vi "New Cobra GUI.vi"(8 "error in":errorcluster) -> (0 "Error Out":errorcluster)   [LabVIEW 2019, in "GUI.lvlib"]
doc: "New GUI 21.7.19"
uses:
  GUI.lvlib
  Controls/Main Waveform.ctl
  Controls/System Graphs.ctl
  Controls/Module Graphs.ctl
  Controls/Dial Gauges.ctl
  Controls/Gauge Graphs/Compression Ratio.ctl
  Controls/Gauge Graphs/Subcooling.ctl
  Controls/Gauge Graphs/Superheat.ctl
  Controls/Gauge Graphs/Current.ctl
  Controls/Module Key Values.ctl
  Controls/Event.ctl
  Controls/Messaging Actions.ctl
  Controls/New GUI Variables.ctl
  Controls/Network Data Down_set back.ctl
  Controls/NS New Data.ctl
  <vilib>/NI/STM/TCP/TCP Connection Info.ctl
  <vilib>/NI/STM/SubVIs/MetaDataElement.ctl
  Controls/Dataset_New.ctl
  Controls/System Status.ctl
  Controls/Module Status.ctl
  Controls/Config Data.ctl
  <vilib>/Utility/miscctls.llb/LVPositionTypeDef.ctl
  <vilib>/NI/STM/TCP/TCP Read Options.ctl
  Controls/WebDAV states.ctl
  <vilib>/Analysis/baseanly.llb/Mean (DBL).vi
  b9938fbe-5ccd-4e62-98e3-88d978d07e59.vi
  795e1a79-78c9-4e5b-9a6d-4827452a9509.vi
  894b418a-eb83-4c03-97c2-0273c02a970a.vi
  81edff22-585a-4beb-bf15-c06a681b6c24.vi
  <vilib>/NI/STM/TCP/Read Meta Data (TCP Ref).vi
  <vilib>/NI/STM/TCP/Get Connection Reference (TCP).vi
  <vilib>/NI/STM/TCP/Read Meta Data (TCP Clst).vi
  <vilib>/NI/STM/TCP/Read Message (TCP).vi
  <vilib>/NI/STM/TCP/Write Message (TCP).vi
  <vilib>/regexp/Match Regular Expression.xnode
  <vilib>/nisyscfg/nisyscfg.lvlib
  <resource>/objmgr/ni.dex.rc
  Controls/Save Log State.ctl
  <vilib>/Analysis/NI_AALBase.lvlib
  <vilib>/NI/STM/NI STM.lvlib
  <vilib>/addons/_JKI.lib/Serialization/JSON/JKI JSON Serialization.lvlib
panel:
  in  "Login":bool
  out "RT Version":string="Simulation Mode" caption="Cobra GUI Version :"
  in  "Shutdown":bool caption="Stop RT"
  in  "M1 Feedback":u8(ring)=1 caption="Enable" items=["Evap Temp", "Case Temp", "Intec Temp", "TSD  Temp", "Autotune", "Extra"]
  in  "M2 Feedback":u8(ring)=1 caption="Enable" items=["Evap Temp", "Case Temp", "Intec Temp", "TSD  Temp", "Autotune", "Extra"]
  out "M2 Data":T1={"Set Temp"=20.0, "Read Temp"=0.0, "Package"="", "Force"=0.0, "Feedback"=1} caption="M2 Status" {"Feedback" items=["Evap Temp", "Case Temp", "Intec Temp", "TSD  Temp", "Autotune", "Extra"]; "Force" format="%4.1f"; "Read Temp" format="%4.1f"; "Set Temp" format="%4.0f"}
  out "M1 Data":T1={"Set Temp"=25.0, "Read Temp"=24.578125, "Package"="new_chip", "Force"=0.0, "Feedback"=1} caption="M1 Status" {"Feedback" items=["Evap Temp", "Case Temp", "Intec Temp", "TSD  Temp", "Autotune", "Extra"]; "Force" format="%4.1f"; "Read Temp" format="%4.1f"; "Set Temp" format="%4.0f"}
  out "Comp":bool caption="System"
  out "Stack light states":T2(ring) caption="System Status"
  in  "Change TSD":bool
  out "TSD Data":T3={"TSD Millivolts"=nan, "X factor"=1.0, "Offset"=0.0, "TSD Temp"=nan, "TSD Feedback"=FALSE, "TSD Max"=225.0, "TSD Min"=-60.0}
  out "M1 AC Load V":dbl
  in  "Net Cluster":T4={"Menu Ring"=0, "System Ready"=TRUE, "Manual IP"="", "Refresh"=FALSE, "IP Override"=FALSE} {"Menu Ring" items=["DualCobra152 (192.168.2.52)", "Gen3Cobra146 (192.168.2.46)", "QC-Test (192.168.1.57)"]}
  out "AI (V)":dbl[](array[numeric])=[0.0, 0.0, 0.0, 0.0, 0.0, 0.0, 0.0, 0.0, 0.0, 0.0, 5.0, 5.0, 1625.0, 0.0, 0.0, 0.0, 0.0, 0.0, 0.0]
  out "data out":T5={"Condensing Pressure"=153.40193026626991, "Suction Pressure"=154.74626335545852, "Bypass steps"=0, "Operating Time"=0.0, "SubCooling"=-2.934594678017916, "Superheat"=3.7527707418295932, "M1 Superheat"=3.162141007730682, "M2 Superheat"=-40.92379649226932, "Autotune output"=0.0, "M1 Testing Elapsed Time"=0.0, "M2 Testing Elapsed Time"=0.0, "M1 Valve Control Mode"=0, "System Amps"=0.1457709610825283, "Compressor Run Time"=0.0, "SD card free Space"=31890.0, "Free Memory"=0.0, "M1 Pressure Feedback"=0.0, "M2 Pressure Feedback"=0.0, "Compression Ratio"=0.9920663161136312, "Serial Number"=0.0, "M1 AC Load V"=0.0, "M1 AC Load W"=nan, "M1 DC Load W"=0.0, "M1 RH"=33.76176771953824, "RH Threshold"=10.0}
  in  "Tab Control":T6(tab)=enum."Debug"
  out "M2 Safe Temp and Head State":bool
  out "M2 Bin String":string
  out "M2 PV":dbl caption="M2 Case Temp" format="%4.1f"
  in  "M2 Package":u16(ring)=4 items=["new_chip", "AI_chip", "CPU", "GPU", "Max Force", "", "", "", "", ""]
  in  "M2 Set Temp":dbl=20.0 min=-50.0 max=150.0 step=5.0 format="%#.1f"
  in  "M2 Commands Panel":T7={"M2 Enable"=TRUE, "M2 TSD Feedback"=FALSE}
  out "M1 Bin String":string
  in  "M1 Set Temp":dbl=25.0 min=-50.0 max=150.0 step=5.0 format="%#.1f"
  in  "M1 Package":u16(ring) items=["new_chip", "AI_chip", "CPU", "GPU", "Max Force", "", "", "", "", ""]
  out "M1 PV":dbl=24.578125 caption="M1 Case Temp" format="%4.1f"
  in  "M1 Commands Panel":T8={"M1 Enable"=TRUE, "M1 TSD Feedback"=FALSE}
  out "M1 Safe Temp and Head State":bool
  in  "M2 Power Drive Control":bool
  out "M1 Main Waveform":T9=[{"t0"=timestamp(3706115941.7064414 s since 1904-01-01), "dt"=1.0, "Y"=[25.0]}, {"t0"=timestamp(3706115941.7064414 s since 1904-01-01), "dt"=1.0, "Y"=[24.4453125]}, {"t0"=timestamp(3706115941.7064414 s since 1904-01-01), "dt"=1.0, "Y"=[24.578125]}, {"t0"=timestamp(3706115941.7064414 s since 1904-01-01), "dt"=1.0, "Y"=[nan]}, {"t0"=timestamp(3706115941.7064414 s since 1904-01-01), "dt"=1.0, "Y"=[nan]}]
  in  "M1 Power Drive Control":bool
  out "M2 Power Drive Indicator":bool caption="M2 Power Drive Control"
  out "M1 Power Drive Indicator":bool caption="M1 Power Drive Control"
  in  "Power On-Off":bool
  out "Play/Pause":bool
  out "M2 Main Waveform":T9=[{"t0"=timestamp(3706115941.7064414 s since 1904-01-01), "dt"=1.0, "Y"=[20.0]}, {"t0"=timestamp(3706115941.7064414 s since 1904-01-01), "dt"=1.0, "Y"=[0.0]}, {"t0"=timestamp(3706115941.7064414 s since 1904-01-01), "dt"=1.0, "Y"=[0.0]}, {"t0"=timestamp(3706115941.7064414 s since 1904-01-01), "dt"=1.0, "Y"=[0.0]}]
  out "M1 Channels":dbl[](array[numeric])=[25.0, 24.4453125, 24.578125, nan, nan, 0.0] format="%4.1f"
  out "M2 Channels":dbl[](array[numeric])=[20.0, 0.0, 0.0, 0.0, 0.0] format="%4.1f"
  out "M1 Humidity":cluster{"M1 RH":dbl, "RH Threshold":dbl}(graph)={"M1 RH"=10.0, "RH Threshold"=33.76176771953824}
  out "Low Side RPM":dbl
  out "High Side RPM":dbl
  out "M2 Thermal State":T10(ring)
  out "System Graphs":T11={"Ambient Temp"=75.93125465512276, "Suction Temp"=76.69062973558903, "Condensor Temp"=75.24219208210707, "Discharge Temp"=76.67656723409891, "Bypass Steps"=72.0}
  out "M1 Thermal State":T12(ring)=enum."Steady State"
  out "Gauges":T13={"Condensing Pressure(psi)"=153.40193026626991, "Compression Ratio"=0.9920663161136312, "Subcool"=-3.0617528737987953, "Superheat"=3.6858450233187767, "Current(A)"=0.1457709610825283, "Suction Pressure(psi)"=154.74626335545852} {"Suction Pressure(psi)" scale=0.0..100.0; "Current(A)" scale=5.0..15.0 scale format="%_1f"; "Superheat" scale=0.0..100.0; "Subcool" scale=-10.0..20.0 scale format="%#4.1f"; "Compression Ratio" scale=0.0..30.0 scale format="%#.0f"; "Condensing Pressure(psi)" scale=150.0..375.0}
  in  "Graph Tab CTL":enum32{"Head #1", "Head #2"}(tab)
  out "M1 Graphs":T18={"Case Temp"=24.578125, "Evap Temp"=24.4453125, "Heater Power (%)"=0.0, "EEV Steps"=0.0, "AC Load(W)"=0.0} caption="Head #1"
  out "M2 Graphs":T18 caption="Head #2"
  in  "Package":bool
  in  "Configure":bool
  out "Errors":string[](array[string])=["Warning: Air not plugged in  (21 06 08 14 08)"]
  in  "Event Tab":enum32{"Cobra Events", "GUI Events"}(tab)
  out "Event log":T19(array[cluster])=[{"Name"="Bypass Inintialized", "Time Stamp"=timestamp(3706031317.901618 s since 1904-01-01), "Code"="", "Source"="", "Value"=22160.0, "Boolean"=FALSE, "String"="Complete", "Error"=FALSE, "Warning"=FALSE, " Fault"=FALSE}, {"Name"="Timeserver not found", "Time Stamp"=timestamp(3706031309.741007 s since 1904-01-01), "Code"="", "Source"="SOM Time", "Value"=0.0, "Boolean"=FALSE, "String"="", "Error"=FALSE, "Warning"=FALSE, " Fault"=FALSE}, {"Name"="Bypass Target Change", "Time Stamp"=timestamp(3706031309.711301 s since 1904-01-01), "Code"="", "Source"="Bypass:Get Target", "Value"=110.0, "Boolean"=FALSE, "String"="", "Error"=FALSE, "Warning"=TRUE, " Fault"=FALSE}, {"Name"="Mains Frequency", "Time Stamp"=timestamp(3706031309.198055 s since 1904-01-01), "Code"="", "Source"="Init System Module", "Value"=59.9940002520096, "Boolean"=FALSE, "String"="", "Error"=FALSE, "Warning"=FALSE, " Fault"=FALSE}, {"Name"="PID Bypassed", "Time Stamp"=timestamp(3706031307.313306 s since 1904-01-01), "Code"="", "Source"="APP:Set/Send PID Bypass", "Value"=0.0, "Boolean"=FALSE, "String"="", "Error"=FALSE, "Warning"=FALSE, " Fault"=FALSE}, {"Name"="Thermal Status Change", "Time Stamp"=timestamp(3706031307.007236 s since 1904-01-01), "Code"="", "Source"="APP:Thermal Status", "Value"=0.0, "Boolean"=FALSE, "String"="", "Error"=FALSE, "Warning"=FALSE, " Fault"=FALSE}, {"Name"="Feedback Change", "Time Stamp"=timestamp(3706031306.793005 s since 1904-01-01), "Code"="", "Source"="APP:Get Feedback", "Value"=1.0, "Boolean"=FALSE, "String"="Case", "Error"=FALSE, "Warning"=FALSE, " Fault"=FALSE}, {"Name"="M1 Setpoint Change", "Time Stamp"=timestamp(3706031306.436291 s since 1904-01-01), "Code"="", "Source"="APP:Send Set Temp", "Value"=25.0, "Boolean"=FALSE, "String"="", "Error"=FALSE, "Warning"=TRUE, " Fault"=FALSE}, {"Name"="M1 Dynamic Set Point", "Time Stamp"=timestamp(3706031306.386277 s since 1904-01-01), "Code"="", "Source"="APP:Get Dynamic Set Temp", "Value"=25.0, "Boolean"=FALSE, "String"="", "Error"=FALSE, "Warning"=FALSE, " Fault"=FALSE}, {"Name"="M1 EEV Check Position", "Time Stamp"=timestamp(3706031306.325976 s since 1904-01-01), "Code"="", "Source"="", "Value"=0.0, "Boolean"=TRUE, "String"="Complete", "Error"=FALSE, "Warning"=FALSE, " Fault"=FALSE}, {"Name"="I2C TSD Freeze Timeout", "Time Stamp"=timestamp(3706031300.268274 s since 1904-01-01), "Code"="", "Source"="", "Value"=0.0, "Boolean"=FALSE, "String"="", "Error"=TRUE, "Warning"=FALSE, " Fault"=FALSE}, {"Name"="New Extra Settings Loaded", "Time Stamp"=timestamp(3706031298.435066 s since 1904-01-01), "Code"="", "Source"="", "Value"=0.0, "Boolean"=FALSE, "String"="", "Error"=FALSE, "Warning"=FALSE, " Fault"=FALSE}, {"Name"="Read Compressor Minutes", "Time Stamp"=timestamp(3706031298.210019 s since 1904-01-01), "Code"="", "Source"="", "Value"=0.0, "Boolean"=TRUE, "String"="PASS", "Error"=FALSE, "Warning"=FALSE, " Fault"=FALSE}, {"Name"="M1 EEV Check Position", "Time Stamp"=timestamp(3706031296.21211 s since 1904-01-01), "Code"="", "Source"="EEV:Check Position", "Value"=0.0, "Boolean"=FALSE, "String"="", "Error"=FALSE, "Warning"=FALSE, " Fault"=FALSE}, {"Name"="EEV PID Output", "Time Stamp"=timestamp(3706031296.161288 s since 1904-01-01), "Code"="", "Source"="APP:Send EEV PID Out", "Value"=0.0, "Boolean"=FALSE, "String"="Value Change", "Error"=FALSE, "Warning"=FALSE, " Fault"=FALSE}, {"Name"="", "Time Stamp"=timestamp(3706031296.053791 s since 1904-01-01), "Code"="", "Source"="EEV:Set Position", "Value"=0.0, "Boolean"=FALSE, "String"="", "Error"=FALSE, "Warning"=FALSE, " Fault"=FALSE}, {"Name"="", "Time Stamp"=timestamp(3706031296.000374 s since 1904-01-01), "Code"="", "Source"="EEV:Config", "Value"=0.0, "Boolean"=FALSE, "String"="", "Error"=FALSE, "Warning"=FALSE, " Fault"=FALSE}, {"Name"="M1 EEV Check Position", "Time Stamp"=timestamp(3706031294.611185 s since 1904-01-01), "Code"="", "Source"="", "Value"=2000.0, "Boolean"=TRUE, "String"="Complete", "Error"=FALSE, "Warning"=FALSE, " Fault"=FALSE}, {"Name"="M1 EEV Check Position", "Time Stamp"=timestamp(3706031294.000098 s since 1904-01-01), "Code"="", "Source"="EEV:Check Position", "Value"=0.0, "Boolean"=FALSE, "String"="", "Error"=FALSE, "Warning"=FALSE, " Fault"=FALSE}, {"Name"="EEV PID Output", "Time Stamp"=timestamp(3706031293.949764 s since 1904-01-01), "Code"="", "Source"="APP:Send EEV PID Out", "Value"=2000.0, "Boolean"=FALSE, "String"="Value Change", "Error"=FALSE, "Warning"=FALSE, " Fault"=FALSE}, {"Name"="", "Time Stamp"=timestamp(3706031293.848812 s since 1904-01-01), "Code"="", "Source"="EEV:Set Position", "Value"=0.0, "Boolean"=TRUE, "String"="", "Error"=FALSE, "Warning"=FALSE, " Fault"=FALSE}, {"Name"="EEV:Set V", "Time Stamp"=timestamp(3706031293.798386 s since 1904-01-01), "Code"="", "Source"="", "Value"=0.0, "Boolean"=FALSE, "String"="", "Error"=FALSE, "Warning"=FALSE, " Fault"=FALSE}, {"Name"="", "Time Stamp"=timestamp(3706031293.748195 s since 1904-01-01), "Code"="", "Source"="EEV:Config", "Value"=0.0, "Boolean"=FALSE, "String"="", "Error"=FALSE, "Warning"=FALSE, " Fault"=FALSE}, {"Name"="Config Loaded", "Time Stamp"=timestamp(3706031293.397414 s since 1904-01-01), "Code"="", "Source"="Config Read Initialize", "Value"=107.0, "Boolean"=FALSE, "String"="", "Error"=FALSE, "Warning"=FALSE, " Fault"=FALSE}, {"Name"="Config Read", "Time Stamp"=timestamp(3706031293.37065 s since 1904-01-01), "Code"="Found", "Source"="EEV PID", "Value"=25.0, "Boolean"=FALSE, "String"="", "Error"=FALSE, "Warning"=FALSE, " Fault"=FALSE}, {"Name"="Config Read", "Time Stamp"=timestamp(3706031293.359371 s since 1904-01-01), "Code"="Found", "Source"="Set Point Range", "Value"=-50.0, "Boolean"=FALSE, "String"="", "Error"=FALSE, "Warning"=FALSE, " Fault"=FALSE}, {"Name"="Config Value Read", "Time Stamp"=timestamp(3706031293.335439 s since 1904-01-01), "Code"="", "Source"="", "Value"=0.0, "Boolean"=TRUE, "String"="Cascade", "Error"=FALSE, "Warning"=FALSE, " Fault"=FALSE}, {"Name"="Config Value Read", "Time Stamp"=timestamp(3706031293.315639 s since 1904-01-01), "Code"="", "Source"="", "Value"=0.0, "Boolean"=TRUE, "String"="Sensors", "Error"=FALSE, "Warning"=FALSE, " Fault"=FALSE}, {"Name"="Read Saved State", "Time Stamp"=timestamp(3706031293.26891 s since 1904-01-01), "Code"="", "Source"="", "Value"=0.0, "Boolean"=FALSE, "String"="", "Error"=FALSE, "Warning"=FALSE, " Fault"=FALSE}, {"Name"="EMO Switch Detected", "Time Stamp"=timestamp(3706031293.21723 s since 1904-01-01), "Code"="", "Source"="", "Value"=0.0, "Boolean"=TRUE, "String"="", "Error"=FALSE, "Warning"=FALSE, " Fault"=FALSE}, {"Name"="Read Saved State", "Time Stamp"=timestamp(3706031293.183574 s since 1904-01-01), "Code"="", "Source"="", "Value"=0.0, "Boolean"=FALSE, "String"="", "Error"=FALSE, "Warning"=FALSE, " Fault"=FALSE}, {"Name"="FPGA Load Complete", "Time Stamp"=timestamp(3706031293.139812 s since 1904-01-01), "Code"="", "Source"="Init FPGA IO.vi", "Value"=0.0, "Boolean"=FALSE, "String"="", "Error"=FALSE, "Warning"=FALSE, " Fault"=FALSE}, {"Name"="Pressure Test", "Time Stamp"=timestamp(3706031291.136962 s since 1904-01-01), "Code"="", "Source"="Init FPGA IO 2.0.vi", "Value"=0.00022888532845044633, "Boolean"=FALSE, "String"="FAIL", "Error"=FALSE, "Warning"=TRUE, " Fault"=FALSE}, {"Name"="Stop LCD", "Time Stamp"=timestamp(3706031285.92111 s since 1904-01-01), "Code"="", "Source"="Init FPGA IO.vi", "Value"=11.0, "Boolean"=FALSE, "String"="", "Error"=FALSE, "Warning"=FALSE, " Fault"=FALSE}, {"Name"="wait", "Time Stamp"=timestamp(3706031284.919174 s since 1904-01-01), "Code"="", "Source"="Init FPGA IO.vi", "Value"=10.0, "Boolean"=FALSE, "String"="", "Error"=FALSE, "Warning"=FALSE, " Fault"=FALSE}, {"Name"="IP Address", "Time Stamp"=timestamp(3706031283.915648 s since 1904-01-01), "Code"="", "Source"="Init FPGA IO.vi", "Value"=12.0, "Boolean"=FALSE, "String"="þQ", "Error"=FALSE, "Warning"=FALSE, " Fault"=FALSE}, {"Name"="wait", "Time Stamp"=timestamp(3706031283.836404 s since 1904-01-01), "Code"="", "Source"="Init FPGA IO.vi", "Value"=10.0, "Boolean"=FALSE, "String"="", "Error"=FALSE, "Warning"=FALSE, " Fault"=FALSE}, {"Name"="Rev Display", "Time Stamp"=timestamp(3706031282.833974 s since 1904-01-01), "Code"="", "Source"="Init FPGA IO.vi", "Value"=9.0, "Boolean"=FALSE, "String"="Ver: CC 21.6.1.0", "Error"=FALSE, "Warning"=FALSE, " Fault"=FALSE}, {"Name"="wait", "Time Stamp"=timestamp(3706031282.765893 s since 1904-01-01), "Code"="", "Source"="Init FPGA IO.vi", "Value"=10.0, "Boolean"=FALSE, "String"="", "Error"=FALSE, "Warning"=FALSE, " Fault"=FALSE}, {"Name"="Chroma Display", "Time Stamp"=timestamp(3706031281.763213 s since 1904-01-01), "Code"="", "Source"="Init FPGA IO.vi", "Value"=8.0, "Boolean"=FALSE, "String"="Chroma ATE", "Error"=FALSE, "Warning"=FALSE, " Fault"=FALSE}, {"Name"="wait", "Time Stamp"=timestamp(3706031281.696552 s since 1904-01-01), "Code"="", "Source"="Init FPGA IO.vi", "Value"=10.0, "Boolean"=FALSE, "String"="", "Error"=FALSE, "Warning"=FALSE, " Fault"=FALSE}, {"Name"="Clear LCD Text", "Time Stamp"=timestamp(3706031280.693969 s since 1904-01-01), "Code"="", "Source"="Init FPGA IO.vi", "Value"=0.0, "Boolean"=FALSE, "String"="", "Error"=FALSE, "Warning"=FALSE, " Fault"=FALSE}, {"Name"="BootLoad", "Time Stamp"=timestamp(3706031279.648552 s since 1904-01-01), "Code"="", "Source"="Init FPGA IO.vi", "Value"=0.0, "Boolean"=FALSE, "String"="", "Error"=FALSE, "Warning"=FALSE, " Fault"=FALSE}, {"Name"="Extra Settings Loaded", "Time Stamp"=timestamp(3706031277.495041 s since 1904-01-01), "Code"="", "Source"="", "Value"=0.0, "Boolean"=FALSE, "String"="", "Error"=FALSE, "Warning"=FALSE, " Fault"=FALSE}, {"Name"="Warmup ", "Time Stamp"=timestamp(3706031277.461598 s since 1904-01-01), "Code"="", "Source"="Extra Settings", "Value"=0.0, "Boolean"=FALSE, "String"="", "Error"=FALSE, "Warning"=TRUE, " Fault"=FALSE}, {"Name"="Flow Curve", "Time Stamp"=timestamp(3706031277.436586 s since 1904-01-01), "Code"="", "Source"="Extra Settings", "Value"=0.0, "Boolean"=FALSE, "String"="", "Error"=FALSE, "Warning"=TRUE, " Fault"=FALSE}, {"Name"="Relative Humidity", "Time Stamp"=timestamp(3706031277.408702 s since 1904-01-01), "Code"="", "Source"="Extra Settings", "Value"=0.0, "Boolean"=TRUE, "String"="", "Error"=FALSE, "Warning"=FALSE, " Fault"=FALSE}, {"Name"="Warnings/Faults 1", "Time Stamp"=timestamp(3706031277.370367 s since 1904-01-01), "Code"="", "Source"="Extra Settings 3", "Value"=0.0, "Boolean"=TRUE, "String"="", "Error"=FALSE, "Warning"=FALSE, " Fault"=FALSE}, {"Name"="SuperHeat Settings", "Time Stamp"=timestamp(3706031277.356517 s since 1904-01-01), "Code"="", "Source"="Extra Settings 3", "Value"=0.0, "Boolean"=TRUE, "String"="", "Error"=FALSE, "Warning"=FALSE, " Fault"=FALSE}, {"Name"="Config Loaded", "Time Stamp"=timestamp(3706031277.313113 s since 1904-01-01), "Code"="", "Source"="Config Read Initialize", "Value"=74.0, "Boolean"=FALSE, "String"="", "Error"=FALSE, "Warning"=FALSE, " Fault"=FALSE}, {"Name"="Config Read", "Time Stamp"=timestamp(3706031277.287857 s since 1904-01-01), "Code"="Found", "Source"="M2 Heater PID", "Value"=0.0, "Boolean"=FALSE, "String"="", "Error"=FALSE, "Warning"=FALSE, " Fault"=FALSE}, {"Name"="Config Value Read", "Time Stamp"=timestamp(3706031277.269987 s since 1904-01-01), "Code"="", "Source"="", "Value"=0.0, "Boolean"=TRUE, "String"="Handler", "Error"=FALSE, "Warning"=FALSE, " Fault"=FALSE}] {"Value" format="%4.1f"; "Time Stamp" format="%<%x %.3X>T"}
  out "GUI Events":T20[](array[typedef])=[{"Name"="NS:Open Connection", "Time Stamp"=timestamp(3706444762.0143776 s since 1904-01-01), "Code"=-1950678953, "Source"="Create Network Stream Reader Endpoint in GUI.lvlib:New Cobra GUI.vi", "Value"="", "Boolean"=FALSE, "Description"="", "Error"=TRUE, "Warning"=FALSE, " Fault"=FALSE}, {"Name"="NS:Open Connection", "Time Stamp"=timestamp(3706444762.0213585 s since 1904-01-01), "Code"=-1950678953, "Source"="Create Network Stream Reader Endpoint in GUI.lvlib:New Cobra GUI.vi", "Value"="", "Boolean"=FALSE, "Description"="", "Error"=TRUE, "Warning"=FALSE, " Fault"=FALSE}, {"Name"="Idle", "Time Stamp"=timestamp(3706444762.122089 s since 1904-01-01), "Code"=0, "Source"="", "Value"="", "Boolean"=FALSE, "Description"="Start Cobra GUI", "Error"=FALSE, "Warning"=FALSE, " Fault"=FALSE}, {"Name"="UI:Module Enable", "Time Stamp"=timestamp(3706444762.1230865 s since 1904-01-01), "Code"=0, "Source"="", "Value"="", "Boolean"=TRUE, "Description"="System Ready", "Error"=FALSE, "Warning"=FALSE, " Fault"=FALSE}] {"Time Stamp" format="%<%x %.3X>T"}
  in  "Datalog":bool
  in  "Reboot RT":bool
  out "M2 Buffer":dbl(slide)=2.0 scale=-4.0..4.0
  out "M2 Valve Output":dbl(knob) scale=0.0..100.0
  in  "Y-scale":bool
  out "Boot Up Time":timestamp=timestamp(3706031293.185896 s since 1904-01-01)
  out "M2 Heater %":dbl format="%3.0f"
  out "M2 Error":bool
  out "M2 Actuated":bool
  out "M2 Head State":enum16{"Disabled", "Run", "Error"}(ring)=enum."Run"
  out "M2 Thermal Status":T12(ring)
  in  "M2 EEV Manual":u16
  in  "M2 Heater Output":dbl
  in  "M1 EEV Manual":u16
  in  "Manual Bypass Mode":bool[](array[boolean])
  in  "M1 Heater output":dbl
  out "M1 Valve Output":dbl(knob) scale=0.0..100.0
  out "M1 Buffer":dbl(slide) scale=-4.0..4.0
  out "Detected Systems":string[](array[string])
  out "Data Rx Timestamp":timestamp=timestamp(3706107700.479949 s since 1904-01-01)
  out "M1 Superheat":dbl=3.162141007730682 format="%#.1f"
  out "M1 Testing Elapsed Time":dbl caption="Test Elapsed Time" format="%<%H:%M:%S>t"
  out "TCP Connections":T21(array[cluster])=[{"port "=1300, "remote address"="", "Connection timeout ms"=100, "Waiting for connection"=TRUE, "Waiting for Command"=FALSE, "timeout ms"=5000}, {"port "=1100, "remote address"="", "Connection timeout ms"=100, "Waiting for connection"=TRUE, "Waiting for Command"=FALSE, "timeout ms"=-1}, {"port "=1000, "remote address"="", "Connection timeout ms"=100, "Waiting for connection"=TRUE, "Waiting for Command"=FALSE, "timeout ms"=60000}, {"port "=1001, "remote address"="", "Connection timeout ms"=100, "Waiting for connection"=TRUE, "Waiting for Command"=FALSE, "timeout ms"=60000}, {"port "=2100, "remote address"="", "Connection timeout ms"=100, "Waiting for connection"=FALSE, "Waiting for Command"=FALSE, "timeout ms"=-1}, {"port "=2001, "remote address"="", "Connection timeout ms"=100, "Waiting for connection"=FALSE, "Waiting for Command"=FALSE, "timeout ms"=60000}, {"port "=2000, "remote address"="", "Connection timeout ms"=100, "Waiting for connection"=FALSE, "Waiting for Command"=FALSE, "timeout ms"=5000}]
  out "Error":string[](array[string])=["Warning: Air not plugged in  (21 06 08 14 08)"]
  in  "Cascade Compressor controls":T22 {"Manual Low Stage frequency" min=40.0 max=150.0 step=1.0; "Manual High stage frequency" min=50.0 max=150.0 step=1.0}
  out "TCP commands":string[](array[string])
  out "M1 Head State":enum16{"Disabled", "Run", "Error"}(ring)=enum."Run"
  out "M1 Thermal Status":T12(ring)=enum."Steady State"
  out "M1 Error":bool
  out "M1 Actuated":bool
  out "M1 Heater %":dbl format="%3.0f"
  out "Sleep":bool=TRUE
  out "Sleep Timer":dbl
  out "Comp Temp":dbl=76.67656723409891 format="%#.1f"
  out "SOM":T23={"Software Version"="SW Version:CC 21.6.1.0", "CPU Usage"=99.04899711963543, "Memory Available"=317.184, "SOM Storage(MB)"=234.236, "SD card free space"=27.598} caption="System of Module" {"SD card free space" format="%#4.1f"; "CPU Usage" format="%#.1f"; "Memory Available" format="%#4.1f"; "SOM Storage(MB)" format="%4.1f"}
  out "Compressor Hours":dbl caption="Comp hrs" format="%#.1f"
  out "Serial Number":string="203800057"
  in  "Graph Temp Unit":bool
  in  "Average Graph":bool
  in  "Fixed Y-Range":dbl=4.0
  in  "Login TO":i32=10 caption="Login Timeout(min)" min=-1 max=1000
  in  "Real Mode":bool=TRUE
  # "System Module"
  # "M1 Module"
  # "M2 Module"
  # "Tuning"
  # "Manual Controls"
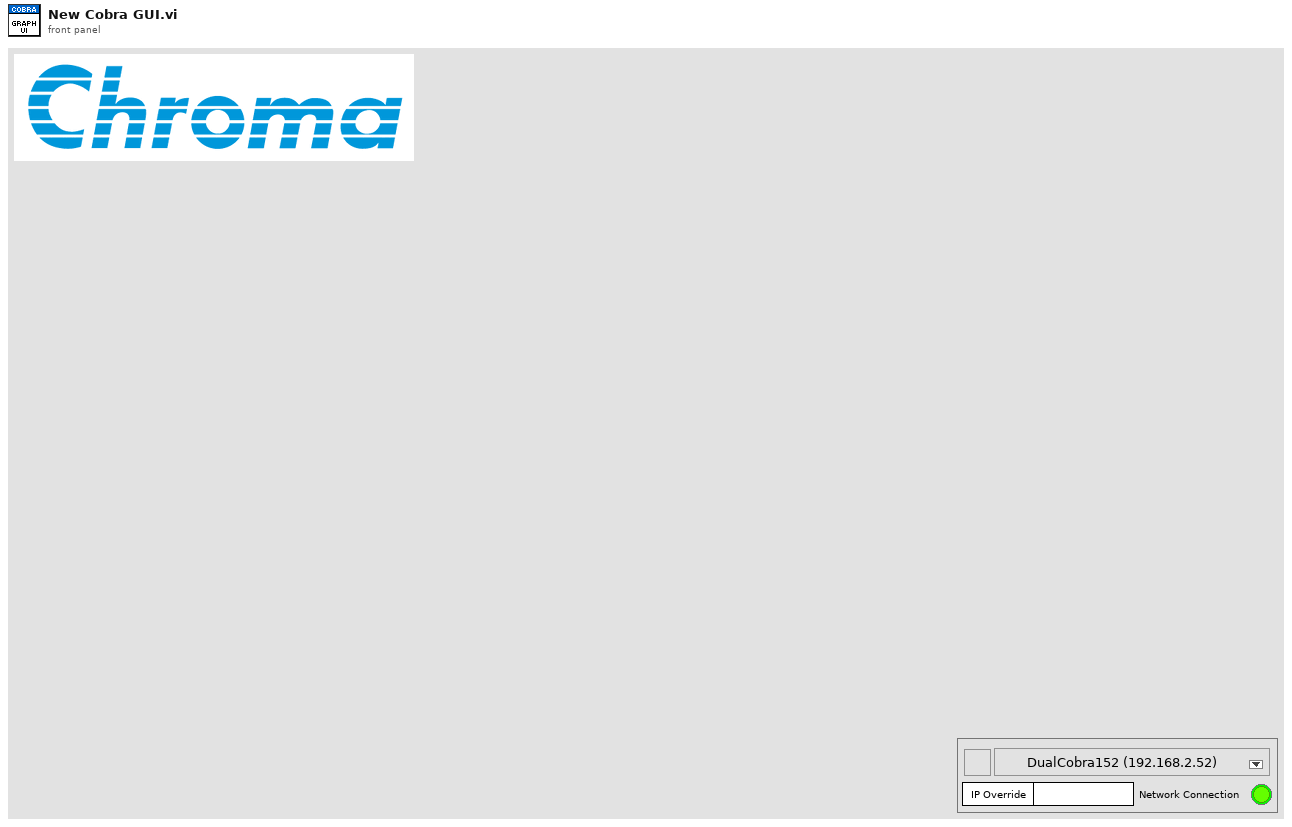
[diagram p1: front panel]
types:
  T1 = typedef "GUI.lvlib/Module Key Values.ctl" = cluster{"Set Temp":dbl, "Read Temp":dbl, "Package":string, "Force":dbl, "Feedback":u8}
  T2 = enum16{"Sleeping", "Warming up", "Ready", "Testing", "Restless", "Idle", "Sleeping Fault", "warning"}
  T3 = cluster{"TSD Millivolts":dbl, "X factor":dbl, "Offset":dbl, "TSD Temp":dbl, "TSD Feedback":bool, "TSD Max":dbl, "TSD Min":dbl}
  T4 = cluster{"Menu Ring":u16, "System Ready":bool, "Manual IP":string, "Refresh":bool, "IP Override":bool}
  T5 = cluster{"Condensing Pressure":dbl, "Suction Pressure":dbl, "Bypass steps":u16, "Operating Time":dbl, "SubCooling":dbl, "Superheat":dbl, "M1 Superheat":dbl, "M2 Superheat":dbl, "Autotune output":dbl, "M1 Testing Elapsed Time":dbl, "M2 Testing Elapsed Time":dbl, "M1 Valve Control Mode":u8, "System Amps":dbl, "Compressor Run Time":dbl, "SD card free Space":dbl, "Free Memory":dbl, "M1 Pressure Feedback":dbl, "M2 Pressure Feedback":dbl, "Compression Ratio":dbl, "Serial Number":dbl, "M1 AC Load V":dbl, "M1 AC Load W":dbl, "M1 DC Load W":dbl, "M1 RH":dbl, "RH Threshold":dbl}
  T6 = enum32{"Controls", "Graphs", "Settings", "Debug", "TEST"}
  T7 = cluster{"M2 Enable":bool, "M2 TSD Feedback":bool}
  T8 = cluster{"M1 Enable":bool, "M1 TSD Feedback":bool}
  T9 = typedef "GUI.lvlib/Main Waveform.ctl" = waveform(dbl)[]
  T10 = enum16{"Ramp Up", "Ramp Down", "Steady State", "Ebb and Flow", "Up", "Under Load", "Cryo Mode", "Shuttle Mode"}
  T11 = typedef "GUI.lvlib/System Graphs.ctl" = cluster{"Ambient Temp":dbl, "Suction Temp":dbl, "Condensor Temp":dbl, "Discharge Temp":dbl, "Bypass Steps":dbl}
  T12 = enum16{"Ramp Up", "Ramp Down", "Steady State", "Ebb and Flow", "Up", "Under Load", "Cryo Mode"}
  T13 = typedef "GUI.lvlib/Dial Gauges.ctl" = cluster{"Condensing Pressure(psi)":dbl, "Compression Ratio":T14, "Subcool":T15, "Superheat":T16, "Current(A)":T17, "Suction Pressure(psi)":dbl}
  T14 = typedef "GUI.lvlib/Compression Ratio.ctl" = dbl
  T15 = typedef "GUI.lvlib/Subcooling.ctl" = dbl
  T16 = typedef "GUI.lvlib/Superheat.ctl" = dbl
  T17 = typedef "GUI.lvlib/Current.ctl" = dbl
  T18 = typedef "GUI.lvlib/Module Graphs.ctl" = cluster{"Case Temp":dbl, "Evap Temp":dbl, "Heater Power (%)":dbl, "EEV Steps":dbl, "AC Load(W)":dbl}
  T19 = cluster{"Name":string, "Time Stamp":timestamp, "Code":string, "Source":string, "Value":dbl, "Boolean":bool, "String":string, "Error":bool, "Warning":bool, " Fault":bool}[]
  T20 = typedef "GUI.lvlib/Event.ctl" = cluster{"Name":string, "Time Stamp":timestamp, "Code":i32, "Source":string, "Value":string, "Boolean":bool, "Description":string, "Error":bool, "Warning":bool, " Fault":bool}
  T21 = cluster{"port ":u16, "remote address":string, "Connection timeout ms":i32, "Waiting for connection":bool, "Waiting for Command":bool, "timeout ms":i32}[]
  T22 = cluster{"High Stage manual speed control":bool, "Manual High stage frequency":dbl, "Low Stage manual speed control":bool, "Manual Low Stage frequency":dbl}
  T23 = cluster{"Software Version":string, "CPU Usage":dbl, "Memory Available":dbl, "SOM Storage(MB)":dbl, "SD card free space":dbl}
  T24 = typedef "GUI.lvlib/New GUI Variables.ctl" = cluster{"Core":cluster{"Current VI":refnum<vi>, "Close Panel on Exit?":bool, "VI Name":string, "VI Path":path}, "reader endpoint":refnum<k21>, "writer endpoint":refnum<k21>, "Detected Systems":string[], "IP Address":string, "Network Connection":bool, "M1 History Temps":dbl[][], "M2 History Temps":dbl[][], "System Ready":bool, "M2 Bootup":bool, "Network Data Down":T25, "Event Log":T20[], "Connected System":string, "TCP connection info":T27, "TCP Connection":bool, "Dataset":T29, "Real Mode":bool, "Last Connected System":enum16{"Single Head", "Duel Head"}, "Reboot":bool, "Test":bool, "User":enum16{"Supervisor", "Engineer", "Operator", "Guest"}}
  T25 = typedef "GUI.lvlib/Network Data Down_set back.ctl" = cluster{"M1 Commands":cluster{"Set Temp":dbl, "Power Drive":bool, "Feedback":u8, "Package":u16, "Enable":bool}, "M2 Commands":cluster{"Set Temp":dbl, "Power Drive":bool, "Feedback":u8, "Package ":u16, "Enable":bool}, "Config Data":cluster{"Packages":cluster{"DUT Force lbf":cluster{" 0":u32, " 1":u32, " 2":u32, "3":u32, "4":u32, "5":u32, " 6":u32, "7":u32, "8":u32, "9":u32}, "DUT Names":cluster{"0":string, "1":string, "2":string, "3":string, "4":string, "5":string, "6":string, "7":string, "8":string, "9":string}}, "Heater PID":cluster{"P":dbl, "I":dbl, "D":dbl}, "Piston Settings":cluster{"Forces Slope":dbl, "Forces Intercept":dbl, "Transition Force":dbl, "Up Force":dbl, "Diameter (mm)":dbl, "Delay (ms)":dbl, "Pressure Ramp Delay (ms)":dbl}, "Safe Temps":cluster{"Minimum":i32, "Enabled":bool, "Maximum":i32}, "System Settings":cluster{"Number of Heads":i32, "60Hz Power":bool, "FTC200":bool, "AutoStartup":bool, "Purge":bool, "Sensors":bool, "HandClamp":bool, "ATE":bool, "Benchtop":bool, "Production":bool, "Refrigerant":enum16{"r404a", "r507", "r508", "r410a", "r134a"}, "Handler":bool, "Shuttle":bool, "220V":bool, "Cascade":bool, "Suction Sensor":enum16{"YCQB02H01", "YCQB02L01", "Carel"}, "Discharge Sensor":enum16{"YCQB05H01", "YCQB05L01", "Carel"}}, "Stepper Settings ":cluster{"Microstepping":enum16{"Full", "Half", "Quarter", "1/16th"}, "Velocity":u8}, "Set Point Range":cluster{"Max":dbl, "Min":dbl}, "Pedestal Check DeltaT":dbl, "Ramp Delta T":dbl, "Ramp-SS Threshold":dbl, "SS Tolerance":dbl, "EEV PID":cluster{"Ramp Up Target":dbl, "Ramp Down Target":dbl, "Steady State Target":dbl, "Output":cluster{"Max":dbl, "Min":dbl}, "EBB and Flow Temp TH":dbl, "Cryomode EEV Max":dbl, "Valve minimum opening ":dbl, "Ramp Up EEV Steps":dbl, "Ramp Down EEV Steps":dbl, "SS EEV Steps Reset":dbl, "EBB and Flow Tol":dbl, "Gains":cluster{"P":dbl, "I":dbl, "D":dbl}, "Dissabled Target":dbl, "CryoMode Gains":cluster{"P":dbl, "I":dbl, "D":dbl}, "M1 SuperHeat Setpoint":dbl, "M2 Gains":cluster{"P":dbl, "I":dbl, "D":dbl}, "Flow Curve":enum16{""}}, "Sleep Timeout":dbl, "Bypass Values":cluster{"Bypass Valve":bool, "Flow Curve":enum16{"0", "1"}, "Output":cluster{"Max":u32, "Min":u32}, "Feedback":enum16{"Temperature", "Pressure", "Superheat", "Pressure 2.0"}, "Cyth Bypass":bool, "PID":cluster{"P":dbl, "I":dbl, "D":dbl}, "Pressure setpoint":i16, "Cryo Temp":i16, "Superheat Setpoint":i16, "Cryo Setpoint":i16}, "Default Temp":dbl, "InTEC":cluster{"Enabled":bool, "IP":string, "Port":u16}, "M1 TSD":cluster{"Gain":dbl, "Offset":dbl, "V Offset ":dbl}, "M2 TSD":cluster{"Gain":dbl, "Offset":dbl, "V Offset ":dbl}, "M1 T-Case Calibration":cluster{"Gain":dbl, "Offset":dbl}, "M2 T-Case Calibration":cluster{"Gain":dbl, "Offset":dbl}, "Heater PID TSD":cluster{"P":dbl, "I":dbl, "D":dbl}, "M2 Heater PID":cluster{"P":dbl, "I":dbl, "D":dbl}}, "System Power On Off":bool, "New Data":T26, "Stop RT":bool}
  T26 = typedef "GUI.lvlib/NS New Data.ctl" = enum16{"M1 Set Point", "M1 Power Drive", "M1 Feedback", "M1 Package", "M1 Enable", "M2 Set Point", "M2 Power Drive", "M2 Feedback", "M2 Package", "M2 Enable", "System Power", "Config Data", "Stop RT"}
  T27 = typedef "NI STM.lvlib/TCP Connection Info.ctl" = cluster{"connection ID":refnum<k5>, "meta data":T28[]}
  T28 = typedef "NI STM.lvlib/MetaDataElement.ctl" = string
  T29 = typedef "GUI.lvlib/Dataset_New.ctl" = cluster{"System Status":T30, "M1 Status":T31, "M2 Status":T31, "Config Data":T32}
  T30 = typedef "GUI.lvlib/System Status.ctl" = cluster{"Power On Off":bool, "Discharge Temp":dbl, "Liquid Temp":dbl, "Suction Temp":dbl, "Ambient Temp":dbl, "Sleep":bool, "System Status":u16, "M1 Actuated":bool, "M2 Actuated":bool, "Sleep Timer":dbl, "M1 Bin":cluster{"Bin String":string, "Bin Color":u16}, "M2 Bin":cluster{"Bin String":string, "Bin Color":u16}, "Discharge Pressure":dbl, "Suction Pressure":dbl, "Compression Ratio":dbl, "Compressor Amps":dbl, "Compressor Hours":dbl, "Bypass Steps":u16, "SubCooling":dbl, "SuperHeat":dbl, "Serial Number":string, "EMO detected":bool, "EMO Tripped":bool, "Thermal cutoff":bool, "Thermal cutoff 2":bool, "High Pressure switch":bool, "Running Time":timestamp, "SOM Status":cluster{"Boot Up Time":timestamp, "Software Version":string, "CPU Usage":dbl, "Memory Available":dbl, "SD card free space":dbl, "SOM Storage":dbl}, "Cascade Extra":cluster{"Discharge Temp High Side":dbl, "Suction Temp High Side":dbl, "Liquid Temp High side":dbl, "Discharge Pressure 2":dbl, "Suction Pressure 2":dbl, "Low Side RPM":dbl, "High Side RPM":dbl}}
  T31 = typedef "GUI.lvlib/Module Status.ctl" = cluster{"Case Temp":dbl, "Evap Temp":dbl, "Heater %":dbl, "EEV Steps":u32, "Set Temp":dbl, "Feedback":u8, "Power Drive":bool, "Piston Volts":dbl, "Safe Temp":bool, "Power":bool, "Thermal State":u16, "Error":bool, "In tollerance":bool, "Head State":u16, "Piston Force":dbl, "Package":string, "Dynamic SV":dbl, "PV":dbl, "TSD Temp":dbl, "AC Load Watts":dbl, "DC Load Watts":dbl, "Intec Feedback":dbl}
  T32 = typedef "GUI.lvlib/Config Data.ctl" = cluster{"Packages":cluster{"DUT Force lbf":cluster{" 0":u32, " 1":u32, " 2":u32, "3":u32, "4":u32, "5":u32, " 6":u32, "7":u32, "8":u32, "9":u32}, "DUT Names":cluster{"0":string, "1":string, "2":string, "3":string, "4":string, "5":string, "6":string, "7":string, "8":string, "9":string}}, "Heater PID":cluster{"P":dbl, "I":dbl, "D":dbl}, "Piston Settings":cluster{"Forces Slope":dbl, "Forces Intercept":dbl, "Transition Force":dbl, "Up Force":dbl, "Diameter (mm)":dbl, "Delay (ms)":dbl, "Pressure Ramp Delay (ms)":dbl}, "Safe Temps":cluster{"Minimum":i32, "Enabled":bool, "Maximum":i32}, "System Settings":cluster{"Number of Heads":i32, "60Hz Power":bool, "FTC200":bool, "AutoStartup":bool, "Purge":bool, "Sensors":bool, "HandClamp":bool, "ATE":bool, "Benchtop":bool, "Production":bool, "Refrigerant":u16, "Handler":bool, "Shuttle":bool, "220V":bool, "Cascade":bool, "Suction Sensor":u16, "Discharge Sensor":u16}, "Stepper Settings ":cluster{"Microstepping":u16, "Velocity":u8}, "Set Point Range":cluster{"Max":dbl, "Min":dbl}, "Pedestal Check DeltaT":dbl, "Ramp Delta T":dbl, "Ramp-SS Threshold":dbl, "SS Tolerance":dbl, "EEV PID":cluster{"Ramp Up Target":dbl, "Ramp Down Target":dbl, "Steady State Target":dbl, "Output":cluster{"Max":dbl, "Min":dbl}, "EBB and Flow Temp TH":dbl, "Cryomode EEV Max":dbl, "Valve minimum opening ":dbl, "Ramp Up EEV Steps":dbl, "Ramp Down EEV Steps":dbl, "SS EEV Steps Reset":dbl, "EBB and Flow Tol":dbl, "Gains":cluster{"P":dbl, "I":dbl, "D":dbl}, "Dissabled Target":dbl, "CryoMode Gains":cluster{"P":dbl, "I":dbl, "D":dbl}, "M1 SuperHeat Setpoint":dbl, "M2 Gains":cluster{"P":dbl, "I":dbl, "D":dbl}, "Flow Curve":u16}, "Sleep Timeout":dbl, "Bypass Values":cluster{"Bypass Valve":bool, "Flow Curve":u16, "Output":cluster{"Max":u32, "Min":u32}, "Feedback":u16, "Cyth Bypass":bool, "PID":cluster{"P":dbl, "I":dbl, "D":dbl}, "Pressure setpoint":i16, "Cryo Temp":i16, "Superheat Setpoint":i16, "Cryo Setpoint":i16}, "Default Temp":dbl, "InTEC":cluster{"Enabled":bool, "IP":string, "Port":u16}, "M1 TSD":cluster{"Gain":dbl, "Offset":dbl, "V Offset ":dbl}, "M2 TSD":cluster{"Gain":dbl, "Offset":dbl, "V Offset ":dbl}, "M1 T-Case Calibration":cluster{"Gain":dbl, "Offset":dbl}, "M2 T-Case Calibration":cluster{"Gain":dbl, "Offset":dbl}, "Heater PID TSD":cluster{"P":dbl, "I":dbl, "D":dbl}, "M2 Heater PID":cluster{"P":dbl, "I":dbl, "D":dbl}}
  T33 = typedef "GUI.lvlib/Messaging Actions.ctl" = enum16{"Create", "Get", "Destroy"}
  T34 = typedef "GUI.lvlib/Save Log State.ctl" = enum16{"Idle", "Init", "Write", "Exit"}
  T35 = enum32{"Invalid", "Standard", "Closed", "Hidden", "Minimized", "Maximized"}
  T36 = enum8{"Enabled", "Disabled", "Disabled and Grayed Out"}
  T37 = enum32{"Page Enabled", "Page Disabled", "Page Disabled & Grayed"}
  T38 = enum16{"Supervisor", "Engineer", "Operator", "Guest"}
  T39 = typedef "LVPositionTypeDef.ctl" = cluster{"Left":i32, "Top":i32}
  T40 = cluster{"Set Temp":dbl, "Power Drive":bool, "Feedback":u8, "Package":u16, "Enable":bool}
  T41 = typedef "NI STM.lvlib/TCP Read Options.ctl" = cluster{"ignore timeout error":bool, "timeout ms (1000)":i32}
  T42 = typedef "GUI.lvlib/WebDAV states.ctl" = enum16{"Open Sess", "Refresh Dir", "Create Dir", "Upload", "Download", "Delete", "Close Sess"}
  T43 = cluster{"Boot Up Time":timestamp, "Software Version":string, "CPU Usage":dbl, "Memory Available":dbl, "SD card free space":dbl, "SOM Storage":dbl}
  T44 = cluster{"0":string, "1":string, "2":string, "3":string, "4":string, "5":string, "6":string, "7":string, "8":string, "9":string}
  T45 = cluster{"Power On Off":bool, "Discharge Temp":dbl, "Liquid Temp":dbl, "Suction Temp":dbl, "Ambient Temp":dbl, "Sleep":bool, "System Status":u16, "M1 Actuated":bool, "M2 Actuated":bool, "Sleep Timer":dbl, "M1 Bin":cluster{"Bin String":string, "Bin Color":u16}, "M2 Bin":cluster{"Bin String":string, "Bin Color":u16}, "Discharge Pressure":dbl, "Suction Pressure":dbl, "Compression Ratio":dbl, "Compressor Amps":dbl, "Compressor Hours":dbl, "Bypass Steps":u16, "SubCooling":dbl, "SuperHeat":dbl, "Serial Number":string, "EMO detected":bool, "EMO Tripped":bool, "Thermal cutoff":bool, "Thermal cutoff 2":bool, "High Pressure switch":bool, "Running Time":string, "SOM Status":cluster{"Boot Up Time":string, "Software Version":string, "CPU Usage":dbl, "Memory Available":dbl, "SD card free space":dbl, "SOM Storage":dbl}, "Cascade Extra":cluster{"Discharge Temp High Side":dbl, "Suction Temp High Side":dbl, "Liquid Temp High side":dbl, "Discharge Pressure 2":dbl, "Suction Pressure 2":dbl, "Low Side RPM":dbl, "High Side RPM":dbl}}
  T46 = cluster{"DUT Force lbf":cluster{" 0":u32, " 1":u32, " 2":u32, "3":u32, "4":u32, "5":u32, " 6":u32, "7":u32, "8":u32, "9":u32}, "DUT Names":cluster{"0":string, "1":string, "2":string, "3":string, "4":string, "5":string, "6":string, "7":string, "8":string, "9":string}}
  T47 = cluster{"Force - pounds":cluster{" 0":u32, " 1":u32, " 2":u32, "3":u32, "4":u32, "5":u32, " 6":u32, "7":u32, "8":u32, "9":u32}, "DUT Names":cluster{"0":string, "1":string, "2":string, "3":string, "4":string, "5":string, "6":string, "7":string, "8":string, "9":string}}
  T48 = typedef "NI_WebDAV.lvlib/FileInfo.ctl" = cluster{"type":string, "size":u64, "last modification":timestamp, "display name":string, "uri":string}
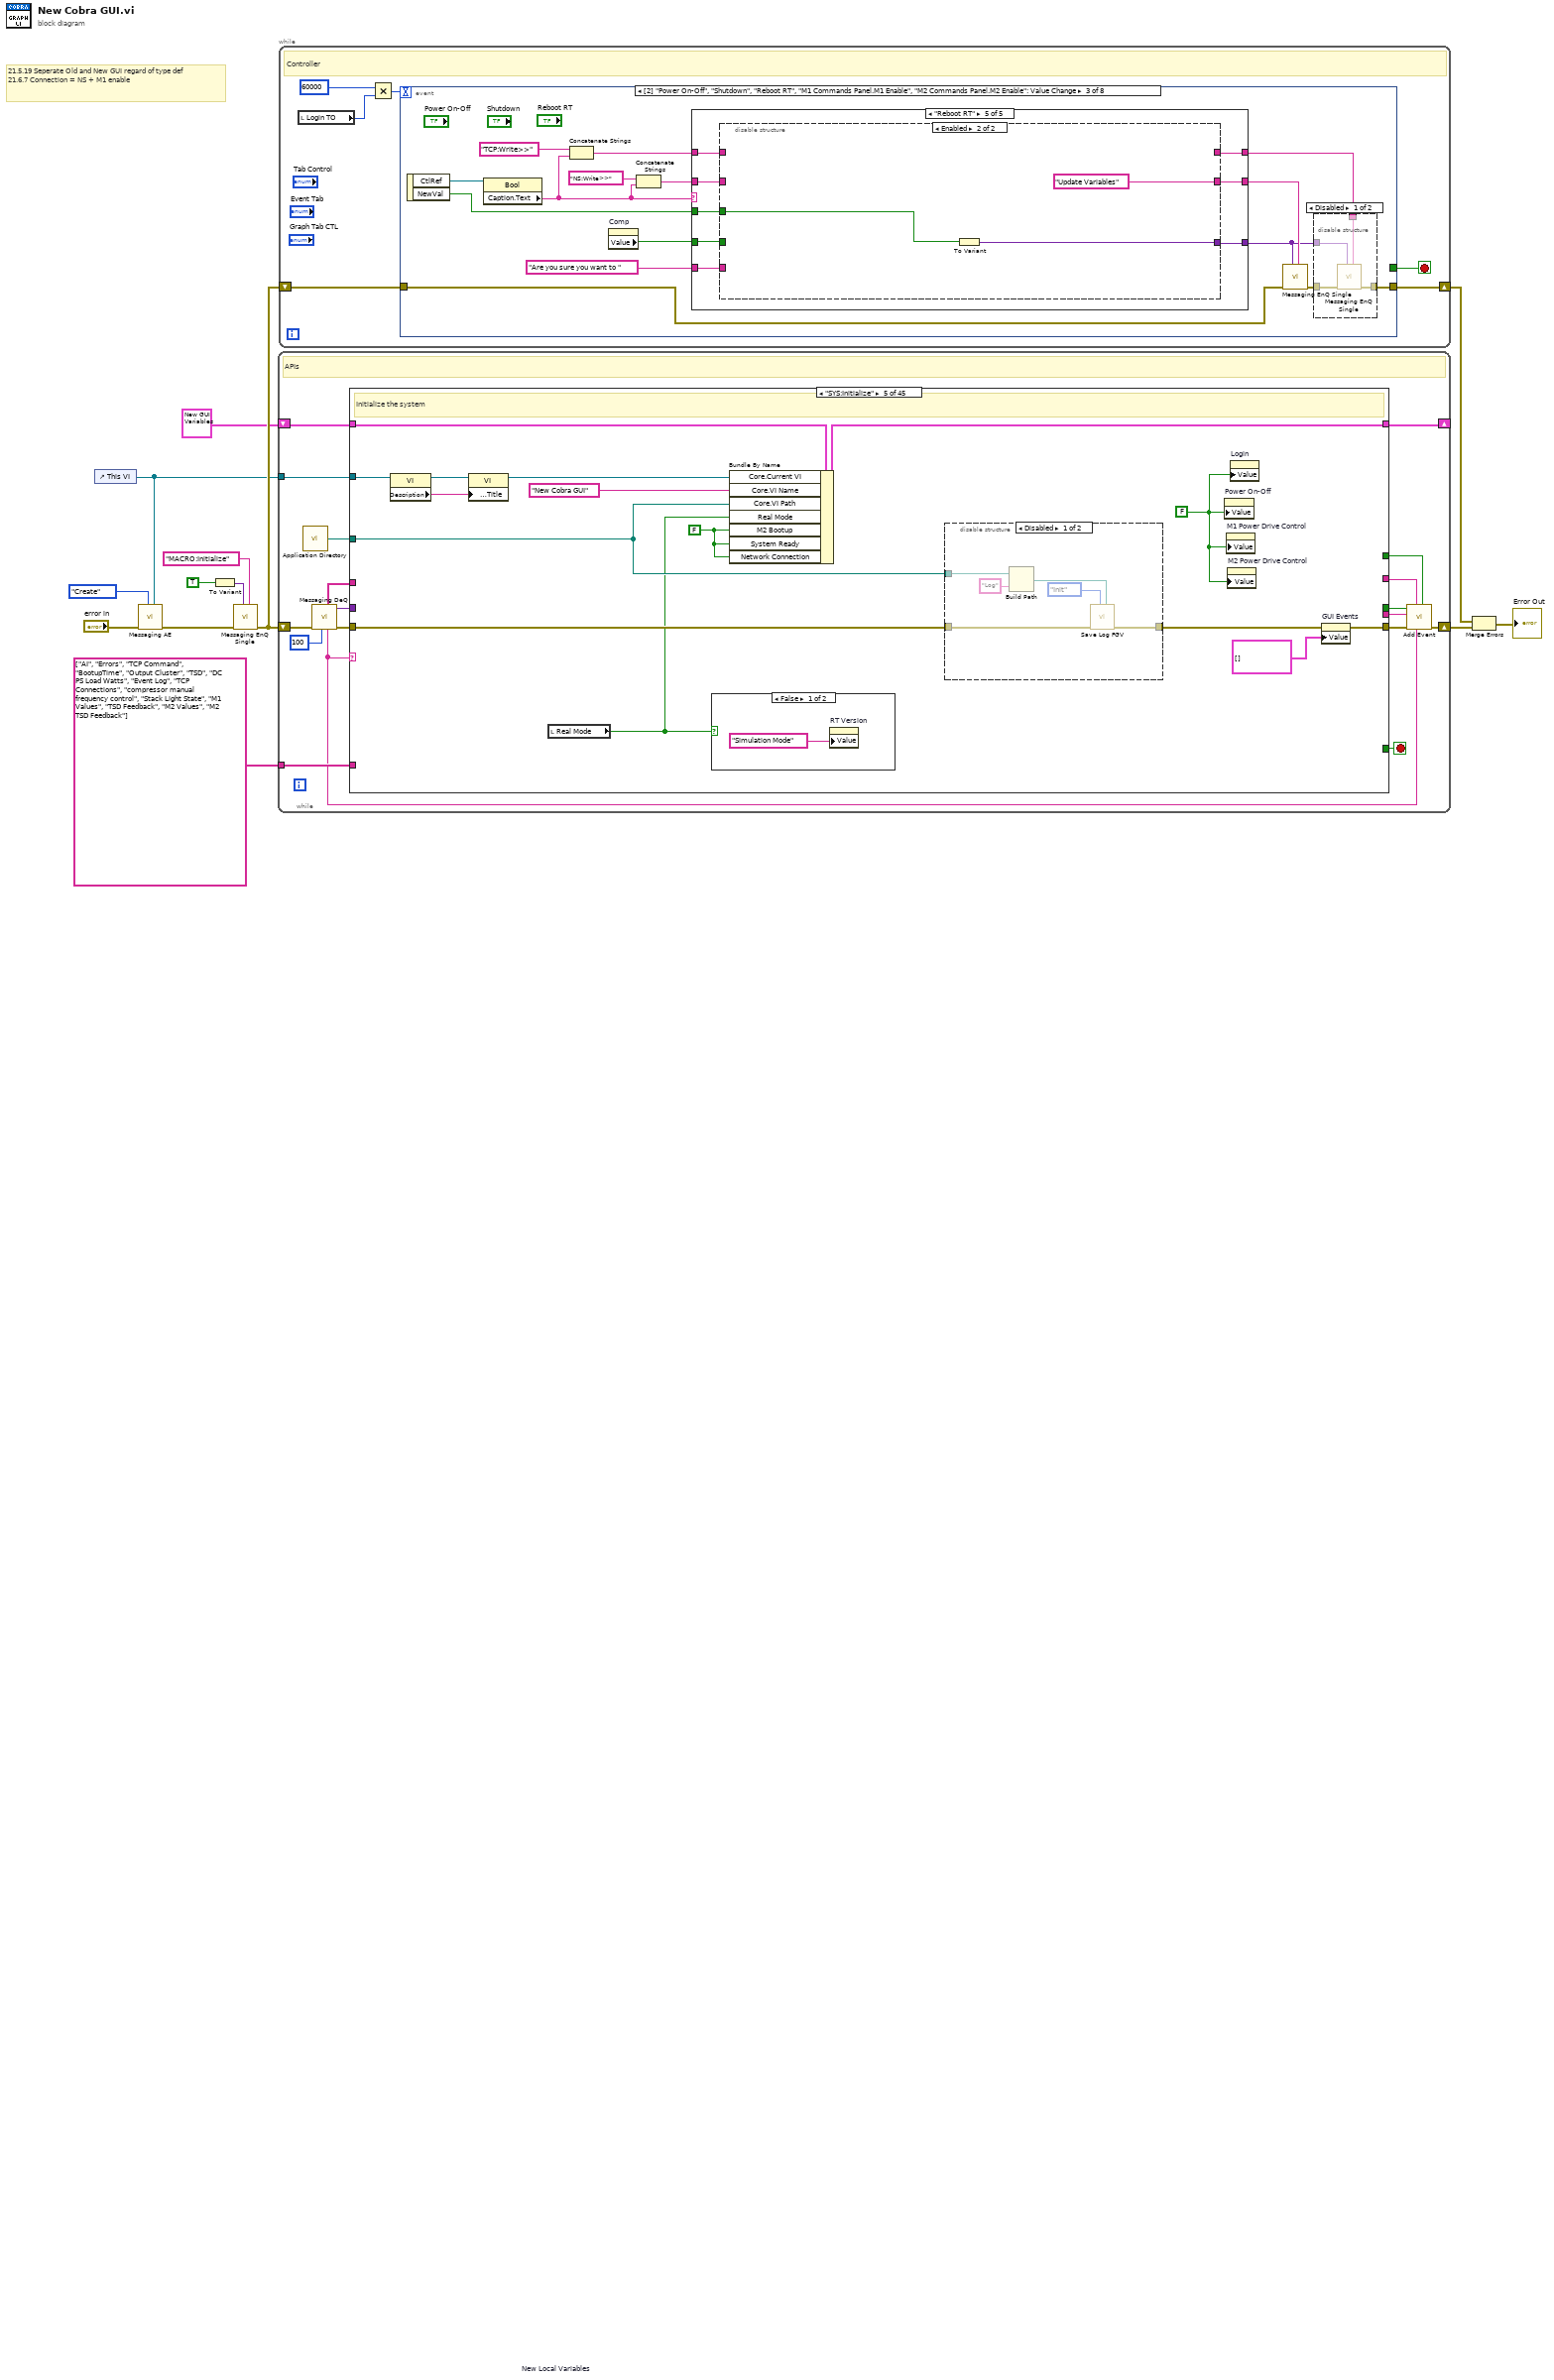
[diagram p0: block diagram]
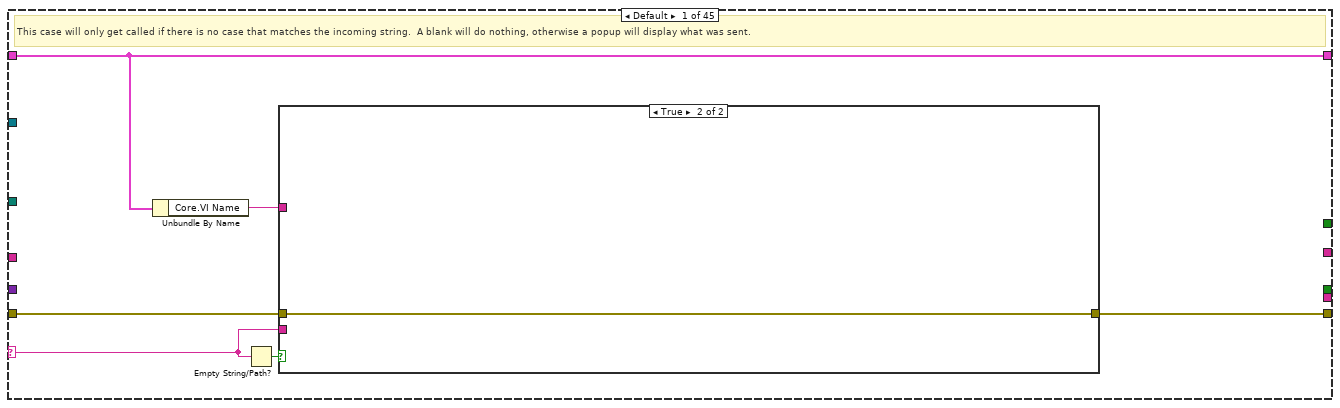
[diagram p2: hidden frame]
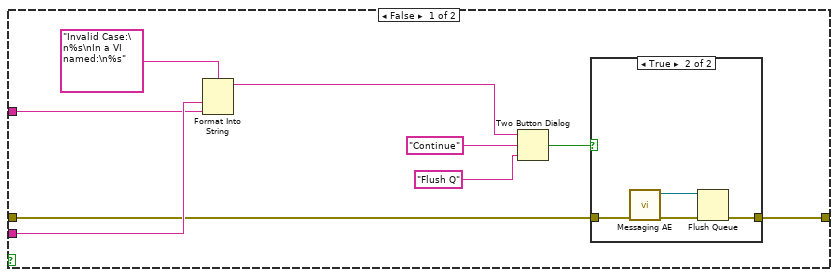
[diagram p3: hidden frame]
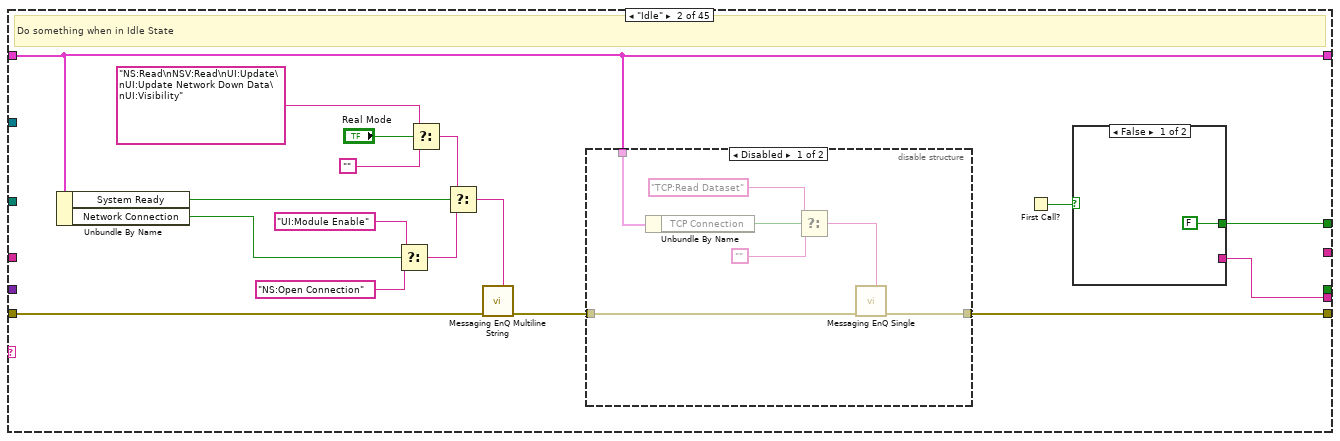
[diagram p5: hidden frame]
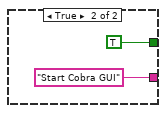
[diagram p7: hidden frame]
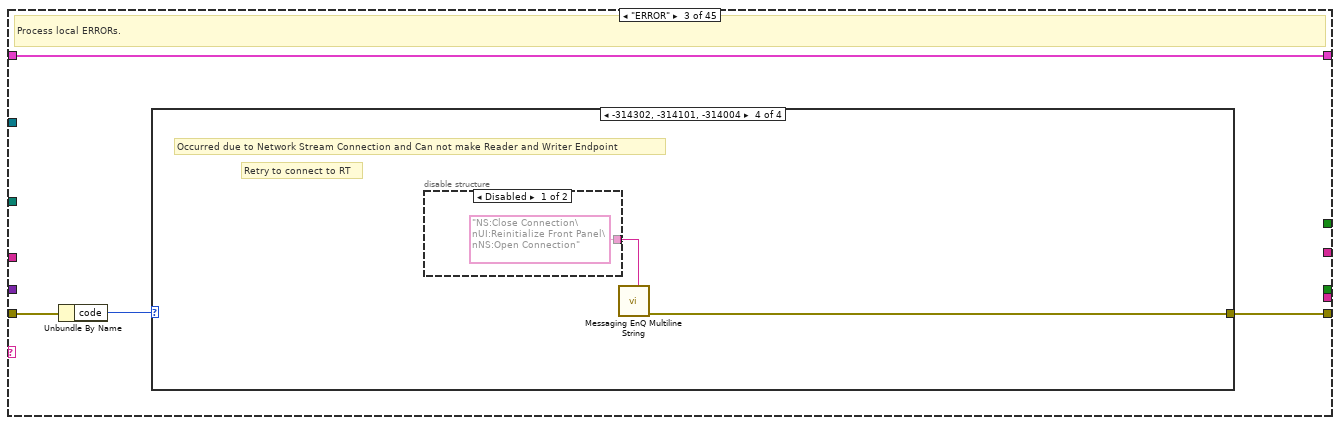
[diagram p8: hidden frame]
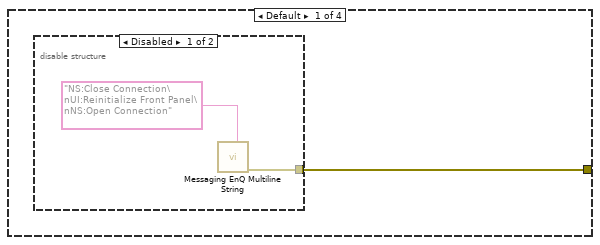
[diagram p9: hidden frame]
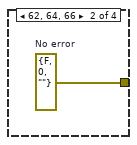
[diagram p11: hidden frame]
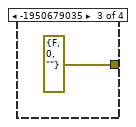
[diagram p12: hidden frame]
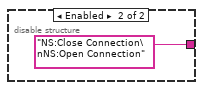
[diagram p13: hidden frame]
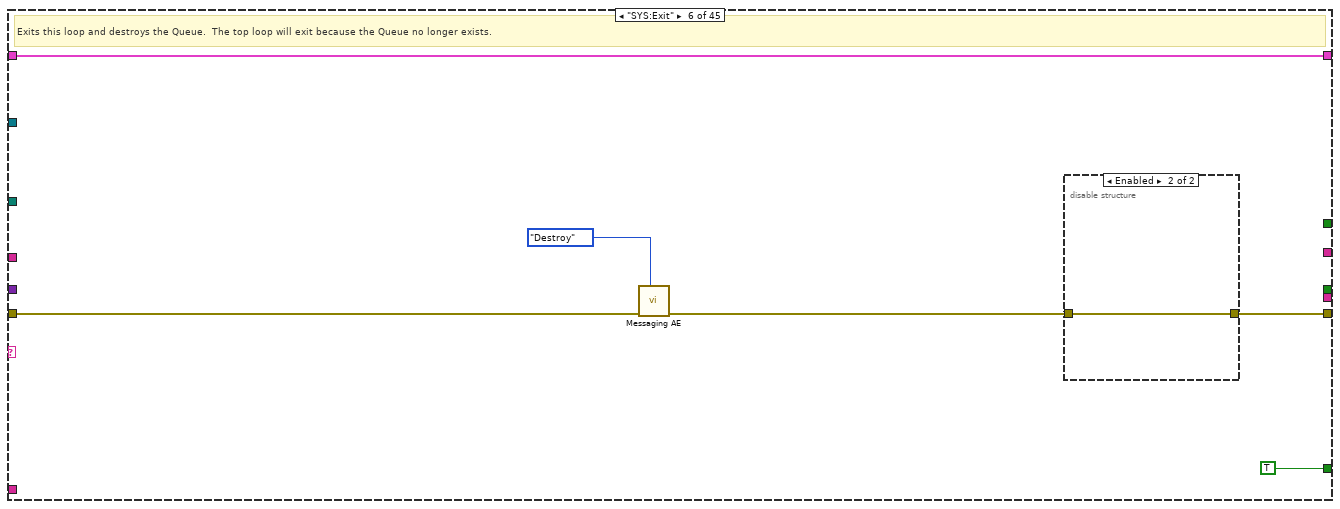
[diagram p17: hidden frame]
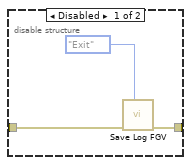
[diagram p18: hidden frame]
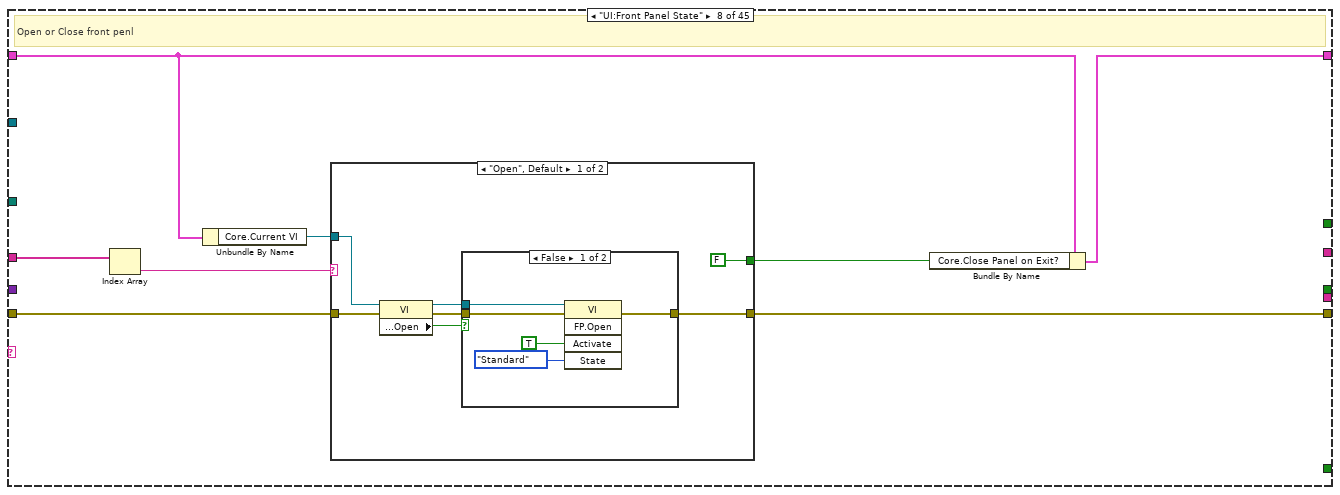
[diagram p20: hidden frame]
diagram:
  w2 = T24 {"Core"={"Current VI"=refnum, "Close Panel on Exit?"=FALSE, "VI Name"="", "VI Path"=path ""}, "reader endpoint"="", "writer endpoint"="", "Detected Systems"=[], "IP Address"="", "Network Connection"=FALSE, "M1 History Temps"=[], "M2 History Temps"=[], "System Ready"=FALSE, "M2 Bootup"=FALSE, "Network Data Down"={"M1 Commands"={"Set Temp"=20.0, "Power Drive"=FALSE, "Feedback"=1, "Package"=0, "Enable"=FALSE}, "M2 Commands"={"Set Temp"=20.0, "Power Drive"=FALSE, "Feedback"=1, "Package "=0, "Enable"=FALSE}, "Config Data"={"Packages"={"DUT Force lbf"={" 0"=0, " 1"=0, " 2"=0, "3"=0, "4"=0, "5"=0, " 6"=0, "7"=0, "8"=0, "9"=0}, "DUT Names"={"0"="", "1"="", "2"="", "3"="", "4"="", "5"="", "6"="", "7"="", "8"="", "9"=""}}, "Heater PID"={"P"=0.0, "I"=0.0, "D"=0.0}, "Piston Settings"={"Forces Slope"=0.0, "Forces Intercept"=0.0, "Transition Force"=0.0, "Up Force"=0.0, "Diameter (mm)"=0.0, "Delay (ms)"=0.0, "Pressure Ramp Delay (ms)"=0.0}, "Safe Temps"={"Minimum"=17, "Enabled"=TRUE, "Maximum"=95}, "System Settings"={"Number of Heads"=0, "60Hz Power"=TRUE, "FTC200"=TRUE, "AutoStartup"=FALSE, "Purge"=TRUE, "Sensors"=TRUE, "HandClamp"=TRUE, "ATE"=TRUE, "Benchtop"=TRUE, "Production"=TRUE, "Refrigerant"=enum."r404a", "Handler"=TRUE, "Shuttle"=TRUE, "220V"=FALSE, "Cascade"=FALSE, "Suction Sensor"=enum."YCQB02H01", "Discharge Sensor"=enum."YCQB05H01"}, "Stepper Settings "={"Microstepping"=enum."Full", "Velocity"=8}, "Set Point Range"={"Max"=0.0, "Min"=0.0}, "Pedestal Check DeltaT"=0.0, "Ramp Delta T"=0.0, "Ramp-SS Threshold"=0.0, "SS Tolerance"=0.0, "EEV PID"={"Ramp Up Target"=0.0, "Ramp Down Target"=0.0, "Steady State Target"=0.0, "Output"={"Max"=0.0, "Min"=0.0}, "EBB and Flow Temp TH"=0.0, "Cryomode EEV Max"=0.0, "Valve minimum opening "=0.0, "Ramp Up EEV Steps"=0.0, "Ramp Down EEV Steps"=0.0, "SS EEV Steps Reset"=0.0, "EBB and Flow Tol"=0.0, "Gains"={"P"=0.0, "I"=0.0, "D"=0.0}, "Dissabled Target"=0.0, "CryoMode Gains"={"P"=0.0, "I"=0.0, "D"=0.0}, "M1 SuperHeat Setpoint"=0.0, "M2 Gains"={"P"=0.0, "I"=0.0, "D"=0.0}, "Flow Curve"=enum.""}, "Sleep Timeout"=0.0, "Bypass Values"={"Bypass Valve"=TRUE, "Flow Curve"=enum."0", "Output"={"Max"=0, "Min"=0}, "Feedback"=enum."Temperature", "Cyth Bypass"=TRUE, "PID"={"P"=0.0, "I"=0.0, "D"=0.0}, "Pressure setpoint"=0, "Cryo Temp"=0, "Superheat Setpoint"=0, "Cryo Setpoint"=0}, "Default Temp"=0.0, "InTEC"={"Enabled"=FALSE, "IP"="192.168.1.100", "Port"=5000}, "M1 TSD"={"Gain"=0.0, "Offset"=0.0, "V Offset "=0.0}, "M2 TSD"={"Gain"=0.0, "Offset"=0.0, "V Offset "=0.0}, "M1 T-Case Calibration"={"Gain"=0.0, "Offset"=0.0}, "M2 T-Case Calibration"={"Gain"=0.0, "Offset"=0.0}, "Heater PID TSD"={"P"=0.0, "I"=0.0, "D"=0.0}, "M2 Heater PID"={"P"=0.0, "I"=0.0, "D"=0.0}}, "System Power On Off"=FALSE, "New Data"=enum."M1 Set Point", "Stop RT"=FALSE}, "Event Log"=[], "Connected System"="", "TCP connection info"={"connection ID"=refnum, "meta data"=[]}, "TCP Connection"=FALSE, "Dataset"={"System Status"={"Power On Off"=FALSE, "Discharge Temp"=0.0, "Liquid Temp"=0.0, "Suction Temp"=0.0, "Ambient Temp"=0.0, "Sleep"=FALSE, "System Status"=0, "M1 Actuated"=FALSE, "M2 Actuated"=FALSE, "Sleep Timer"=0.0, "M1 Bin"={"Bin String"="", "Bin Color"=1}, "M2 Bin"={"Bin String"="", "Bin Color"=1}, "Discharge Pressure"=0.0, "Suction Pressure"=0.0, "Compression Ratio"=0.0, "Compressor Amps"=0.0, "Compressor Hours"=0.0, "Bypass Steps"=0, "SubCooling"=0.0, "SuperHeat"=0.0, "Serial Number"="", "EMO detected"=FALSE, "EMO Tripped"=FALSE, "Thermal cutoff"=FALSE, "Thermal cutoff 2"=FALSE, "High Pressure switch"=FALSE, "Running Time"=timestamp(0 s since 1904-01-01), "SOM Status"={"Boot Up Time"=timestamp(0 s since 1904-01-01), "Software Version"="", "CPU Usage"=0.0, "Memory Available"=0.0, "SD card free space"=0.0, "SOM Storage"=0.0}, "Cascade Extra"={"Discharge Temp High Side"=0.0, "Suction Temp High Side"=0.0, "Liquid Temp High side"=0.0, "Discharge Pressure 2"=0.0, "Suction Pressure 2"=0.0, "Low Side RPM"=0.0, "High Side RPM"=0.0}}, "M1 Status"={"Case Temp"=0.0, "Evap Temp"=0.0, "Heater %"=0.0, "EEV Steps"=0, "Set Temp"=0.0, "Feedback"=0, "Power Drive"=FALSE, "Piston Volts"=0.0, "Safe Temp"=FALSE, "Power"=FALSE, "Thermal State"=0, "Error"=FALSE, "In tollerance"=FALSE, "Head State"=0, "Piston Force"=0.0, "Package"="", "Dynamic SV"=0.0, "PV"=0.0, "TSD Temp"=0.0, "AC Load Watts"=0.0, "DC Load Watts"=0.0, "Intec Feedback"=0.0}, "M2 Status"={"Case Temp"=0.0, "Evap Temp"=0.0, "Heater %"=0.0, "EEV Steps"=0, "Set Temp"=0.0, "Feedback"=0, "Power Drive"=FALSE, "Piston Volts"=0.0, "Safe Temp"=FALSE, "Power"=FALSE, "Thermal State"=0, "Error"=FALSE, "In tollerance"=FALSE, "Head State"=0, "Piston Force"=0.0, "Package"="", "Dynamic SV"=0.0, "PV"=0.0, "TSD Temp"=0.0, "AC Load Watts"=0.0, "DC Load Watts"=0.0, "Intec Feedback"=0.0}, "Config Data"={"Packages"={"DUT Force lbf"={" 0"=0, " 1"=0, " 2"=0, "3"=0, "4"=0, "5"=0, " 6"=0, "7"=0, "8"=0, "9"=0}, "DUT Names"={"0"="", "1"="", "2"="", "3"="", "4"="", "5"="", "6"="", "7"="", "8"="", "9"=""}}, "Heater PID"={"P"=0.0, "I"=0.0, "D"=0.0}, "Piston Settings"={"Forces Slope"=0.0, "Forces Intercept"=0.0, "Transition Force"=0.0, "Up Force"=0.0, "Diameter (mm)"=0.0, "Delay (ms)"=0.0, "Pressure Ramp Delay (ms)"=0.0}, "Safe Temps"={"Minimum"=17, "Enabled"=TRUE, "Maximum"=95}, "System Settings"={"Number of Heads"=0, "60Hz Power"=TRUE, "FTC200"=TRUE, "AutoStartup"=FALSE, "Purge"=TRUE, "Sensors"=TRUE, "HandClamp"=TRUE, "ATE"=TRUE, "Benchtop"=TRUE, "Production"=TRUE, "Refrigerant"=0, "Handler"=TRUE, "Shuttle"=TRUE, "220V"=FALSE, "Cascade"=FALSE, "Suction Sensor"=0, "Discharge Sensor"=0}, "Stepper Settings "={"Microstepping"=0, "Velocity"=8}, "Set Point Range"={"Max"=0.0, "Min"=0.0}, "Pedestal Check DeltaT"=0.0, "Ramp Delta T"=0.0, "Ramp-SS Threshold"=0.0, "SS Tolerance"=0.0, "EEV PID"={"Ramp Up Target"=0.0, "Ramp Down Target"=0.0, "Steady State Target"=0.0, "Output"={"Max"=0.0, "Min"=0.0}, "EBB and Flow Temp TH"=0.0, "Cryomode EEV Max"=0.0, "Valve minimum opening "=0.0, "Ramp Up EEV Steps"=0.0, "Ramp Down EEV Steps"=0.0, "SS EEV Steps Reset"=0.0, "EBB and Flow Tol"=0.0, "Gains"={"P"=0.0, "I"=0.0, "D"=0.0}, "Dissabled Target"=0.0, "CryoMode Gains"={"P"=0.0, "I"=0.0, "D"=0.0}, "M1 SuperHeat Setpoint"=0.0, "M2 Gains"={"P"=0.0, "I"=0.0, "D"=0.0}, "Flow Curve"=0}, "Sleep Timeout"=0.0, "Bypass Values"={"Bypass Valve"=TRUE, "Flow Curve"=0, "Output"={"Max"=0, "Min"=0}, "Feedback"=0, "Cyth Bypass"=TRUE, "PID"={"P"=0.0, "I"=0.0, "D"=0.0}, "Pressure setpoint"=0, "Cryo Temp"=0, "Superheat Setpoint"=0, "Cryo Setpoint"=0}, "Default Temp"=0.0, "InTEC"={"Enabled"=FALSE, "IP"="192.168.1.100", "Port"=5000}, "M1 TSD"={"Gain"=0.0, "Offset"=0.0, "V Offset "=0.0}, "M2 TSD"={"Gain"=0.0, "Offset"=0.0, "V Offset "=0.0}, "M1 T-Case Calibration"={"Gain"=0.0, "Offset"=0.0}, "M2 T-Case Calibration"={"Gain"=0.0, "Offset"=0.0}, "Heater PID TSD"={"P"=0.0, "I"=0.0, "D"=0.0}, "M2 Heater PID"={"P"=0.0, "I"=0.0, "D"=0.0}}}, "Real Mode"=FALSE, "Last Connected System"=enum."Single Head", "Reboot"=FALSE, "Test"=FALSE, "User"=enum."Operator"}  # New Local Variables
  # "21.5.19 Seperate Old and New GUI regard of type def\n21.6.7 Connection = NS + M1 enable"
  n1 = control-ref of="This VI"() -> (w1:refnum<vi>)
  n2 = call "Messaging AE.vi"("VI Refnum"=w1, "Action"=Messaging_Actions."Create", "Error In"="error in") -> ("Error Out"=w6:errorcluster)  [unwired: 7 in, 1 out]
  n3 = To Variant(anything=TRUE ("Init")) -> (Variant=w8:variant)
  n4 = call "Messaging EnQ Single.vi"("Command"="MACRO:Initialize", "Data"=w8, "error in (no error)"=w6) -> ("error out"=w10:errorcluster)  [unwired: 8 in]
  n5 = while {
    shift-right: [w21] -> w12
    shift-left: w10 -> [w30]
    shift-right: [w28] -> _
    shift-left: w2 -> [w24]
    tunnel: string[] ["AI", "Errors", "TCP Command", "BootupTime", "Output Cluster", "TSD", "DC PS Load Watts", "Event Log", "TCP Connections", "compressor manual frequency control", "Stack Light State", "M1 Values", "TSD Feedback", "M2 Values", "M2 TSD Feedback"] -> [w23]
    tunnel: w1 -> [w15]
    stop <- w31 stop-if-true
    # "APIs"
    n6 = call <vilib>:"Application Directory.vi"() -> ("Application Directory"=w14:path)
    n7 = call "Messaging DeQ.vi"("Time out"=100 ("SV Update Rate"), "Error In"=w30) -> ("error out"=w29:errorcluster, "Data"=w26:variant, "Command"=w20:string, "[String Data]"=w25:string[])  [unwired: 6 in]
    n8 = case shown="\"SYS:Initialize\"" w20 {
      selector: w20 -> [w33 _ _ _ _ _ _ _ _ _ _ _ _ _ _ _ _ _ _ _ _ _ _ _ _ _ _ _ _ _ _ _ _ _ _ _ _ _ _ _ w1930 _ _ _ _]
      tunnel: w29 -> [w35 w69 w81 w94 w109 w120 w129 w137 w166 w560 w582 w593 w663 w677 w745 w751 w778 w808 w870 w889 w901 w915 w930 w937 w946 w957 w1107 w1132 w1146 w1199 w1391 w1398 w1508 w1653 w1666 w1680 w1769 w1888 w1892 w1908 w1938 w1949 w1951 w1979 w2012]
      tunnel: [w34 w63 w82 w94 w107 w119 w129 w136 w166 w551 w568 w591 w643 w686 w745 w750 w773 w808 w870 w871 w899 w914 w934 w937 w942 w949 w1097 w1126 w1147 w1205 w1391 w1396 w1507 w1653 w1658 w1675 w1773 w1881 w1892 w1909 w1933 w1949 w1959 w1994 w2011] -> w22
      tunnel: [_ _ _ _ _ TRUE _ _ _ _ _ _ _ _ _ _ _ _ _ _ _ _ _ _ _ _ _ _ _ _ _ _ _ _ _ _ _ _ _ _ _ _ _ _ _] -> w31
      tunnel: [w32 w62 w80 w93 w103 w121 w128 w131 w165 w563 w569 w592 w661 w689 w730 w754 w779 w809 w869 w876 w894 w912 w931 w936 w944 w955 w1093 w1127 w1149 w1197 w1390 w1402 w1511 w1652 w1660 w1671 w1772 w1887 w1891 w1904 w1934 w1948 w1958 w1995 w2008] -> w28
      tunnel: w24 -> [w32 w62 w80 w93 w104 w121 w128 w132 w164 w563 w569 w592 w660 w679 w729 w762 w779 w809 w869 w876 w894 w913 w931 w936 w945 w953 w1091 w1128 w1134 w1198 w1390 w1402 w1511 w1652 w1661 w1672 w1772 w1887 w1891 w1905 w1939 w1948 w1958 w1995 w2009]
      tunnel: w25 -> [_ _ _ _ _ _ _ w135 _ _ _ _ _ _ _ _ _ _ _ _ _ _ _ _ _ _ _ _ _ w1209 _ w1399 _ _ _ _ w1770 _ _ _ _ _ w1957 _ _]
      tunnel: w26 -> [_ _ _ _ _ _ _ _ _ w559 w581 _ w662 _ _ _ _ _ _ w887 w902 _ _ _ _ w956 _ _ _ w1200 _ w1397 _ _ _ _ w1768 _ _ w1907 w1937 _ _ _ w2007]
      tunnel: w23 -> [_ _ _ _ _ _ _ _ _ _ _ _ _ _ _ _ _ _ _ _ _ _ _ _ _ _ _ _ _ _ _ _ w1509 _ _ _ _ _ _ _ _ _ _ _ _]
      tunnel: [_ w66 _ _ _ _ _ _ _ _ _ _ _ w675 _ w746 _ _ _ _ _ _ TRUE ("Boolean") _ _ _ w1088 _ w1139 TRUE ("Connected") _ TRUE ("Connected") _ _ TRUE ("Visible") _ TRUE ("Visible") TRUE ("Visible") _ w1893 _ _ _ _ _] -> w19
      tunnel: [_ _ _ _ _ _ _ _ _ _ _ _ _ w675 _ w746 _ _ _ _ _ _ _ _ _ _ w1088 _ w1138 _ _ w1392 _ _ TRUE ("TSD Feedback") _ w1765 _ _ _ _ _ _ _ _] -> w18
      tunnel: [_ w65 _ _ _ _ _ _ _ _ _ _ _ _ _ "System Ready" ("Command") _ _ _ _ _ _ "Stop Cobra GUI" ("String") _ _ _ w1092 _ w1137 w1195 _ w1394 _ _ "Open a TCP port " ("Name") _ w1766 "Close the connected client" ("Name") _ w1897 _ _ _ _ _] -> w17
      tunnel: [_ _ _ _ _ _ _ _ _ _ _ _ _ _ _ _ _ _ _ _ _ _ _ _ _ _ _ _ _ w1194 _ w1393 _ _ w1659 _ w1762 _ _ _ _ _ _ _ _] -> w16
      tunnel: w15 -> [_ _ _ _ w101 _ _ _ _ _ _ _ _ _ _ _ _ _ _ _ _ _ _ _ _ _ _ _ _ _ _ _ _ _ _ _ _ _ _ _ _ _ _ _ _]
      tunnel: w14 -> [_ _ _ _ w98 _ _ _ _ _ _ _ _ _ _ _ _ _ _ _ _ _ _ _ _ _ _ _ _ _ _ _ _ _ _ _ _ _ _ _ _ _ _ _ _]
      frame Default {
        # "This case will only get called if there is no case that matches the incoming string.  A blank will do nothing, otherwise a popup will display what was sent."
        n9 = Unbundle By Name(w32) -> ("Core.VI Name"=w36:string)
        n10 = Empty String/Path?(string/path=w33) -> (empty?=w37:bool)
        n11 = case shown="True" w37 {
          tunnel: [w45 w52] -> w34
          tunnel: w35 -> [w38 w52]
          tunnel: w33 -> [w40 _]
          tunnel: w36 -> [w39 _]
          frame False {
            n12 = Format Into String(format string="Invalid Case:\n%s\nIn a VI named:\n%s", w40, w39) -> (resulting string=w42:string)  [unwired: 2 in, 1 out]
            n13 = Two Button Dialog(message=w42, 1:"Flush Q" ("T button name (\"OK\")"), 2:"Continue" ("T button name (\"OK\")")) -> (T button?=w46:bool)
            n14 = case shown="True" w46 {
              tunnel: w38 -> [w47 w50]
              tunnel: [w47 w51] -> w45
              frame False {
              }
              frame True {
                n15 = call "Messaging AE.vi"("Error In"=w50) -> ("Error Out"=w49:errorcluster, "queue out"=w48:refnum<queue>)  [unwired: 9 in]
                n16 = Flush Queue(queue=w48, error in (no error)=w49) -> (error out=w51:errorcluster)  [unwired: 2 out]
              }
            }
          }
          frame True {
          }
        }
      }
      frame "Idle" {
        # "Do something when in Idle State"
        n17 = Unbundle By Name(w62) -> ("System Ready"=w68:bool, "Network Connection"=w61:bool)
        n18 = Select(t="UI:Module Enable" ("Command"), s=w61, f="NS:Open Connection" ("Command")) -> (s? t:f=w60:string)
        n19 = Select(t="NS:Read\nNSV:Read\nUI:Update\nUI:Update Network Down Data\nUI:Visibility" ("Command(s)"), s="Real Mode", f="") -> (s? t:f=w55:string)
        n20 = Select(t=w55, s=w68, f=w60) -> (s? t:f=w54:string)
        n21 = call "Messaging EnQ Multiline String.vi"("Command(s)"=w54, "error in (no error)"=w69) -> ("error out"=w64:errorcluster)  [unwired: 9 in]
        n22 = disable-structure shown="Disabled" {
          disable-tunnel: w64 -> [w76 _]
          disable-tunnel: [w75 _] -> w63
          disable-tunnel: w62 -> [w74 _]
          frame Disabled {
            n23 = Unbundle By Name(w74) -> ("TCP Connection"=w73:bool)
            n24 = Select(t="TCP:Read Dataset" ("Command"), s=w73, f="") -> (s? t:f=w70:string)
            n25 = call "Messaging EnQ Single.vi"("Command"=w70, "error in (no error)"=w76) -> ("error out"=w75:errorcluster)  [unwired: 9 in]
          }
          frame Enabled {
          }
        }
        n26 = First Call?() -> (First Call?: T/F=w67:bool)
        n27 = case shown="False" w67 {
          tunnel: [FALSE ("Boolean") TRUE ("Boolean")] -> w66
          tunnel: [_ "Start Cobra GUI" ("String")] -> w65
          frame False {
          }
          frame True {
          }
        }
      }
      frame "ERROR" {
        # "Process local ERRORs."
        n28 = Unbundle By Name(w81) -> ("code"=w83:i32)
        n29 = case shown="-314302, -314101, -314004" w83 {
          tunnel: [w84 w87 errorcluster {"status"=FALSE, "code"=0, "source"=""} ("error out") w90] -> w82
          frame Default {
            n30 = disable-structure shown="Disabled" {
              disable-tunnel: [w86 _] -> w84
              frame Disabled {
                n31 = call "Messaging EnQ Multiline String.vi"("Command(s)"="NS:Close Connection\nUI:Reinitialize Front Panel\nNS:Open Connection" ("Command")) -> ("error out"=w86:errorcluster)  [unwired: 10 in]
              }
              frame Enabled {
              }
            }
          }
          frame 62, 64, 66 {
            w87 = errorcluster {"status"=FALSE, "code"=0, "source"=""}  # No error
          }
          frame -1950679035 {
          }
          frame -314302, -314101, -314004 {
            # "Retry to connect to RT"
            # "Occurred due to Network Stream Connection and Can not make Reader and Writer Endpoint"
            n32 = disable-structure shown="Disabled" {
              disable-tunnel: ["NS:Close Connection\nUI:Reinitialize Front Panel\nNS:Open Connection" ("Command") "NS:Close Connection\nNS:Open Connection" ("Command")] -> w89
              frame Disabled {
              }
              frame Enabled {
              }
            }
            n33 = call "Messaging EnQ Multiline String.vi"("Command(s)"=w89) -> ("error out"=w90:errorcluster)  [unwired: 10 in]
          }
        }
      }
      frame "-----System-----" {
        # "Command Format:\nCAT:Command>>Data1,Data2,DataN"
        # "SYSTEM is used for things that directly effect this module"
      }
      frame "SYS:Initialize" {
        w97 = FALSE ("M2 Bootup")
        w95 = FALSE ("Power On-Off")
        # "Initialize the system"
        n34 = property class="VI"(reference=w101) -> (reference out=w100:refnum<vi>, "Description"=w99:string)  [unwired: 1 in, 1 out]
        n35 = property class="VI"(reference=w100, "Front Panel.Title"=w99) -> (reference out=w106:refnum<vi>)  [unwired: 1 in, 1 out]
        n36 = local read "Real Mode"() -> (w96:bool)
        n37 = case shown="False" w96 {
          frame False {
            n38 = property on="RT Version" class="Str"("Value"="Simulation Mode" ("f")) -> ()  [unwired: 2 in, 2 out]
          }
          frame True {
          }
        }
        n39 = Bundle By Name(cluster=w104, "Core.Current VI"=w106, "Core.VI Name"="New Cobra GUI" ("VI Name"), "Core.VI Path"=w98, "Real Mode"=w96, "M2 Bootup"=w97, "System Ready"=w97, "Network Connection"=w97) -> (w103:T24)
        n40 = disable-structure shown="Disabled" {
          disable-tunnel: w109 -> [w115 w117]
          disable-tunnel: [w112 w117] -> w102
          disable-tunnel: w98 -> [w111 _]
          frame Disabled {
            n41 = Build Path(base path=w111, name or relative path="Log") -> (appended path=w113:path)
            n42 = call "Save Log FGV.vi"("Log Path"=w113, "State"=Save_Log_State."Init", "Error In"=w115) -> ("Error Out"=w112:errorcluster)  [unwired: 8 in]
          }
          frame Enabled {
          }
        }
        n43 = property on="Power On-Off" class="Bool (strict)"("Value"=w95) -> ()  [unwired: 2 in, 2 out]
        n44 = property on="M1 Power Drive Control" class="Bool (strict)"("Value"=w95) -> ()  [unwired: 2 in, 2 out]
        n45 = property on="M2 Power Drive Control" class="Bool (strict)"("Value"=w95) -> ()  [unwired: 2 in, 2 out]
        n46 = property on="Login" class="Bool (strict)"("Value"=w95) -> ()  [unwired: 2 in, 2 out]
        n47 = property on="GUI Events" class="Arr (strict)"(error in=w102, "Value"=T20[] [] ("GUI Events")) -> (error out=w107:errorcluster)  [unwired: 1 in, 1 out]
      }
      frame "SYS:Exit" {
        # "Exits this loop and destroys the Queue.  The top loop will exit because the Queue no longer exists."
        n48 = call "Messaging AE.vi"("Action"=Messaging_Actions."Destroy", "Error In"=w120) -> ("Error Out"=w118:errorcluster)  [unwired: 8 in, 1 out]
        n49 = disable-structure shown="Enabled" {
          disable-tunnel: [w126 w127] -> w119
          disable-tunnel: w118 -> [w124 w127]
          frame Disabled {
            n50 = call "Save Log FGV.vi"("State"=Save_Log_State."Exit", "Error In"=w124) -> ("Error Out"=w126:errorcluster)  [unwired: 9 in]
          }
          frame Enabled {
          }
        }
      }
      frame "-----User Interface-----" {
        # "UI is used for things that will change the UI.,"
      }
      frame "UI:Front Panel State" {
        # "Open or Close front penl"
        n51 = Index Array(array=w135) -> (element=w134:string)  [unwired: 1 in]
        n52 = Unbundle By Name(w132) -> ("Core.Current VI"=w133:refnum<vi>)
        n53 = case shown="\"Open\", Default" w134 {
          tunnel: w137 -> [w142 w156]
          tunnel: [w144 w157] -> w136
          tunnel: w133 -> [w143 w154]
          tunnel: [FALSE ("Core.Close Panel on Exit?") w151] -> w130
          frame "Open", Default {
            n54 = property class="VI"(reference=w143, error in=w142) -> (reference out=w140:refnum<vi>, error out=w141:errorcluster, "Front Panel.Open"=w139:bool)
            n55 = case shown="False" w139 {
              tunnel: [w147 w150] -> w144
              tunnel: w141 -> [w146 w150]
              tunnel: w140 -> [w145 _]
              frame False {
                n56 = invoke class="VI" method="FP.Open"(reference=w145, error in=w146, "Activate"=TRUE, "State"=T35."Standard") -> (error out=w147:errorcluster)  [unwired: 1 in, 4 out]
              }
              frame True {
              }
            }
          }
          frame "Close" {
            n57 = property class="VI"(reference=w154, error in=w156) -> (reference out=w153:refnum<vi>, error out=w155:errorcluster, "Front Panel.Open"=w152:bool)
            n58 = case shown="False" w152 {
              tunnel: [w159 w163] -> w157
              tunnel: w155 -> [w159 w162]
              tunnel: w153 -> [_ w161]
              tunnel: [FALSE ("Core.Close Panel on Exit?") TRUE ("Core.Close Panel on Exit?")] -> w151
              frame False {
              }
              frame True {
                n59 = invoke class="VI" method="FP.Close"(reference=w161, error in=w162) -> (error out=w163:errorcluster)  [unwired: 1 in, 2 out]
              }
            }
          }
        }
        n60 = Bundle By Name(cluster=w132, "Core.Close Panel on Exit?"=w130) -> (w131:T24)
      }
      frame "UI:Update" {
        n61 = stacked-sequence {
          tunnel: w164 -> [w172 w198 w230 w261 w303 w352 w400 w423 w503 w512]
          tunnel: w164 -> [_ _ _ _ _ _ _ w446 _ _]
          tunnel: [_ _ _ _ _ _ _ w445 _ _] -> w165
          frame #0 {
            # "Update System Module Data"
            n62 = Unbundle By Name(w172) -> ("Dataset.System Status"=w179:T30)
            n63 = Unbundle By Name(w179) -> ("Compression Ratio"=w176:dbl, "Compressor Amps"=w175:dbl, "Discharge Pressure"=w174:dbl, "Suction Pressure"=w173:dbl, "SubCooling"=w171:dbl, "SuperHeat"=w170:dbl, "Cascade Extra.High Side RPM"=w180:dbl, "Cascade Extra.Low Side RPM"=w182:dbl)
            n64 = Round To Nearest(number=w182) -> (nearest integer value=→"Low Side RPM":dbl)
            n65 = Round To Nearest(number=w180) -> (nearest integer value=→"High Side RPM":dbl)
            n66 = local read "Graph Temp Unit"() -> (w167:bool)
            n67 = case shown="False" w167 {
              tunnel: w171 -> [w185 w191]
              tunnel: w170 -> [w184 w190]
              tunnel: [w185 w187] -> w169
              tunnel: [w184 w186] -> w168
              frame False {
              }
              frame True {
                n68 = Build Array(w191, w190) -> (w189:dbl[])
                n69 = for {
                  tunnel: w189 -> [w193] mode=indexing
                  tunnel: [w192] -> w188 mode=indexing
                  n70 = expression code="5/9*(x-32)"(w193) -> (w192:dbl)
                }
                n71 = Index Array(array=w188) -> (element #1=w187:dbl, element #2=w186:dbl)  [unwired: 2 in]
              }
            }
            n72 = Bundle By Name(cluster=T13 {"Condensing Pressure(psi)"=0.0, "Compression Ratio"=0.0, "Subcool"=0.0, "Superheat"=0.0, "Current(A)"=0.0, "Suction Pressure(psi)"=0.0} ("Gauges"), "Compression Ratio"=w176, "Current(A)"=w175, "Condensing Pressure(psi)"=w174, "Suction Pressure(psi)"=w173, "Subcool"=w169, "Superheat"=w168) -> (→"Gauges":T13)
          }
          frame #1 {
            # "Update M1 Module Data"
            n73 = Unbundle By Name(w198) -> ("Dataset.System Status.M1 Bin.Bin String"=→"M1 Bin String":string, "Dataset.System Status.M1 Bin.Bin Color"=w204:u16)
            n74 = Unbundle By Name(w198) -> ("Dataset.M1 Status.Thermal State"=→"M1 Thermal State":u16, "Dataset.M1 Status.Power Drive"=→"M1 Power Drive Indicator":bool)
            n75 = case shown="0, Default" w204 {
              tunnel: [u32 14342874 u32 16777215 u32 16712704 u32 56399 u32 1185791 u32 2818010 u32 15701504] -> w206
              frame 0, Default {
              }
              frame 1 {
              }
              frame 2 {
              }
              frame 3 {
              }
              frame 4 {
              }
              frame 5 {
              }
              frame 6 {
              }
            }
            n76 = property on="M1 Bin String" class="Str"("Text.BGColor"=w206) -> ()  [unwired: 2 in, 2 out]
            n77 = Unbundle By Name(w198) -> ("Dataset.M1 Status.Evap Temp"=w202:dbl, "Dataset.M1 Status.Case Temp"=w201:dbl, "Dataset.M1 Status.Intec Feedback"=w200:dbl, "Dataset.M1 Status.TSD Temp"=w199:dbl, "Dataset.M1 Status.Feedback"=w196:u8)
            n78 = case shown="3" w196 {
              tunnel: w202 -> [w209 _ _ _ _ _]
              tunnel: w201 -> [_ w211 _ _ _ _]
              tunnel: [w209 w211 w213 w215 nan nan] -> w197
              tunnel: w200 -> [_ _ w213 _ _ _]
              tunnel: w199 -> [_ _ _ w215 _ _]
              tunnel: ["M1 Evap Temp" ("Command") "M1 Case Temp" ("Command") "M1 Intec Temp" ("Command") "M1 TSD" ("Command") "M1 Auto Tune" ("Command") "M1 Extra" ("Command")] -> w194
              frame 0, Default {
                # "Evap Temp"
              }
              frame 1 {
                # "Case Temp"
              }
              frame 2 {
                # "intec Temp"
              }
              frame 3 {
                # "TSD"
              }
              frame 4 {
                # "Auto Tune"
              }
              frame 5 {
                # "Extra"
              }
            }
            n79 = property on="M1 PV" class="DigNum (strict)"("Value"=w197, "Caption.Text"=w194, "Caption.FontBold"=TRUE ("Caption.Font:Bold")) -> ()  [unwired: 2 in, 2 out]
          }
          frame #2 {
            # "Update M2 Module Data"
            n80 = Unbundle By Name(w230) -> ("Dataset.System Status.M2 Bin.Bin String"=→"M2 Bin String":string, "Dataset.System Status.M2 Bin.Bin Color"=w239:u16)
            n81 = Unbundle By Name(w230) -> ("Dataset.M2 Status.Thermal State"=→"M2 Thermal State":u16, "Dataset.M2 Status.Power Drive"=→"M2 Power Drive Indicator":bool)
            n82 = case shown="4" w239 {
              tunnel: [u32 14342874 u32 16777215 u32 16712704 u32 56399 u32 1185791 u32 2818010 u32 15701504] -> w238
              frame 0, Default {
              }
              frame 1 {
              }
              frame 2 {
              }
              frame 3 {
              }
              frame 4 {
              }
              frame 5 {
              }
              frame 6 {
              }
            }
            n83 = property on="M2 Bin String" class="Str"("Text.BGColor"=w238) -> ()  [unwired: 2 in, 2 out]
            n84 = Unbundle By Name(w230) -> ("Dataset.M2 Status.Evap Temp"=w235:dbl, "Dataset.M2 Status.Case Temp"=w234:dbl, "Dataset.M2 Status.Intec Feedback"=w233:dbl, "Dataset.M2 Status.TSD Temp"=w232:dbl, "Dataset.M2 Status.Feedback"=w231:u8)
            n85 = case shown="3" w231 {
              tunnel: w235 -> [w242 _ _ _ _ _]
              tunnel: w234 -> [_ w244 _ _ _ _]
              tunnel: [w242 w244 w246 w248 nan nan] -> w229
              tunnel: w233 -> [_ _ w246 _ _ _]
              tunnel: w232 -> [_ _ _ w248 _ _]
              tunnel: ["M2 Evap Temp" ("Caption.Text") "M2 Case Temp" ("Caption.Text") "M2 Intec Temp" ("Caption.Text") "M2 TSD" ("Caption.Text") "M2 Auto Tune" ("Caption.Text") "M2 Extra" ("Caption.Text")] -> w227
              frame 0, Default {
                # "Evap Temp"
              }
              frame 1 {
                # "Case Temp"
              }
              frame 2 {
                # "intec Temp"
              }
              frame 3 {
                # "TSD"
              }
              frame 4 {
                # "Auto Tune"
              }
              frame 5 {
                # "Extra"
              }
            }
            n86 = property on="M2 PV" class="DigNum (strict)"("Value"=w229, "Caption.Text"=w227, "Caption.FontBold"=TRUE ("Caption.Font:Bold")) -> ()  [unwired: 2 in, 2 out]
          }
          frame #3 {
            # "System information For Debugging"
            n87 = Unbundle By Name(w261) -> ("Dataset.M1 Status"=w291:T31)
            n88 = Unbundle By Name(w261) -> ("Dataset.M2 Status"=w288:T31)
            n89 = Unbundle By Name(w261) -> ("Dataset.System Status"=w275:T30)
            n90 = Unbundle By Name(w288) -> ("Head State"=→"M2 Head State":u16, "Thermal State"=→"M2 Thermal Status":u16, "Error"=→"M2 Error":bool, "Heater %"=→"M2 Heater %":dbl)
            n91 = Unbundle By Name(w291) -> ("Head State"=→"M1 Head State":u16, "Thermal State"=→"M1 Thermal Status":u16, "Error"=→"M1 Error":bool, "Heater %"=→"M1 Heater %":dbl)
            n92 = Unbundle By Name(w275) -> ("SOM Status"=w274:T43)
            n93 = Unbundle By Name(w274) -> ("Memory Available"=w273:dbl, "SOM Storage"=w272:dbl, "SD card free space"=w263:dbl, "CPU Usage"=w268:dbl, "Software Version"=w260:string)
            "RT Version" <- w260
            n94 = Unbundle By Name(w275) -> ("M1 Actuated"=→"M1 Actuated":bool, "M2 Actuated"=→"M2 Actuated":bool, "Sleep"=→"Sleep":bool, "Sleep Timer"=→"Sleep Timer":dbl, "Discharge Temp"=→"Comp Temp":dbl, "Compressor Hours"=→"Compressor Hours":dbl, "Serial Number"=→"Serial Number":string)
            n95 = Build Array(w273, w272, w263) -> (w271:dbl[])
            n96 = for {
              tunnel: w271 -> [w293] mode=indexing
              tunnel: [w292] -> w270 mode=indexing
              n97 = Divide(x=w293, y=1000.0) -> (x/y=w292:dbl)
            }
            n98 = Index Array(array=w270) -> (element #1=w269:dbl, element #2=w266:dbl, element #3=w262:dbl)  [unwired: 3 in]
            n99 = Bundle By Name(cluster=T23 {"Software Version"="SW Version:CC 21.5.11.0", "CPU Usage"=46.7905609206245, "Memory Available"=349.908, "SOM Storage(MB)"=241.236, "SD card free space"=31661.0} ("SOM"), "Memory Available"=w269, "SOM Storage(MB)"=w266, "SD card free space"=w262, "CPU Usage"=w268, "Software Version"=w260) -> (→"SOM":T23)
          }
          frame #4 {
            # "Graphs in Control Tab (Fit Y-Scale at Main Waveform Charts )"
            n100 = Unbundle By Name(w303) -> ("Dataset.M1 Status"=w314:T31)
            n101 = Unbundle By Name(w303) -> ("Dataset.M2 Status"=w310:T31)
            n102 = Unbundle By Name(w310) -> ("Set Temp"=w304:dbl, "Evap Temp"=w309:dbl, "Case Temp"=w308:dbl, "TSD Temp"=w307:dbl, "AC Load Watts"=w306:dbl)
            n103 = Unbundle By Name(w314) -> ("Set Temp"=w305:dbl, "Evap Temp"=w313:dbl, "Case Temp"=w311:dbl, "TSD Temp"=w312:dbl, "Intec Feedback"=w295:dbl, "AC Load Watts"=w296:dbl)
            n104 = Build Array(w305, w313, w311, w312, w295, w296) -> (w301:dbl[])
            "M1 Channels" <- w301
            n105 = Build Array(w304, w309, w308, w307, w306) -> (w299:dbl[])
            "M2 Channels" <- w299
            n106 = control-ref of="M1 Main Waveform"() -> (w302:refnum<vi>)
            n107 = control-ref of="M2 Main Waveform"() -> (w300:refnum<vi>)
            n108 = case shown="False" "Y-scale" {
              tunnel: w302 -> [w319 w335]
              tunnel: w301 -> [_ w334]
              tunnel: w300 -> [w316 w333]
              tunnel: w299 -> [_ w332]
              tunnel: [T36."Disabled and Grayed Out" ("Disabled") T36."Enabled" ("Disabled")] -> w297
              frame False {
                # "Y- Autoscale"
                n109 = property on="Property Node" class="WFChart (strict)"(reference=w319, "YScale.ScaleFit"=u8 2 ("Y Scale.Scale Fit")) -> ()  [unwired: 1 in, 2 out]
                n110 = property on="Property Node" class="WFChart (strict)"(reference=w316, "YScale.ScaleFit"=u8 2 ("Y Scale.Scale Fit")) -> ()  [unwired: 1 in, 2 out]
              }
              frame True {
                # "Manually fix the Y-scale"
                n111 = Array Max & Min(array=w334) -> (max value=w328:dbl, min value=w329:dbl)  [unwired: 2 out]
                n112 = Array Max & Min(array=w332) -> (max value=w323:dbl, min value=w324:dbl)  [unwired: 2 out]
                n113 = Add(x=w328, y="Fixed Y-Range") -> (x+y=w330:dbl)
                n114 = Subtract(x=w329, y="Fixed Y-Range") -> (x-y=w331:dbl)
                n115 = Add(x=w323, y="Fixed Y-Range") -> (x+y=w325:dbl)
                n116 = Subtract(x=w324, y="Fixed Y-Range") -> (x-y=w326:dbl)
                n117 = property on="Property Node" class="WFChart (strict)"(reference=w335, "YScale.Maximum"=w330, "YScale.Minimum"=w331, "YScale.ScaleFit"=u8 0 ("Y Scale.Scale Fit")) -> ()  [unwired: 1 in, 2 out]
                n118 = property on="Property Node" class="WFChart (strict)"(reference=w333, "YScale.Maximum"=w325, "YScale.Minimum"=w326, "YScale.ScaleFit"=u8 0 ("Y Scale.Scale Fit")) -> ()  [unwired: 1 in, 2 out]
              }
            }
            n119 = property on="Fixed Y-Range" class="DigNum (strict)"("DisabledEnum"=w297) -> ()  [unwired: 2 in, 2 out]
          }
          frame #5 {
            w351 = T1 {"Set Temp"=0.0, "Read Temp"=23.7890625, "Package"="50", "Force"=0.0, "Feedback"=0} ("M1 Status")
            # "Display the status of M1 and M2 below the main page"
            n120 = Unbundle By Name(w352) -> ("Dataset.M1 Status.Set Temp"=w358:dbl, "Dataset.M1 Status.Package"=w357:string, "Dataset.M1 Status.Piston Force"=w356:dbl, "Dataset.M1 Status.Evap Temp"=w341:dbl, "Dataset.M1 Status.Case Temp"=w340:dbl, "Dataset.M1 Status.Intec Feedback"=w339:dbl, "Dataset.M1 Status.TSD Temp"=w338:dbl, "Dataset.M1 Status.Feedback"=w337:u8)
            n121 = Unbundle By Name(w352) -> ("Dataset.M2 Status.Set Temp"=w355:dbl, "Dataset.M2 Status.Package"=w354:string, "Dataset.M2 Status.Piston Force"=w353:dbl, "Dataset.M2 Status.Evap Temp"=w347:dbl, "Dataset.M2 Status.Case Temp"=w346:dbl, "Dataset.M2 Status.Intec Feedback"=w344:dbl, "Dataset.M2 Status.TSD Temp"=w342:dbl, "Dataset.M2 Status.Feedback"=w345:u8)
            n122 = case shown="2" w337 {
              tunnel: w341 -> [w359 _ _ _ _ _]
              tunnel: w340 -> [_ w360 _ _ _ _]
              tunnel: [w359 w360 w361 w362 nan nan] -> w336
              tunnel: w339 -> [_ _ w361 _ _ _]
              tunnel: w338 -> [_ _ _ w362 _ _]
              frame 0, Default {
                # "Evap Temp"
              }
              frame 1 {
                # "Case Temp"
              }
              frame 2 {
                # "intec Temp"
              }
              frame 3 {
                # "TSD"
              }
              frame 4 {
                # "Auto Tune"
              }
              frame 5 {
                # "Extra"
              }
            }
            n123 = case shown="4" w345 {
              tunnel: w347 -> [w365 _ _ _ _ _]
              tunnel: w346 -> [_ w366 _ _ _ _]
              tunnel: [w365 w366 w367 w368 nan nan] -> w343
              tunnel: w344 -> [_ _ w367 _ _ _]
              tunnel: w342 -> [_ _ _ w368 _ _]
              frame 0, Default {
                # "Evap Temp"
              }
              frame 1 {
                # "Case Temp"
              }
              frame 2 {
                # "intec Temp"
              }
              frame 3 {
                # "TSD"
              }
              frame 4 {
                # "Auto Tune"
              }
              frame 5 {
                # "Extra"
              }
            }
            n124 = Bundle By Name(cluster=w351, "Set Temp"=w358, "Package"=w357, "Force"=w356, "Read Temp"=w336, "Feedback"=w337) -> (→"M1 Data":T1)
            n125 = Bundle By Name(cluster=w351, "Set Temp"=w355, "Package"=w354, "Force"=w353, "Read Temp"=w343, "Feedback"=w345) -> (→"M2 Data":T1)
            n126 = Unbundle By Name(w352) -> ("Dataset.System Status.Power On Off"=→"Play/Pause" →"Comp":bool)
          }
          frame #6 {
            # "(°F - 32) × 5/9 => °C"
            # "Display module and sytem graphs on Graph tab"
            n127 = Unbundle By Name(w400) -> ("Dataset.M1 Status.AC Load Watts"=w372:dbl, "Dataset.M1 Status.Case Temp"=w396:dbl, "Dataset.M1 Status.Evap Temp"=w395:dbl, "Dataset.M1 Status.Heater %"=w394:dbl, "Dataset.M1 Status.EEV Steps"=w398:u32)
            n128 = Unbundle By Name(w400) -> ("Dataset.M2 Status.AC Load Watts"=w373:dbl, "Dataset.M2 Status.Case Temp"=w392:dbl, "Dataset.M2 Status.Evap Temp"=w391:dbl, "Dataset.M2 Status.Heater %"=w390:dbl, "Dataset.M2 Status.EEV Steps"=w388:u32)
            n129 = To Double Precision Float(number=w398) -> (double precision float=w397:dbl)
            n130 = To Double Precision Float(number=w388) -> (double precision float=w389:dbl)
            n131 = Unbundle By Name(w400) -> ("Dataset.System Status.Bypass Steps"=w382:u16, "Dataset.System Status.Discharge Temp"=w383:dbl, "Dataset.System Status.Liquid Temp"=w384:dbl, "Dataset.System Status.Suction Temp"=w385:dbl, "Dataset.System Status.Ambient Temp"=w386:dbl)
            n132 = Bundle By Name(cluster=T18 {"Case Temp"=0.0, "Evap Temp"=0.0, "Heater Power (%)"=0.0, "EEV Steps"=0.0, "AC Load(W)"=nan} ("M1 Temp Graphs"), "AC Load(W)"=w372, "Case Temp"=w396, "Evap Temp"=w395, "Heater Power (%)"=w394, "EEV Steps"=w397) -> (→"M1 Graphs":T18)
            n133 = Bundle By Name(cluster=T18 {"Case Temp"=0.0, "Evap Temp"=0.0, "Heater Power (%)"=0.0, "EEV Steps"=0.0, "AC Load(W)"=nan} ("M1 Temp Graphs"), "AC Load(W)"=w373, "Case Temp"=w392, "Evap Temp"=w391, "Heater Power (%)"=w390, "EEV Steps"=w389) -> (→"M2 Graphs":T18)
            n134 = local read "Graph Temp Unit"() -> (w374:bool)
            n135 = To Double Precision Float(number=w382) -> (double precision float=w380:dbl)
            n136 = case shown="True" w374 {
              tunnel: w383 -> [w404 w414]
              tunnel: w384 -> [w403 w413]
              tunnel: w385 -> [w402 w412]
              tunnel: w386 -> [w401 w411]
              tunnel: [w404 w408] -> w376
              tunnel: [w403 w407] -> w377
              tunnel: [w402 w406] -> w378
              tunnel: [w401 w405] -> w379
              frame False {
              }
              frame True {
                n137 = Build Array(w414, w413, w412, w411) -> (w410:dbl[])
                n138 = for {
                  tunnel: w410 -> [w421] mode=indexing
                  tunnel: [w415] -> w409 mode=indexing
                  n139 = Subtract(x=w421, y=32.0) -> (x-y=w419:dbl)
                  n140 = Divide(x=5.0, y=9.0) -> (x/y=w416:dbl)
                  n141 = Multiply(x=w419, y=w416) -> (x*y=w415:dbl)
                }
                n142 = Index Array(array=w409) -> (element #1=w408:dbl, element #2=w407:dbl, element #3=w406:dbl, element #4=w405:dbl)  [unwired: 4 in]
              }
            }
            n143 = Bundle By Name(cluster=T11 {"Ambient Temp"=0.0, "Suction Temp"=0.0, "Condensor Temp"=0.0, "Discharge Temp"=0.0, "Bypass Steps"=0.0} ("System Graphs"), "Bypass Steps"=w380, "Discharge Temp"=w376, "Condensor Temp"=w377, "Suction Temp"=w378, "Ambient Temp"=w379) -> (→"System Graphs":T11)
          }
          frame #7 {
            # "Buffer : 1hr (36000 samples)"
            n144 = Unbundle By Name(w423) -> ("Dataset.M2 Status"=w441:T31)
            n145 = Unbundle By Name(w423) -> ("Dataset.M1 Status"=w447:T31)
            n146 = Unbundle By Name(w423) -> ("M2 History Temps"=w433:dbl[][])
            n147 = Unbundle By Name(w441) -> ("Evap Temp"=w440:dbl, "Case Temp"=w439:dbl, "TSD Temp"=w438:dbl, "Set Temp"=w431:dbl)
            n148 = Unbundle By Name(w423) -> ("M1 History Temps"=w435:dbl[][])
            n149 = Unbundle By Name(w447) -> ("Evap Temp"=w444:dbl, "Case Temp"=w443:dbl, "TSD Temp"=w442:dbl, "Intec Feedback"=w424:dbl, "Set Temp"=w434:dbl)
            n150 = Build Array(w440, w439, w438) -> (w432:dbl[])
            n151 = Build Array(w444, w443, w442, w424) -> (w436:dbl[])
            n152 = case shown="False" "Average Graph" {
              tunnel: w436 -> [w464 w470]
              tunnel: w435 -> [w456 w471]
              tunnel: w434 -> [w463 w478]
              tunnel: w433 -> [w459 w476]
              tunnel: w432 -> [w460 w479]
              tunnel: w431 -> [w461 w477]
              tunnel: [w458 w475] -> w429
              tunnel: [w457 w474] -> w427
              tunnel: [w456 w469] -> w426
              tunnel: [w459 w473] -> w425
              frame False {
                n153 = Insert Into Array(array=w464, index=0, new element=w463) -> (w457:dbl[])
                n154 = Insert Into Array(array=w460, index=0, new element=w461) -> (w458:dbl[])
              }
              frame True {
                n155 = Build Array (concatenate)(w471, w470) -> (w469:dbl[][])
                n156 = Build Array (concatenate)(w476, w479) -> (w473:dbl[][])
                n157 = Transpose 2D Array(2D array=w469) -> (transposed array=w468:dbl[][])
                n158 = Transpose 2D Array(2D array=w473) -> (transposed array=w480:dbl[][])
                n159 = for {
                  tunnel: w468 -> [w483] mode=indexing
                  tunnel: [w486] -> w467 mode=indexing
                  n160 = Reverse 1D Array(array=w483) -> (reversed array=w482:dbl[])
                  n161 = Array Subset(array=w482, length=30) -> (w484:dbl[])  [unwired: 1 in]
                  n162 = call-poly <vilib>:"Mean.vi"("X"=w484) -> ("mean"=w486:dbl)  [unwired: 1 out]
                }
                n163 = for {
                  tunnel: w480 -> [w488] mode=indexing
                  tunnel: [w489] -> w472 mode=indexing
                  n164 = Reverse 1D Array(array=w488) -> (reversed array=w487:dbl[])
                  n165 = Array Subset(array=w487, length=30) -> (w490:dbl[])  [unwired: 1 in]
                  n166 = call-poly <vilib>:"Mean.vi"("X"=w490) -> ("mean"=w489:dbl)  [unwired: 1 out]
                }
                n167 = Insert Into Array(array=w467, index=0, new element=w478) -> (w474:dbl[])
                n168 = Insert Into Array(array=w472, index=0, new element=w477) -> (w475:dbl[])
              }
            }
            n169 = Get Date/Time In Seconds() -> (seconds since 1Jan1904=w428:timestamp)
            n170 = for {
              tunnel: [w451] -> w422 mode=indexing
              tunnel: w428 -> [w450]
              tunnel: w427 -> [w448] mode=indexing
              n171 = Build Array(w448) -> (w449:dbl[])
              n172 = Bundle By Name("Y"=w449, "t0"=w450) -> (w451:waveform(dbl))  [unwired: 1 in]
            }
            "M1 Main Waveform" <- w422
            n173 = for {
              tunnel: w428 -> [w454]
              tunnel: [w455] -> w430 mode=indexing
              tunnel: w429 -> [w452] mode=indexing
              n174 = Build Array(w452) -> (w453:dbl[])
              n175 = Bundle By Name("t0"=w454, "Y"=w453) -> (w455:waveform(dbl))  [unwired: 1 in]
            }
            "M2 Main Waveform" <- w430
            n176 = Bundle By Name(cluster=w446, "M1 History Temps"=w426, "M2 History Temps"=w425) -> (w445:T24)
          }
          frame #8 {
            # "Update M1 and M2 conmand module when both first call and chaged value"
            n177 = Unbundle By Name(w503) -> ("Dataset.M1 Status"=w510:T31, "Dataset.M1 Status.Head State"=w502:u16)
            n178 = Unbundle By Name(w503) -> ("Dataset.M2 Status"=w509:T31, "Dataset.M2 Status.Head State"=w498:u16)
            n179 = Unbundle By Name(w503) -> ("Dataset.Config Data.Packages.DUT Names"=w504:T44)
            n180 = Equal?(x=w498, y=enum16{"Disabled", "Run", "Error"}."Run" ("Dataset.M1 Status.Head State")) -> (x = y?=w497:bool)
            n181 = Equal?(x=w502, y=enum16{"Disabled", "Run", "Error"}."Run" ("Dataset.M1 Status.Head State")) -> (x = y?=w500:bool)
            n182 = Unbundle By Name(w509) -> ("Package"=w505:string, "Set Temp"=w506:dbl)
            n183 = Unbundle By Name(w510) -> ("Set Temp"=w508:dbl, "Package"=w507:string)
            n184 = property on="M2 Enable" class="Bool (strict)"("Value"=w497) -> ()  [unwired: 2 in, 2 out]
            n185 = property on="M1 Enable" class="Bool (strict)"("Value"=w500) -> ()  [unwired: 2 in, 2 out]
            n186 = Cluster To Array(cluster=w504) -> (array=w496:string[])
            n187 = Search 1D Array(1D array=w496, element=w505) -> (index of element=w493:i32)  [unwired: 1 in]
            n188 = Search 1D Array(1D array=w496, element=w507) -> (index of element=w495:i32)  [unwired: 1 in]
            n189 = To Unsigned Word Integer(number=w493) -> (unsigned 16bit integer=w492:u16)
            n190 = To Unsigned Word Integer(number=w495) -> (unsigned 16bit integer=w494:u16)
            n191 = local write "M1 Set Temp"(w508) -> ()
            n192 = local write "M1 Package"(w494) -> ()
            n193 = local write "M2 Package"(w492) -> ()
            n194 = local write "M2 Set Temp"(w506) -> ()
          }
          frame #9 {
            # "ETC"
            n195 = Unbundle By Name(w512) -> ("Dataset.Config Data.Packages.DUT Names"=w511:T44)
            n196 = Unbundle By Name(w512) -> ("Dataset.Config Data.Set Point Range"=w527:cluster{"Max":dbl, "Min":dbl})
            n197 = control-ref of="M1 Set Temp"() -> (w524:refnum<vi>)
            n198 = control-ref of="M2 Set Temp"() -> (w525:refnum<vi>)
            n199 = control-ref of="M1 Package"() -> (w523:refnum<vi>)
            n200 = control-ref of="M2 Package"() -> (w522:refnum<vi>)
            n201 = Build Array(w523, w522) -> (w521:refnum<vi>[])
            n202 = Build Array(w524, w525) -> (w526:refnum<vi>[])
            n203 = for {
              tunnel: w526 -> [w548] mode=indexing
              tunnel: w527 -> [w547]
              tunnel: w521 -> [w546] mode=indexing
              tunnel: w511 -> [w544]
              n204 = Unbundle By Name(w547) -> ("Max"=w549:dbl, "Min"=w550:dbl)
              n205 = Cluster To Array(cluster=w544) -> (array=w545:string[])
              n206 = property class="Ring (strict)"(reference=w546, "Strings []"=w545) -> ()  [unwired: 1 in, 2 out]
              n207 = property class="DigNum (strict)"(reference=w548, "Maximum"=w549, "Minimum"=w550) -> ()  [unwired: 1 in, 2 out]
            }
            n208 = disable-structure shown="Disabled" {
              frame Disabled {
                n209 = property on="AC Load(W)" class="WFChart (strict)"() -> ("YScale.ScaleFit"=w531:u8)  [unwired: 2 in, 2 out]
                n210 = Equal To 0?(x=w531) -> (x = 0?=w530:bool)
                n211 = case shown="True" w530 {
                  frame False {
                  }
                  frame True {
                    n212 = property on="AC Load(W)" class="WFChart (strict)"("YScale.Maximum"=800.0 ("Y Scale.Range:Maximum"), "YScale.Minimum"=0.0 ("Y Scale.Range:Minimum")) -> ()  [unwired: 2 in, 2 out]
                  }
                }
                n213 = property on="AC Load(W)" class="WFChart (strict)"() -> ("YScale.ScaleFit"=w528:u8)  [unwired: 2 in, 2 out]
                n214 = Equal To 0?(x=w528) -> (x = 0?=w529:bool)
                n215 = case shown="True" w529 {
                  frame False {
                  }
                  frame True {
                    n216 = property on="AC Load(W)" class="WFChart (strict)"("YScale.Maximum"=800.0 ("Y Scale.Range:Maximum"), "YScale.Minimum"=0.0 ("Y Scale.Range:Minimum")) -> ()  [unwired: 2 in, 2 out]
                  }
                }
              }
              frame Enabled {
                # "Jonathan asked customers would be able to set the y-scale"
              }
            }
            n217 = property on="EEV Steps" class="WFChart (strict)"() -> ("YScale.ScaleFit"=w518:u8)  [unwired: 2 in, 2 out]
            n218 = property on="Heater Power (%)" class="WFChart (strict)"() -> ("YScale.ScaleFit"=w520:u8)  [unwired: 2 in, 2 out]
            n219 = Equal To 0?(x=w518) -> (x = 0?=w517:bool)
            n220 = Equal To 0?(x=w520) -> (x = 0?=w519:bool)
            n221 = case shown="True" w519 {
              frame False {
              }
              frame True {
                n222 = property on="Heater Power (%)" class="WFChart (strict)"("YScale.Maximum"=100.0 ("Y Scale.Range:Maximum"), "YScale.Minimum"=0.0 ("Y Scale.Range:Minimum")) -> ()  [unwired: 2 in, 2 out]
              }
            }
            n223 = case shown="True" w517 {
              frame False {
              }
              frame True {
                n224 = property on="EEV Steps" class="WFChart (strict)"("YScale.Maximum"=600.0 ("Y Scale.Range:Maximum"), "YScale.Minimum"=0.0 ("Y Scale.Range:Minimum")) -> ()  [unwired: 2 in, 2 out]
              }
            }
            n225 = property on="EEV Steps" class="WFChart (strict)"() -> ("YScale.ScaleFit"=w514:u8)  [unwired: 2 in, 2 out]
            n226 = property on="Heater Power (%)" class="WFChart (strict)"() -> ("YScale.ScaleFit"=w516:u8)  [unwired: 2 in, 2 out]
            n227 = Equal To 0?(x=w514) -> (x = 0?=w513:bool)
            n228 = Equal To 0?(x=w516) -> (x = 0?=w515:bool)
            n229 = case shown="True" w513 {
              frame False {
              }
              frame True {
                n230 = property on="EEV Steps" class="WFChart (strict)"("YScale.Maximum"=600.0 ("Y Scale.Range:Maximum"), "YScale.Minimum"=0.0 ("Y Scale.Range:Minimum")) -> ()  [unwired: 2 in, 2 out]
              }
            }
            n231 = case shown="True" w515 {
              frame False {
              }
              frame True {
                n232 = property on="Heater Power (%)" class="WFChart (strict)"("YScale.Maximum"=100.0 ("Y Scale.Range:Maximum"), "YScale.Minimum"=0.0 ("Y Scale.Range:Minimum")) -> ()  [unwired: 2 in, 2 out]
              }
            }
          }
        }
      }
      frame "UI:Enable Tabs" {
        n233 = Variant To Data(error in=w560, type=i32[] [] ("Page array"), Variant=w559) -> (data=w552:i32[], error out=w551:errorcluster)
        n234 = control-ref of="Tab Control"() -> (w561:refnum<vi>)
        n235 = property class="TabCtl (strict)"(reference=w561) -> ("Pages"=w558:refnum<vi>[])  [unwired: 1 in, 2 out]
        n236 = Array Size(array=w552) -> (size(s)=w557:i32)
        n237 = Split 1D Array(array=w558, index=w557) -> (first subarray=w556:refnum<vi>[], second subarray=w555:refnum<vi>[])
        n238 = for {
          tunnel: w556 -> [w566] mode=indexing
          tunnel: T37."Page Enabled" ("Page Enabled State") -> [w567]
          n239 = property class="Page"(reference=w566, "PageEnb"=w567) -> ()  [unwired: 1 in, 2 out]
        }
        n240 = for {
          tunnel: w555 -> [w564] mode=indexing
          tunnel: T37."Page Disabled & Grayed" ("Page Enabled State") -> [w565]
          n241 = property class="Page"(reference=w564, "PageEnb"=w565) -> ()  [unwired: 1 in, 2 out]
        }
      }
      frame "UI:Enable Controls" {
        n242 = Variant To Data(error in=w582, type=T38."Supervisor" ("f"), Variant=w581) -> (data=w570:T38, error out=w568:errorcluster)
        n243 = case shown="Default" w570 {
          tunnel: [T36."Disabled and Grayed Out" ("Disabled") T36."Enabled" ("Disabled") T36."Enabled" ("Disabled")] -> w579
          tunnel: [FALSE ("Visible") TRUE ("Visible") w589] -> w571
          frame Default {
          }
          frame "Engineer" {
          }
          frame "Supervisor" {
            w589 = TRUE ("Visible")
            n244 = property on="Real Mode" class="Bool (strict)"("Visible"=w589) -> ()  [unwired: 2 in, 2 out]
            n245 = property on="Reboot RT" class="Bool (strict)"("Visible"=w589) -> ()  [unwired: 2 in, 2 out]
          }
        }
        n246 = control-ref of="?"() -> (w577:refnum<vi>)
        n247 = control-ref of="?"() -> (w576:refnum<vi>)
        n248 = control-ref of="?"() -> (w575:refnum<vi>)
        n249 = control-ref of="?"() -> (w574:refnum<vi>)
        n250 = control-ref of="?"() -> (w573:refnum<vi>)
        n251 = control-ref of="?"() -> (w572:refnum<vi>)
        n252 = property on="M1 EEV Manual" class="DigNum (strict)"("DisabledEnum"=w579) -> ()  [unwired: 2 in, 2 out]
        n253 = property on="M2 EEV Manual" class="DigNum (strict)"("DisabledEnum"=w579) -> ()  [unwired: 2 in, 2 out]
        n254 = property on="M1 Heater output" class="DigNum (strict)"("DisabledEnum"=w579) -> ()  [unwired: 2 in, 2 out]
        n255 = property on="M2 Heater Output" class="DigNum (strict)"("DisabledEnum"=w579) -> ()  [unwired: 2 in, 2 out]
        n256 = Build Array(w577, w576, w575, w574, w573, w572) -> (w578:refnum<vi>[])
        n257 = for {
          tunnel: w571 -> [w584]
          tunnel: w578 -> [w583] mode=indexing
          n258 = property class="DigNum (strict)"(reference=w583, "Visible"=w584) -> ()  [unwired: 1 in, 2 out]
        }
        n259 = property on="Configure" class="Bool"("Visible"=w571) -> ()  [unwired: 2 in, 2 out]
        n260 = property on="Subcool" class="Knob (strict)"("Visible"=w571) -> ()  [unwired: 2 in, 2 out]
        n261 = property on="Superheat" class="Knob (strict)"("Visible"=w571) -> ()  [unwired: 2 in, 2 out]
      }
      frame "UI:Visible Controls" {
        n262 = stacked-sequence {
          tunnel: [w595 _] -> w591
          tunnel: w592 -> [w599 w609]
          tunnel: w593 -> [w601 w606]
          frame #0 {
            # "Module#2 Page makes disable"
            n263 = Unbundle By Name(w599) -> ("M2 Bootup"=w594:bool)
            n264 = Select(t=T37."Page Enabled" ("Page Enabled State"), s=w594, f=T37."Page Disabled & Grayed" ("Page Enabled State")) -> (s? t:f=w596:T37)
            n265 = control-ref of="Graph Tab CTL"() -> (w603:refnum<vi>)
            n266 = property class="TabCtl (strict)"(reference=w603, error in=w601) -> (error out=w600:errorcluster, "Pages"=w604:refnum<vi>[])  [unwired: 1 out]
            n267 = Index Array(array=w604, index=1) -> (element=w605:refnum<vi>)
            n268 = property class="Page"(reference=w605, error in=w600, "PageEnb"=w596) -> (error out=w595:errorcluster)  [unwired: 1 out]
          }
          frame #1 {
            # "Visibility of Tab Control"
            n269 = control-ref of="Tab Control"() -> (w612:refnum<vi>)
            n270 = Unbundle By Name(w609) -> ("System Ready"=w608:bool, "M2 Bootup"=w607:bool)
            n271 = property class="TabCtl (strict)"(reference=w612, error in=w606) -> (error out=w610:errorcluster, "Pages"=w611:refnum<vi>[])  [unwired: 1 out]
            n272 = for {
              tunnel: w611 -> [w619] mode=indexing
              tunnel: w610 -> [w617]
              tunnel: w607 -> [w615]
              tunnel: w608 -> [w614]
              tunnel: [w613] -> _
              n273 = property class="Page"(reference=w619, error in=w617) -> (error out=w616:errorcluster, "ControlsOnPage"=w618:refnum<vi>[])  [unwired: 1 out]
              n274 = for {
                tunnel: w618 -> [w630] mode=indexing
                tunnel: w616 -> [w629]
                tunnel: w615 -> [w628]
                tunnel: w614 -> [w627]
                tunnel: [w626] -> w613
                n275 = property class="Ctl"(reference=w630, error in=w629) -> (reference out=w624:refnum<vi>, error out=w623:errorcluster, "Label.Text"=w621:string)
                n276 = Scan From String(format string="%s", input string=w621) -> (output 1=w622:string)  [unwired: 3 in, 3 out]
                n277 = case shown="Default" w622 {
                  tunnel: w627 -> [w631 _]
                  tunnel: w628 -> [_ w632]
                  tunnel: [w631 w632] -> w620
                  frame Default {
                  }
                  frame "M2" {
                  }
                }
                n278 = property class="Ctl"(reference=w624, error in=w623, "Visible"=w620) -> (error out=w626:errorcluster)  [unwired: 1 out]
              }
            }
          }
        }
      }
      frame "UI:Refresh Graph" {
        w641 = 0.0 ("M1 Heater output")
        w642 = u16 0 ("M1 EEV Manual")
        w645 = dbl[][] [] ("M1 Original Temps")
        w653 = waveform(dbl)[][] [] ("M1 Main Waveform")
        n279 = Variant To Data(error in=w663, type="", Variant=w662) -> (data=w639:string, error out=w648:errorcluster)
        n280 = control-ref of="Ambient Temp"() -> (w655:refnum<vi>)
        n281 = Format Into String(format string="(%s)", initial string="Superheat" ("Command"), w639) -> (resulting string=w637:string)  [unwired: 1 in, 1 out]
        n282 = Format Into String(format string="(%s)", initial string="Subcool" ("Command"), w639) -> (resulting string=w638:string)  [unwired: 1 in, 1 out]
        n283 = Format Into String(format string="(%s)", initial string="Temperature" ("Command"), w639) -> (resulting string=w656:string)  [unwired: 1 in, 1 out]
        n284 = property on="Subcool" class="Knob (strict)"("Caption.Text"=w638) -> ()  [unwired: 2 in, 2 out]
        n285 = property on="Superheat" class="Knob (strict)"("Caption.Text"=w637) -> ()  [unwired: 2 in, 2 out]
        n286 = property class="WFChart (strict)"(reference=w655, "YScale.NameLbl.Text"=w656) -> ()  [unwired: 1 in, 2 out]
        n287 = control-ref of="System Graphs"() -> (w649:refnum<vi>)
        n288 = control-ref of="M1 Graphs"() -> (w652:refnum<vi>)
        n289 = control-ref of="M2 Graphs"() -> (w651:refnum<vi>)
        n290 = Build Array(w652, w651, w649) -> (w650:refnum<vi>[])
        n291 = property on="M1 Humidity" class="WFChart (strict)"(error in=w648, "History Data"=cluster{"M1 RH":dbl, "RH Threshold":dbl}[] []) -> (error out=w647:errorcluster)  [unwired: 1 in, 1 out]
        n292 = for {
          tunnel: w650 -> [w667] mode=indexing
          n293 = property class="Clust (strict)"(reference=w667) -> ("Controls[]"=w665:refnum<vi>[])  [unwired: 1 in, 2 out]
          n294 = for {
            tunnel: dbl[] [] ("History Data") -> [w671]
            tunnel: w665 -> [w670] mode=indexing
            tunnel: refnum<vi> refnum ("M1 Heater Power (%)") -> [w668]
            n295 = To More Specific Class(target class=w668, reference=w670) -> (specific class reference=w669:refnum<vi>)  [unwired: 1 in, 1 out]
            n296 = property class="WFChart (strict)"(reference=w669, "History Data"=w671) -> ()  [unwired: 1 in, 2 out]
          }
        }
        n297 = property on="M2 Main Waveform" class="WFChart (strict)"(error in=w647, "History Data"=w653) -> (error out=w654:errorcluster)  [unwired: 1 in, 1 out]
        n298 = property on="M1 Main Waveform" class="WFChart (strict)"(error in=w654, "History Data"=w653) -> (error out=w640:errorcluster)  [unwired: 1 in, 1 out]
        n299 = property on="M1 EEV Manual" class="DigNum (strict)"("Value"=w642) -> ()  [unwired: 2 in, 2 out]
        n300 = property on="M2 EEV Manual" class="DigNum (strict)"("Value"=w642) -> ()  [unwired: 2 in, 2 out]
        n301 = property on="M1 Heater output" class="DigNum (strict)"("Value"=w641) -> ()  [unwired: 2 in, 2 out]
        n302 = property on="M2 Heater Output" class="DigNum (strict)"("Value"=w641) -> ()  [unwired: 2 in, 2 out]
        n303 = property on="Manual Bypass Mode" class="Arr (strict)"(error in=w640, "Value"=bool[] [] ("Manual Bypass Mode")) -> (error out=w643:errorcluster)  [unwired: 1 in, 1 out]
        n304 = Bundle By Name(cluster=w660, "M1 History Temps"=w645, "M2 History Temps"=w645) -> (w661:T24)
      }
      frame "UI:M2 Enable Controls" {
        n305 = Unbundle By Name(w679) -> ("Reboot"=w672:bool, "Last Connected System"=w681:enum16{"Single Head", "Duel Head"})
        n306 = Unbundle By Name(w679) -> ("Dataset.M2 Status.Case Temp"=w693:dbl, "Dataset.M2 Status.Evap Temp"=w692:dbl)
        n307 = Unbundle By Name(w679) -> ("Real Mode"=w685:bool)
        n308 = Equal?(x=w681, y=enum16{"Single Head", "Duel Head"}."Duel Head") -> (x = y?=w680:bool)
        n309 = Not Equal To 0?(x=w693) -> (x != 0?=w691:bool)
        n310 = Not Equal To 0?(x=w692) -> (x != 0?=w690:bool)
        n311 = And(x=w672, y=w680) -> (x .and. y?=w674:bool)
        n312 = Compound Arithmetic op=AND(w691, w690) -> (w684:bool)
        n313 = Select(t=w684, s=w685, f=TRUE) -> (s? t:f=w676:bool)
        n314 = case shown="True" w676 {
          selector: w676 -> [_ w709]
          tunnel: w674 -> [w700 _]
          tunnel: [w697 "MACRO:Display Panel" ("Command")] -> w678
          tunnel: [w699 enum16{"Single Head", "Duel Head"}."Duel Head" ("Last Connected System")] -> w673
          tunnel: [w698 w709] -> w675
          frame False {
            n315 = case shown="False" w700 {
              selector: w700 -> [w702 w705]
              tunnel: [enum16{"Single Head", "Duel Head"}."Single Head" ("Last Connected System") enum16{"Single Head", "Duel Head"}."Duel Head" ("Last Connected System")] -> w699
              tunnel: [w702 w705] -> w698
              tunnel: ["MACRO:Display Panel" ("Command") "NS:Read\nUI:M2 Enable Controls" ("Command")] -> w697
              frame False {
              }
              frame True {
              }
            }
          }
          frame True {
          }
        }
        n316 = call "Messaging EnQ Multiline String.vi"("Command(s)"=w678, "error in (no error)"=w677) -> ("error out"=w686:errorcluster)  [unwired: 9 in]
        n317 = stacked-sequence {
          tunnel: w675 -> [w710 w717]
          frame #0 {
            n318 = property on="M1 Enable" class="Bool (strict)"("Visible"=w710) -> ()  [unwired: 2 in, 2 out]
            n319 = property on="M2 Data" class="Clust (strict)"("Visible"=w710) -> ()  [unwired: 2 in, 2 out]
            n320 = Select(t=u32 4 ("Number of Rows"), s=w710, f=u32 2 ("Number of Rows")) -> (s? t:f=w713:u32)
            n321 = property on="Manual Bypass Mode" class="Arr (strict)"("Number of Rows"=w713) -> ()  [unwired: 2 in, 2 out]
          }
          frame #1 {
            n322 = Select(t=u32 239 ("Plot Area:Size:Height"), s=w717, f=u32 530 ("Plot Area:Size:Height")) -> (s? t:f=w720:u32)
            n323 = property on="M1 Main Waveform" class="WFChart (strict)"("Height"=w720) -> ()  [unwired: 2 in, 2 out]
            n324 = property on="Event Tab" class="TabCtl (strict)"("Value"=enum32{"Cobra Events", "GUI Events"}."Cobra Events" ("Event Tab")) -> ()  [unwired: 2 in, 2 out]
            n325 = property on="Tab Control" class="TabCtl (strict)"("Value"=T6."Controls" ("Tab Control")) -> ()  [unwired: 2 in, 2 out]
            n326 = property on="Graph Tab CTL" class="TabCtl (strict)"("Value"=enum32{"Head #1", "Head #2"}."Head #1" ("Graph Tab CTL")) -> ()  [unwired: 2 in, 2 out]
          }
        }
        n327 = case shown="True" w675 {
          tunnel: [w723 w727] -> w695
          tunnel: [T39 {"Left"=1915, "Top"=190} ("Position") T39 {"Left"=2890, "Top"=-70} ("Position")] -> w696
          tunnel: [w723 w727] -> w694
          tunnel: [T39 {"Left"=2900, "Top"=-20} ("Position") T39 {"Left"=1930, "Top"=40} ("Position")] -> w688
          tunnel: [T39 {"Left"=2880, "Top"=-43} ("Position") T39 {"Left"=1905, "Top"=20} ("Position")] -> w687
          frame False {
            w723 = T39 {"Left"=1880, "Top"=150} ("Position")
          }
          frame True {
            w727 = T39 {"Left"=2850, "Top"=-110} ("Position")
          }
        }
        n328 = property on="M1 Power Drive Control" class="Bool (strict)"("Position"=w696) -> ()  [unwired: 2 in, 2 out]
        n329 = property on="M1 Power Drive Indicator" class="Bool"("Position"=w695) -> ()  [unwired: 2 in, 2 out]
        n330 = property on="M1 Safe Temp and Head State" class="Bool (strict)"("Position"=w694) -> ()  [unwired: 2 in, 2 out]
        n331 = property on="Power On-Off" class="Bool (strict)"("Position"=w688) -> ()  [unwired: 2 in, 2 out]
        n332 = property on="Play/Pause" class="Bool"("Position"=w687) -> ()  [unwired: 2 in, 2 out]
        n333 = Bundle By Name(cluster=w679, "Last Connected System"=w673, "M2 Bootup"=w675) -> (w689:T24)
      }
      frame "UI:Update Network Down Data" {
        # "Keep RT status if not change"
        n334 = Unbundle By Name(w729) -> ("Dataset"=w739:T29)
        n335 = Unbundle By Name(w729) -> ("Dataset.Config Data.Packages.DUT Names"=w742:T44)
        n336 = Unbundle By Name(w739) -> ("System Status.Power On Off"=w737:bool, "Config Data"=w738:T32, "System Status.M1 Actuated"=w732:bool, "M1 Status"=w733:T31)
        n337 = Unbundle By Name(w733) -> ("Set Temp"=w736:dbl, "Power Drive"=w735:bool, "Feedback"=w734:u8, "Package"=w743:string)
        n338 = Cluster To Array(cluster=w742) -> (array=w741:string[])
        n339 = Search 1D Array(1D array=w741, element=w743) -> (index of element=w744:i32)  [unwired: 1 in]
        n340 = Bundle By Name(cluster=T40 {"Set Temp"=0.0, "Power Drive"=FALSE, "Feedback"=0, "Package"=0, "Enable"=FALSE} ("Network Data Down.M1 Commands"), "Enable"=w732, "Set Temp"=w736, "Power Drive"=w735, "Feedback"=w734, "Package"=w744) -> (w731:T40)
        n341 = Bundle By Name(cluster=w729, "Network Data Down.System Power On Off"=w737, "Network Data Down.Config Data"=w738, "Network Data Down.M1 Commands"=w731) -> (w730:T24)
      }
      frame "UI:Module Enable" {
        n342 = Unbundle By Name(w762) -> ("Dataset.M1 Status.Case Temp"=w764:dbl, "Dataset.M1 Status.Evap Temp"=w765:dbl)
        n343 = Unbundle By Name(w762) -> ("Real Mode"=w749:bool, "Network Connection"=w753:bool)
        n344 = Not Equal To 0?(x=w764) -> (x != 0?=w766:bool)
        n345 = Not Equal To 0?(x=w765) -> (x != 0?=w767:bool)
        n346 = Compound Arithmetic op=AND(w766, w767) -> (w748:bool)
        n347 = Select(t=w748, s=w749, f=TRUE) -> (s? t:f=w746:bool)
        n348 = Select(t=T36."Enabled" ("Disabled"), s=w746, f=T36."Disabled" ("Disabled")) -> (s? t:f=w757:T36)
        n349 = Not(x=w746) -> (.not. x?=w758:bool)
        n350 = property on="System Ready" class="Bool (strict)"("Blinking"=w758, "Value"=w746, "DisabledEnum"=w757) -> ()  [unwired: 2 in, 2 out]
        n351 = Select(t="NS:Read\nUI:Reinitialize Front Panel\nUI:Module Enable" ("Command"), s=w753, f="NS:Open Connection" ("Command")) -> (s? t:f=w763:string)
        n352 = Select(t="NS:Read\nUI:M2 Enable Controls" ("Command"), s=w746, f=w763) -> (s? t:f=w752:string)
        n353 = call "Messaging EnQ Multiline String.vi"("Command(s)"=w752, "error in (no error)"=w751) -> ("error out"=w750:errorcluster)  [unwired: 9 in]
        n354 = Bundle By Name(cluster=w762, "System Ready"=w746) -> (w754:T24)
      }
      frame "UI:Reinitialize Front Panel" {
        # "Visible or Invisible Components in Front Panel"
        n355 = Unbundle By Name(w779) -> ("System Ready"=w772:bool, "M2 Bootup"=w776:bool, "Core.Current VI"=w777:refnum<vi>)
        n356 = property class="VI"(reference=w777, error in=w778) -> (error out=w783:errorcluster, "Panel"=w780:refnum<vi>)  [unwired: 1 out]
        n357 = property class="Pnl"(reference=w780, error in=w783) -> (error out=w782:errorcluster, "Controls[]"=w781:refnum<vi>[])  [unwired: 1 out]
        n358 = for {
          tunnel: w781 -> [w793] mode=indexing
          tunnel: w782 -> [w794]
          tunnel: w772 -> [w790]
          tunnel: w776 -> [w789]
          tunnel: [w786] -> w774
          n359 = property class="Ctl"(reference=w793, error in=w794) -> (reference out=w791:refnum<vi>, error out=w792:errorcluster, "Label.Text"=w788:string)
          n360 = case shown="Default" w788 {
            selector: w788 -> [_ w800]
            tunnel: [w795 w803] -> w787
            tunnel: w792 -> [w795 w803]
            tunnel: w791 -> [w796 w798]
            tunnel: w790 -> [_ w802]
            tunnel: w789 -> [_ w801]
            tunnel: [TRUE ("Network Connection") w799] -> w785
            tunnel: [w796 w798] -> w784
            frame "Net Cluster" {
            }
            frame Default {
              n361 = Scan From String(format string="%s", input string=w800) -> (output 1=w805:string)  [unwired: 3 in, 3 out]
              n362 = case shown="Default" w805 {
                tunnel: [w806 w807] -> w799
                tunnel: w802 -> [w806 _]
                tunnel: w801 -> [_ w807]
                frame Default {
                }
                frame "M2" {
                }
              }
            }
          }
          n363 = property class="Ctl"(reference=w784, error in=w787, "Visible"=w785) -> (error out=w786:errorcluster)  [unwired: 1 out]
        }
        n364 = Not(x=w772) -> (.not. x?=w775:bool)
        n365 = Select(t=T36."Enabled" ("Disabled"), s=w772, f=T36."Disabled" ("Disabled")) -> (s? t:f=w769:T36)
        n366 = property on="System Ready" class="Bool (strict)"(error in=w774, "Blinking"=w775, "Value"=w772, "DisabledEnum"=w769) -> (error out=w773:errorcluster)  [unwired: 1 in, 1 out]
      }
      frame "UI:Visibility" {
        n367 = stacked-sequence {
          tunnel: w809 -> [w829 w845 w862]
          frame #0 {
            n368 = Unbundle By Name(w829) -> ("Dataset.System Status.Compressor Amps"=w830:dbl, "Dataset.System Status.Power On Off"=w825:bool, "Dataset.Config Data.System Settings.Cascade"=w831:bool)
            n369 = Unbundle By Name(w829) -> ("System Ready"=w818:bool, "M2 Bootup"=w812:bool)
            n370 = local read "M2 Channels"() -> (w816:dbl[])
            n371 = Index Array(array=w816, index=3) -> (element=w814:dbl)
            n372 = local read "M1 Channels"() -> (w823:dbl[])
            n373 = Not A Number/Path/Refnum?(number/path/refnum=w814) -> (NaN/Path/Refnum?=w815:bool)
            n374 = Not(x=w815) -> (.not. x?=w817:bool)
            n375 = Round To Nearest(number=w830) -> (nearest integer value=w832:dbl)
            n376 = And(x=w812, y=w817) -> (x .and. y?=w810:bool)
            n377 = Not Equal To 0?(x=w832) -> (x != 0?=w828:bool)
            n378 = property on="M2 TSD Feedback" class="Bool (strict)"("Visible"=w810) -> ()  [unwired: 2 in, 2 out]
            n379 = Index Array(array=w823, index=3) -> (element=w822:dbl)
            n380 = Not A Number/Path/Refnum?(number/path/refnum=w822) -> (NaN/Path/Refnum?=w821:bool)
            n381 = Not(x=w821) -> (.not. x?=w820:bool)
            n382 = And(x=w820, y=w818) -> (x .and. y?=w811:bool)
            n383 = And(x=w825, y=w831) -> (x .and. y?=w824:bool)
            n384 = property on="M1 TSD Feedback" class="Bool (strict)"("Visible"=w811) -> ()  [unwired: 2 in, 2 out]
            n385 = property on="High Side RPM" class="DigNum (strict)"("Visible"=w824) -> ()  [unwired: 2 in, 2 out]
            n386 = property on="Low Side RPM" class="DigNum (strict)"("Visible"=w824) -> ()  [unwired: 2 in, 2 out]
            n387 = property on="Cascade Compressor controls" class="Clust (strict)"("Visible"=w824) -> ()  [unwired: 2 in, 2 out]
            n388 = Compound Arithmetic op=AND(w812, w828, w825) -> (w826:bool)
            n389 = Compound Arithmetic op=AND(w818, w828, w825) -> (w827:bool)
            n390 = property on="M1 Thermal State" class="Enum (strict)"("Visible"=w827) -> ()  [unwired: 2 in, 2 out]
            n391 = property on="M2 Thermal State" class="Enum (strict)"("Visible"=w826) -> ()  [unwired: 2 in, 2 out]
          }
          frame #1 {
            n392 = Unbundle By Name(w845) -> ("System Ready"=w841:bool, "M2 Bootup"=w835:bool)
            n393 = local read "M1 Channels"() -> (w844:dbl[])
            n394 = local read "M2 Channels"() -> (w836:dbl[])
            n395 = Index Array(array=w844, index=4) -> (element=w843:dbl)
            n396 = Index Array(array=w836, index=4) -> (element=w837:dbl)
            n397 = Not A Number/Path/Refnum?(number/path/refnum=w843) -> (NaN/Path/Refnum?=w839:bool)
            n398 = Not A Number/Path/Refnum?(number/path/refnum=w837) -> (NaN/Path/Refnum?=w834:bool)
            n399 = And(x=w835, y=w834) -> (x .and. y?=w833:bool)
            n400 = And(x=w839, y=w841) -> (x .and. y?=w840:bool)
            n401 = case shown="True" w833 {
              frame False {
              }
              frame True {
                w846 = u32 4 ("Active Plot")
                n402 = property on="M2 Main Waveform" class="WFChart (strict)"("Active Plot"=w846, "LegNumRows"=w846) -> ()  [unwired: 2 in, 2 out]
                n403 = property on="M1 Channels" class="Arr (strict)"("Number of Rows"=w846) -> ()  [unwired: 2 in, 2 out]
              }
            }
            n404 = case shown="True" w840 {
              frame False {
              }
              frame True {
                w847 = u32 4 ("Active Plot")
                n405 = property on="M1 Channels" class="Arr (strict)"("Number of Rows"=w847) -> ()  [unwired: 2 in, 2 out]
                n406 = property on="M1 Main Waveform" class="WFChart (strict)"("Active Plot"=w847, "LegNumRows"=w847) -> ()  [unwired: 2 in, 2 out]
              }
            }
          }
          frame #2 {
            # "Disable"
            # "Disable"
            n407 = Unbundle By Name(w862) -> ("Dataset.M2 Status.Head State"=w851:u16, "Dataset.Config Data.Piston Settings.Diameter (mm)"=w866:dbl, "Dataset.M2 Status.Safe Temp"=w859:bool, "Dataset.Config Data.Safe Temps.Enabled"=w856:bool, "M2 Bootup"=w855:bool)
            n408 = Unbundle By Name(w862) -> ("System Ready"=w854:bool, "Dataset.Config Data.Safe Temps.Enabled"=w860:bool, "Dataset.M1 Status.Safe Temp"=w861:bool, "Dataset.Config Data.Piston Settings.Diameter (mm)"=w867:dbl, "Dataset.M1 Status.Head State"=w849:u16)
            n409 = Equal To 0?(x=w851) -> (x = 0?=w850:bool)
            n410 = Greater Than 0?(x=w866) -> (x > 0?=w865:bool)
            n411 = Equal To 0?(x=w849) -> (x = 0?=w848:bool)
            n412 = Greater Than 0?(x=w867) -> (x > 0?=w868:bool)
            n413 = Compound Arithmetic op=AND(w859, w856, w855) -> (w852:bool)
            n414 = Compound Arithmetic op=AND(w854, w860, w861) -> (w853:bool)
            n415 = property on="M2 Safe Temp and Head State" class="Bool (strict)"("Value"=w850, "Visible"=w852) -> ()  [unwired: 2 in, 2 out]
            n416 = Not(x=w853) -> (.not. x?=w864:bool)
            n417 = Not(x=w852) -> (.not. x?=w863:bool)
            n418 = property on="M1 Safe Temp and Head State" class="Bool (strict)"("Visible"=w853, "Value"=w848) -> ()  [unwired: 2 in, 2 out]
            n419 = Compound Arithmetic op=AND(w865, w863, w855) -> (w857:bool)
            n420 = Compound Arithmetic op=AND(w854, w864, w868) -> (w858:bool)
            n421 = property on="M2 Power Drive Indicator" class="Bool"("Visible"=w857) -> ()  [unwired: 2 in, 2 out]
            n422 = property on="M2 Power Drive Control" class="Bool (strict)"("Visible"=w857) -> ()  [unwired: 2 in, 2 out]
            n423 = property on="M1 Power Drive Control" class="Bool (strict)"("Visible"=w858) -> ()  [unwired: 2 in, 2 out]
            n424 = property on="M1 Power Drive Indicator" class="Bool"("Visible"=w858) -> ()  [unwired: 2 in, 2 out]
          }
        }
      }
      frame "-----MACRO-----" {
        # "MACRO is used for groups of cases that need to be run together."
      }
      frame "MACRO:Initialize" {
        # "1. Initialize Core Data\n2. Set Front Panel State\n3. Detect the available systems"
        # "3."
        # "2."
        # "1."
        # "Send initialize sequence of commands"
        n425 = Variant To Data(error in=w889, type=TRUE ("Log Events?"), Variant=w887) -> (data=w885:bool, error out=w888:errorcluster)
        n426 = call "Messaging EnQ Single.vi"("Command"="SYS:Initialize", "error in (no error)"=w888) -> ("error out"=w881:errorcluster)  [unwired: 9 in]
        n427 = Select(t="Open", s=w885, f="Close") -> (s? t:f=w882:string)
        n428 = Format Into String(format string="UI:Front Panel State>>%s" ("Command"), w882) -> (resulting string=w890:string)  [unwired: 2 in, 1 out]
        n429 = call "Messaging EnQ Single.vi"("Command"=w890, "error in (no error)"=w881) -> ("error out"=w879:errorcluster)  [unwired: 9 in]
        n430 = call "Messaging EnQ Single.vi"("Command"="UI:Reinitialize Front Panel", "error in (no error)"=w879) -> ("error out"=w878:errorcluster)  [unwired: 9 in]
        n431 = call "Messaging EnQ Single.vi"("Command"="NS:Detect Systems", "error in (no error)"=w878) -> ("error out"=w872:errorcluster)  [unwired: 9 in]
        n432 = To Variant(anything=T38."Operator" ("f")) -> (Variant=w875:variant)
        n433 = call "Messaging EnQ Single.vi"("Command"="DB:Login", "Data"=w875, "error in (no error)"=w872) -> ("error out"=w871:errorcluster)  [unwired: 8 in]
      }
      frame "MACRO:NS Update" {
        n434 = call "Messaging EnQ Single.vi"("Command"="NS:Update IP", "Data"=w902, "error in (no error)"=w901) -> ("error out"=w896:errorcluster)  [unwired: 8 in]
        n435 = Unbundle By Name(w894) -> ("Test"=w893:bool)
        n436 = case shown="True" w893 {
          tunnel: w896 -> [w903 w907]
          tunnel: [w903 w906] -> w895
          frame False {
          }
          frame True {
            n437 = call "Messaging EnQ Single.vi"("Command"="APP:Test", "Data"=FALSE, "error in (no error)"=w907) -> ("error out"=w906:errorcluster)  [unwired: 8 in]
          }
        }
        n438 = call "Messaging EnQ Multiline String.vi"("Command(s)"="NS:Close Connection\nUI:Reinitialize Front Panel\nNS:Open Connection", "error in (no error)"=w895) -> ("error out"=w900:errorcluster)  [unwired: 9 in]
        n439 = disable-structure shown="Disabled" {
          disable-tunnel: w900 -> [w910 _]
          disable-tunnel: [w908 _] -> w899
          frame Disabled {
            n440 = call "Messaging EnQ Single.vi"("Command"="TCP:Close Connection", "error in (no error)"=w910) -> ("error out"=w908:errorcluster)  [unwired: 9 in]
          }
          frame Enabled {
          }
        }
      }
      frame "MACRO:Display Panel" {
        w911 = FALSE ("Reboot")
        n441 = call "Messaging EnQ Single.vi"("Command"="UI:Visible Controls", "error in (no error)"=w915) -> ("error out"=w916:errorcluster)  [unwired: 9 in]
        n442 = To Variant(anything="°F" ("Command")) -> (Variant=w923:variant)
        n443 = call "Messaging EnQ Single.vi"("Command"="UI:Refresh Graph", "Data"=w923, "error in (no error)"=w916) -> ("error out"=w920:errorcluster)  [unwired: 8 in]
        n444 = Unbundle By Name(w913) -> ("User"=w926:T38)
        n445 = To Variant(anything=w926) -> (Variant=w922:variant)
        n446 = call "Messaging EnQ Single.vi"("Command"="UI:Enable Controls", "Data"=w922, "error in (no error)"=w920) -> ("error out"=w918:errorcluster)  [unwired: 8 in]
        n447 = call "Messaging EnQ Single.vi"("Command"="UI:Reinitialize Front Panel" ("Command(s)"), "error in (no error)"=w918) -> ("error out"=w914:errorcluster)  [unwired: 9 in]
        n448 = Bundle By Name(cluster=w913, "Reboot"=w911) -> (w912:T24)
        n449 = property on="Reboot RT" class="Bool (strict)"("Value"=w911) -> ()  [unwired: 2 in, 2 out]
      }
      frame "MACRO:Shutdown" {
        # "Shutdown Process\n1. Stop Event Loop\n2. Stop Test\n3. Disconnection of Network Stream\n4. Disconnection of Network Shared Variable\n5. Disconnection of TCP\n6. Close Front Panel\n7. Logging, Stop Queue, and Exit"
        # "List of commands to send for shutting down."
        n450 = call "Messaging EnQ Single.vi"("Command"="APP:Test", "Data"=FALSE ("Test"), "error in (no error)"=w930) -> ("error out"=w928:errorcluster)  [unwired: 8 in]
        n451 = call "Messaging EnQ Multiline String.vi"("Command(s)"="NS:Close Connection\nUI:Front Panel State>>Close\nSYS:Exit", "error in (no error)"=w928) -> ("error out"=w934:errorcluster)  [unwired: 9 in]
      }
      frame "------Network Stream------" {
        # "Deals with the Shared Variable Engine interface (network Streams)"
      }
      frame "NS:Detect Systems" {
        w939 = u32 0 items=["none"=0, "only if online"=1, "all"=3] ("Include Cached Results (all)")
        w940 = u32 18 items=["Hostname"=16, "Hostname (IP)"=18, "Hostname (MAC)"=19, "IP"=32, "IP (Hostname)"=33, "IP (MAC)"=35, "MAC"=48, "MAC (Hostname)"=49, "MAC (IP)"=50] ("Output (Hostname and IP)")
        n452 = call <vilib>:"Find Systems.vi"("error in (no error)"=w946, "Output (Hostname and IP)"=w940, "Include Cached Results (all)"=w939) -> ("error out"=w943:errorcluster, "Detected Systems"=w941:string[])  [unwired: 6 in, 1 out]
        "Detected Systems" <- w941
        n453 = property on="Menu Ring" class="Ring (strict)"(error in=w943, "Strings []"=w941, "Val(Sgnl)"=u16 0 ("Value (Signaling)")) -> (error out=w942:errorcluster)  [unwired: 1 in, 1 out]
        n454 = Bundle By Name(cluster=w945, "Detected Systems"=w941) -> (w944:T24)
      }
      frame "NS:Update IP" {
        (unwired) "CFX315" ("format string")
        n455 = Unbundle By Name(w953) -> ("Dataset.M1 Status.Package"=w948:string, "Detected Systems"=w951:string[])
        n456 = Variant To Data(error in=w957, type=0, Variant=w956) -> (data=w952:i32, error out=w950:errorcluster)
        n457 = Index Array(array=w951, index=w952) -> (element=w947:string)
        n458 = disable-structure shown="Enabled" {
          disable-tunnel: [w966 w969] -> w955
          disable-tunnel: w953 -> [w965 w970]
          disable-tunnel: w950 -> [w963 w972]
          disable-tunnel: [w962 w971] -> w949
          disable-tunnel: w948 -> [w961 _]
          disable-tunnel: w947 -> [w958 w967]
          frame Disabled {
            n459 = call "Update IP Address.vi"("error in"=w963, "Detected System"=w958, "Package Name"=w961) -> ("error out"=w962:errorcluster, "Shared Variable Address"=w959:string, "IP Address"=w960:string)  [unwired: 6 in]
            n460 = Bundle By Name(cluster=w965, "Connected System"=w958, "IP Address"=w960, "Shared Variable Address"=w959, "URI Directory"="/C/TTV Test Patterns/" ("relative uri")) -> (w966:T24)
          }
          frame Enabled {
            n461 = xnode "Match Regular Expression"("input string"=w967, "regular expression"="\\b[0-9]+\\.[0-9]+\\.[0-9]+\\.[0-9]+", "error in"=w972) -> ("whole match"=w968:string, "error out"=w971:errorcluster)  [unwired: 3 in, 3 out]
            n462 = Bundle By Name(cluster=w970, "Connected System"=w967, "IP Address"=w968) -> (w969:T24)
          }
        }
      }
      frame "NS:Open Connection" {
        n463 = Unbundle By Name(w1091) -> ("IP Address"=w1103:string)
        n464 = Unbundle By Name(w1091) -> ("Real Mode"=w1090:bool)
        n465 = Format Into String(format string="%s", initial string="//" ("string"), w1103) -> (resulting string=w1101:string)  [unwired: 1 in, 1 out]
        n466 = Concatenate Strings(w1101, "/CFX315Writer" ("string")) -> (w1113:string)
        n467 = Create Network Stream Reader Endpoint(5:1000 ("timeout in ms (-1)"), 7:1 ("reader buffer size"), 8:w1107, 9:cluster{"Data":variant, "Timestamp":timestamp} {"Data"=variant, "Timestamp"=timestamp(0 s since 1904-01-01)} ("Dataset"), 10:w1113, 11:"GUIReader1" ("reader name")) -> (0:w1106:errorcluster, 3:w1100:refnum<k21>)  [unwired: 1 in]
        n468 = Concatenate Strings(w1101, "/CFX315Reader" ("writer name")) -> (w1108:string)
        n469 = Create Network Stream Writer Endpoint(5:1000 ("timeout in ms (-1)"), 7:1 ("writer buffer size"), 8:w1106, 9:variant, 10:w1108, 11:"GUIWriter1" ("writer name")) -> (0:w1096:errorcluster, 3:w1095:refnum<k21>)  [unwired: 1 in]
        n470 = case shown="True" w1090 {
          tunnel: w1096 -> [w1119 w1124]
          tunnel: w1095 -> [_ w1123]
          tunnel: [w1119 w1122] -> w1089
          tunnel: [TRUE ("Connected") w1121] -> w1088
          frame False {
          }
          frame True {
            n471 = property class="Network Stream Endpoint"(reference=w1123, error in=w1124) -> (error out=w1122:errorcluster, "Connected"=w1121:bool)  [unwired: 1 out]
          }
        }
        n472 = Bundle By Name(cluster=w1091, "reader endpoint"=w1100, "writer endpoint"=w1095, "Network Connection"=w1088) -> (w1093:T24)
        n473 = Unbundle By Name(w1093) -> ("Connected System"=w1092:string)
        n474 = Select(t="NS:Read\nUI:Module Enable" ("Command"), s=w1088, f="NS:Close Connection\nNS:Open Connection" ("Command")) -> (s? t:f=w1098:string)
        n475 = call "Messaging EnQ Multiline String.vi"("Command(s)"=w1098, "error in (no error)"=w1089) -> ("error out"=w1097:errorcluster)  [unwired: 9 in]
      }
      frame "NS:Close Connection" {
        w1125 = FALSE ("Network Connection")
        n476 = Unbundle By Name(w1128) -> ("reader endpoint"=w1130:refnum<k21>, "writer endpoint"=w1129:refnum<k21>)
        n477 = Destroy Stream Endpoint(8:w1132, 11:w1129) -> (0:w1131:errorcluster)
        n478 = Destroy Stream Endpoint(8:w1131, 11:w1130) -> (0:w1126:errorcluster)
        n479 = Bundle By Name(cluster=w1128, "Network Connection"=w1125, "System Ready"=w1125, "M2 Bootup"=w1125) -> (w1127:T24)
      }
      frame "NS:Read" {
        n480 = Unbundle By Name(w1134) -> ("Network Connection"=w1135:bool, "Dataset"=w1136:T29, "reader endpoint"=w1140:refnum<k21>)
        n481 = Unbundle By Name(w1134) -> ("Real Mode"=w1133:bool)
        n482 = shared-variable-read(w1140, w1146, 1000 ("timeout ms (-1)"), cluster{"Data":variant, "Timestamp":timestamp} {"Data"=variant, "Timestamp"=timestamp(0 s since 1904-01-01)} ("Dataset")) -> (w1145:errorcluster, w1144:bool, w1143:cluster{"Data":variant, "Timestamp":timestamp})  [unwired: 1 out]
        n483 = Or(x=w1144, y=w1145) -> (x .or. y?=w1148:bool)
        n484 = case shown="True" w1148 {
          tunnel: [w1166 w1177] -> w1149
          tunnel: w1134 -> [w1165 w1178]
          tunnel: [w1155 w1175] -> w1147
          tunnel: w1136 -> [w1161 _]
          tunnel: w1145 -> [w1159 w1180]
          tunnel: w1143 -> [w1160 _]
          tunnel: w1140 -> [_ w1179]
          tunnel: [w1154 FALSE ("Connected")] -> w1139
          tunnel: [w1153 _] -> w1138
          tunnel: [w1152 _] -> w1137
          tunnel: w1135 -> [w1150 _]
          tunnel: w1133 -> [_ w1173]
          frame False {
            n485 = Unbundle By Name(w1160) -> ("Timestamp"=→"Data Rx Timestamp":timestamp, "Data"=w1164:variant)
            n486 = Variant To Data(error in=w1159, type=w1161, Variant=w1164) -> (data=w1162:T29, error out=w1156:errorcluster)
            n487 = call "Messaging EnQ Single.vi"("Command"="UI:Update Network Down Data", "@Front?"=TRUE, "error in (no error)"=w1156) -> ("error out"=w1155:errorcluster)  [unwired: 8 in]
            n488 = call "Is Value Changed.vim"("value"=w1150) -> ("changed or first call?"=w1151:bool)
            n489 = case shown="False" w1151 {
              tunnel: [FALSE ("Connected") w1170] -> w1154
              tunnel: ["" ("Name") "Start Streaming" ("Name")] -> w1152
              tunnel: [FALSE ("Connected") w1170] -> w1153
              frame False {
              }
              frame True {
                w1170 = TRUE ("Connected")
              }
            }
            n490 = Bundle By Name(cluster=w1165, "Dataset"=w1162) -> (w1166:T24)
          }
          frame True {
            n491 = case shown="True" w1173 {
              tunnel: w1180 -> [_ w1186]
              tunnel: w1179 -> [_ w1185]
              tunnel: [errorcluster {"status"=FALSE, "code"=0, "source"=""} ("error out") w1184] -> w1176
              tunnel: [TRUE ("Connected") w1183] -> w1172
              frame False {
              }
              frame True {
                n492 = property class="Network Stream Endpoint"(reference=w1185, error in=w1186) -> (error out=w1184:errorcluster, "Connected"=w1183:bool)  [unwired: 1 out]
              }
            }
            n493 = case shown="False" w1172 {
              tunnel: w1176 -> [w1191 w1192]
              tunnel: [w1189 w1192] -> w1175
              frame False {
                n494 = call <vilib>:"Clear Errors.vi"("error in (no error)"=w1191) -> ("error out"=w1190:errorcluster)  [unwired: 5 in, 1 out]
                n495 = call "Messaging EnQ Multiline String.vi"("Command(s)"="NS:Close Connection\nUI:Reinitialize Front Panel\nNS:Open Connection" ("Command"), "@Front?"=TRUE, "error in (no error)"=w1190) -> ("error out"=w1189:errorcluster)  [unwired: 8 in]
              }
              frame True {
              }
            }
            n496 = Bundle By Name(cluster=w1178, "System Ready"=w1172, "Network Connection"=w1172) -> (w1177:T24)
          }
        }
      }
      frame "NS:Write" {
        n497 = Index Array(array=w1209) -> (element=w1201:string)  [unwired: 1 in]
        n498 = case shown="\"M1 Enable\"" w1201 {
          tunnel: w1199 -> [w1210 w1224 w1235 w1247 w1261 w1273 w1286 w1298 w1310 w1322 w1334 w1346 w1357 w1365 w1389]
          tunnel: [w1212 w1222 w1233 w1246 w1259 w1271 w1284 w1296 w1308 w1321 w1328 w1340 w1358 w1362 w1385] -> w1197
          tunnel: [w1210 w1223 w1234 w1238 w1258 w1272 w1285 w1297 w1309 w1320 w1333 w1341 w1356 w1361 w1384] -> w1196
          tunnel: w1198 -> [w1212 w1220 w1232 w1245 w1257 w1270 w1283 w1295 w1307 w1319 w1329 w1342 w1354 w1363 w1386]
          tunnel: ["No data to command" w1217 w1228 w1241 w1252 w1265 w1278 w1290 w1303 w1314 w1332 w1345 w1351 w1360 w1381] -> w1195
          tunnel: [_ w1216 w1227 w1240 w1251 w1266 w1279 w1291 w1301 w1315 w1331 w1344 w1349 w1359 w1378] -> w1194
          tunnel: w1200 -> [_ w1214 w1226 w1239 w1250 w1263 w1276 w1288 w1300 w1312 w1330 w1343 w1348 w1364 w1388]
          frame Default {
          }
          frame "Power On-Off" {
            w1213 = NS_New_Data."System Power" ("New Data")
            n499 = Variant To Data(error in=w1224, type=TRUE, Variant=w1214) -> (data=w1218:bool, error out=w1223:errorcluster)
            n500 = Bundle By Name(cluster=w1220, "Network Data Down.System Power On Off"=w1218, "Network Data Down.New Data"=w1213) -> (w1222:T24)
            n501 = call <vilib>:"Space Constant.vi"() -> ("String"=w1219:string)
            n502 = Format Into String(w1213) -> (resulting string=w1215:string)  [unwired: 3 in, 1 out]
            n503 = Format Into String(w1218) -> (resulting string=w1216:string)  [unwired: 3 in, 1 out]
            n504 = Concatenate Strings(w1215, w1219, w1216) -> (w1217:string)
          }
          frame "M1 Power Drive Control" {
            w1225 = NS_New_Data."M1 Power Drive" ("New Data")
            n505 = Variant To Data(error in=w1235, type=TRUE, Variant=w1226) -> (data=w1230:bool, error out=w1234:errorcluster)
            n506 = Format Into String(w1230) -> (resulting string=w1227:string)  [unwired: 3 in, 1 out]
            n507 = Bundle By Name(cluster=w1232, "Network Data Down.M1 Commands.Power Drive"=w1230, "Network Data Down.New Data"=w1225) -> (w1233:T24)
            n508 = call <vilib>:"Space Constant.vi"() -> ("String"=w1231:string)
            n509 = Format Into String(w1225) -> (resulting string=w1229:string)  [unwired: 3 in, 1 out]
            n510 = Concatenate Strings(w1229, w1231, w1227) -> (w1228:string)
          }
          frame "M2 Power Drive Control" {
            w1237 = NS_New_Data."M2 Power Drive" ("New Data")
            (unwired) FALSE ("data")
            n511 = Variant To Data(error in=w1247, type=TRUE, Variant=w1239) -> (data=w1243:bool, error out=w1238:errorcluster)
            n512 = Format Into String(w1243) -> (resulting string=w1240:string)  [unwired: 3 in, 1 out]
            n513 = Bundle By Name(cluster=w1245, "Network Data Down.M2 Commands.Power Drive"=w1243, "Network Data Down.New Data"=w1237) -> (w1246:T24)
            n514 = call <vilib>:"Space Constant.vi"() -> ("String"=w1244:string)
            n515 = Format Into String(w1237) -> (resulting string=w1242:string)  [unwired: 3 in, 1 out]
            n516 = Concatenate Strings(w1242, w1244, w1240) -> (w1241:string)
          }
          frame "M1 Set Temp" {
            w1249 = NS_New_Data."M1 Set Point" ("New Data")
            n517 = Variant To Data(error in=w1261, type=20.0 ("SET TEMP 1"), Variant=w1250) -> (data=w1255:dbl, error out=w1258:errorcluster)
            n518 = Number To Fractional String(number=w1255, precision (6)=i16 1) -> (F-format string=w1251:string)  [unwired: 2 in]
            n519 = Bundle By Name(cluster=w1257, "Network Data Down.M1 Commands.Set Temp"=w1255, "Network Data Down.New Data"=w1249) -> (w1259:T24)
            n520 = Format Into String(w1249) -> (resulting string=w1253:string)  [unwired: 3 in, 1 out]
            n521 = call <vilib>:"Space Constant.vi"() -> ("String"=w1254:string)
            n522 = Concatenate Strings(w1253, w1254, w1251) -> (w1252:string)
          }
          frame "M2 Set Temp" {
            w1262 = NS_New_Data."M2 Set Point" ("New Data")
            n523 = Variant To Data(error in=w1273, type=0.0 ("SET TEMP 1"), Variant=w1263) -> (data=w1267:dbl, error out=w1272:errorcluster)
            n524 = Number To Fractional String(number=w1267, precision (6)=i16 1) -> (F-format string=w1266:string)  [unwired: 2 in]
            n525 = Bundle By Name(cluster=w1270, "Network Data Down.M2 Commands.Set Temp"=w1267, "Network Data Down.New Data"=w1262) -> (w1271:T24)
            n526 = Format Into String(w1262) -> (resulting string=w1264:string)  [unwired: 3 in, 1 out]
            n527 = call <vilib>:"Space Constant.vi"() -> ("String"=w1269:string)
            n528 = Concatenate Strings(w1264, w1269, w1266) -> (w1265:string)
          }
          frame "M1 Feedback" {
            w1275 = NS_New_Data."M1 Feedback" ("New Data")
            n529 = Variant To Data(error in=w1286, type=u8 0 ("Network Data Down.M1 Commands.Feedback"), Variant=w1276) -> (data=w1281:u8, error out=w1285:errorcluster)
            n530 = Format Into String(w1281) -> (resulting string=w1279:string)  [unwired: 3 in, 1 out]
            n531 = Bundle By Name(cluster=w1283, "Network Data Down.M1 Commands.Feedback"=w1281, "Network Data Down.New Data"=w1275) -> (w1284:T24)
            n532 = Format Into String(w1275) -> (resulting string=w1277:string)  [unwired: 3 in, 1 out]
            n533 = call <vilib>:"Space Constant.vi"() -> ("String"=w1280:string)
            n534 = Concatenate Strings(w1277, w1280, w1279) -> (w1278:string)
          }
          frame "M2 Feedback" {
            w1287 = NS_New_Data."M2 Feedback" ("New Data")
            n535 = Variant To Data(error in=w1298, type=u8 0 ("Network Data Down.M2 Commands.Feedback"), Variant=w1288) -> (data=w1289:u8, error out=w1297:errorcluster)
            n536 = Bundle By Name(cluster=w1295, "Network Data Down.M2 Commands.Feedback"=w1289, "Network Data Down.New Data"=w1287) -> (w1296:T24)
            n537 = Format Into String(w1289) -> (resulting string=w1291:string)  [unwired: 3 in, 1 out]
            n538 = Format Into String(w1287) -> (resulting string=w1292:string)  [unwired: 3 in, 1 out]
            n539 = call <vilib>:"Space Constant.vi"() -> ("String"=w1293:string)
            n540 = Concatenate Strings(w1292, w1293, w1291) -> (w1290:string)
          }
          frame "M1 Package" {
            w1299 = NS_New_Data."M1 Package" ("New Data")
            n541 = Variant To Data(error in=w1310, type=u16 0 ("Network Data Down.M1 Commands.Package"), Variant=w1300) -> (data=w1304:u16, error out=w1309:errorcluster)
            n542 = Bundle By Name(cluster=w1307, "Network Data Down.M1 Commands.Package"=w1304, "Network Data Down.New Data"=w1299) -> (w1308:T24)
            n543 = Format Into String(w1304) -> (resulting string=w1301:string)  [unwired: 3 in, 1 out]
            n544 = Format Into String(w1299) -> (resulting string=w1302:string)  [unwired: 3 in, 1 out]
            n545 = call <vilib>:"Space Constant.vi"() -> ("String"=w1305:string)
            n546 = Concatenate Strings(w1302, w1305, w1301) -> (w1303:string)
          }
          frame "M2 Package" {
            w1311 = NS_New_Data."M2 Package" ("New Data")
            n547 = Variant To Data(error in=w1322, type=u16 0 ("Network Data Down.M2 Commands.Package"), Variant=w1312) -> (data=w1316:u16, error out=w1320:errorcluster)
            n548 = Bundle By Name(cluster=w1319, "Network Data Down.M2 Commands.Package"=w1316, "Network Data Down.New Data"=w1311) -> (w1321:T24)
            n549 = Format Into String(w1316) -> (resulting string=w1315:string)  [unwired: 3 in, 1 out]
            n550 = Format Into String(w1311) -> (resulting string=w1313:string)  [unwired: 3 in, 1 out]
            n551 = call <vilib>:"Space Constant.vi"() -> ("String"=w1317:string)
            n552 = Concatenate Strings(w1313, w1317, w1315) -> (w1314:string)
          }
          frame "M1 Enable" {
            w1324 = NS_New_Data."M1 Enable" ("New Data")
            n553 = Variant To Data(error in=w1334, type=TRUE, Variant=w1330) -> (data=w1323:bool, error out=w1333:errorcluster)
            n554 = Bundle By Name(cluster=w1329, "Network Data Down.M1 Commands.Enable"=w1323, "Network Data Down.New Data"=w1324) -> (w1328:T24)
            n555 = Format Into String(w1323) -> (resulting string=w1331:string)  [unwired: 3 in, 1 out]
            n556 = Format Into String(w1324) -> (resulting string=w1325:string)  [unwired: 3 in, 1 out]
            n557 = call <vilib>:"Space Constant.vi"() -> ("String"=w1326:string)
            n558 = Concatenate Strings(w1325, w1326, w1331) -> (w1332:string)
          }
          frame "M2 Enable" {
            w1335 = NS_New_Data."M2 Enable" ("New Data")
            n559 = Variant To Data(error in=w1346, type=TRUE, Variant=w1343) -> (data=w1337:bool, error out=w1341:errorcluster)
            n560 = Bundle By Name(cluster=w1342, "Network Data Down.M2 Commands.Enable"=w1337, "Network Data Down.New Data"=w1335) -> (w1340:T24)
            n561 = Format Into String(w1337) -> (resulting string=w1344:string)  [unwired: 3 in, 1 out]
            n562 = Format Into String(w1335) -> (resulting string=w1336:string)  [unwired: 3 in, 1 out]
            n563 = call <vilib>:"Space Constant.vi"() -> ("String"=w1338:string)
            n564 = Concatenate Strings(w1336, w1338, w1344) -> (w1345:string)
          }
          frame "Update Config" {
            w1347 = NS_New_Data."Config Data" ("New Data")
            w1349 = "Download"
            w1353 = T32 {"Packages"={"DUT Force lbf"={" 0"=0, " 1"=0, " 2"=0, "3"=0, "4"=0, "5"=0, " 6"=0, "7"=0, "8"=0, "9"=0}, "DUT Names"={"0"="", "1"="", "2"="", "3"="", "4"="", "5"="", "6"="", "7"="", "8"="", "9"=""}}, "Heater PID"={"P"=0.0, "I"=0.0, "D"=0.0}, "Piston Settings"={"Forces Slope"=0.0, "Forces Intercept"=0.0, "Transition Force"=0.0, "Up Force"=0.0, "Diameter (mm)"=0.0, "Delay (ms)"=0.0, "Pressure Ramp Delay (ms)"=0.0}, "Safe Temps"={"Minimum"=17, "Enabled"=TRUE, "Maximum"=95}, "System Settings"={"Number of Heads"=0, "60Hz Power"=TRUE, "FTC200"=TRUE, "AutoStartup"=FALSE, "Purge"=TRUE, "Sensors"=TRUE, "HandClamp"=TRUE, "ATE"=TRUE, "Benchtop"=TRUE, "Production"=TRUE, "Refrigerant"=0, "Handler"=TRUE, "Shuttle"=TRUE, "220V"=FALSE, "Cascade"=FALSE, "Suction Sensor"=0, "Discharge Sensor"=0}, "Stepper Settings "={"Microstepping"=0, "Velocity"=8}, "Set Point Range"={"Max"=0.0, "Min"=0.0}, "Pedestal Check DeltaT"=0.0, "Ramp Delta T"=0.0, "Ramp-SS Threshold"=0.0, "SS Tolerance"=0.0, "EEV PID"={"Ramp Up Target"=0.0, "Ramp Down Target"=0.0, "Steady State Target"=0.0, "Output"={"Max"=0.0, "Min"=0.0}, "EBB and Flow Temp TH"=0.0, "Cryomode EEV Max"=0.0, "Valve minimum opening "=0.0, "Ramp Up EEV Steps"=0.0, "Ramp Down EEV Steps"=0.0, "SS EEV Steps Reset"=0.0, "EBB and Flow Tol"=0.0, "Gains"={"P"=0.0, "I"=0.0, "D"=0.0}, "Dissabled Target"=0.0, "CryoMode Gains"={"P"=0.0, "I"=0.0, "D"=0.0}, "M1 SuperHeat Setpoint"=0.0, "M2 Gains"={"P"=0.0, "I"=0.0, "D"=0.0}, "Flow Curve"=0}, "Sleep Timeout"=0.0, "Bypass Values"={"Bypass Valve"=TRUE, "Flow Curve"=0, "Output"={"Max"=0, "Min"=0}, "Feedback"=0, "Cyth Bypass"=TRUE, "PID"={"P"=0.0, "I"=0.0, "D"=0.0}, "Pressure setpoint"=0, "Cryo Temp"=0, "Superheat Setpoint"=0, "Cryo Setpoint"=0}, "Default Temp"=0.0, "InTEC"={"Enabled"=FALSE, "IP"="192.168.1.100", "Port"=5000}, "M1 TSD"={"Gain"=0.0, "Offset"=0.0, "V Offset "=0.0}, "M2 TSD"={"Gain"=0.0, "Offset"=0.0, "V Offset "=0.0}, "M1 T-Case Calibration"={"Gain"=0.0, "Offset"=0.0}, "M2 T-Case Calibration"={"Gain"=0.0, "Offset"=0.0}, "Heater PID TSD"={"P"=0.0, "I"=0.0, "D"=0.0}, "M2 Heater PID"={"P"=0.0, "I"=0.0, "D"=0.0}}  # Config Data
            n565 = Variant To Data(error in=w1357, type=w1353, Variant=w1348) -> (data=w1355:T32, error out=w1356:errorcluster)
            n566 = Bundle By Name(cluster=w1354, "Network Data Down.Config Data"=w1355, "Network Data Down.New Data"=w1347) -> (w1358:T24)
            n567 = Format Into String(w1347) -> (resulting string=w1350:string)  [unwired: 3 in, 1 out]
            n568 = call <vilib>:"Space Constant.vi"() -> ("String"=w1352:string)
            n569 = Concatenate Strings(w1350, w1352, w1349) -> (w1351:string)
          }
          frame "Reboot RT" {
            n570 = disable-structure shown="Disabled" {
              disable-tunnel: w1365 -> [w1376 _]
              disable-tunnel: w1364 -> [w1375 _]
              disable-tunnel: w1363 -> [w1374 w1377]
              disable-tunnel: [w1373 w1377] -> w1362
              disable-tunnel: [w1372 _] -> w1361
              disable-tunnel: [w1371 _] -> w1360
              disable-tunnel: [w1370 _] -> w1359
              frame Disabled {
                w1367 = TRUE  # Reboot RT
                # "Change Reboot process"
                n571 = Variant To Data(error in=w1376, type=w1367, Variant=w1375) -> (data=w1366:bool, error out=w1372:errorcluster)
                n572 = Format Into String(w1366) -> (resulting string=w1370:string)  [unwired: 3 in, 1 out]
                n573 = Format Into String(w1366) -> (resulting string=w1368:string)  [unwired: 3 in, 1 out]
                n574 = call <vilib>:"Space Constant.vi"() -> ("String"=w1369:string)
                n575 = Concatenate Strings(w1368, w1369, w1370) -> (w1371:string)
                n576 = Bundle By Name(cluster=w1374, "Reboot"=w1366) -> (w1373:T24)
              }
              frame Enabled {
              }
            }
          }
          frame "Stop RT" {
            w1380 = NS_New_Data."Stop RT" ("Network Data Down.New Data")
            n577 = Variant To Data(error in=w1389, type=TRUE ("STop RT"), Variant=w1388) -> (data=w1379:bool, error out=w1384:errorcluster)
            n578 = Format Into String(w1379) -> (resulting string=w1378:string)  [unwired: 3 in, 1 out]
            n579 = Format Into String(w1380) -> (resulting string=w1382:string)  [unwired: 3 in, 1 out]
            n580 = Bundle By Name(cluster=w1386, "Network Data Down.Stop RT"=w1379, "Network Data Down.New Data"=w1380) -> (w1385:T24)
            n581 = call <vilib>:"Space Constant.vi"() -> ("String"=w1383:string)
            n582 = Concatenate Strings(w1382, w1383, w1378) -> (w1381:string)
          }
        }
        n583 = Unbundle By Name(w1197) -> ("writer endpoint"=w1207:refnum<k21>, "Network Data Down"=w1204:T25)
        n584 = To Variant(anything=w1204) -> (Variant=w1203:variant)
        n585 = shared-variable-write(w1207, w1196, w1203) -> (w1206:refnum<k21>, w1208:errorcluster)  [unwired: 1 in, 1 out]
        n586 = Flush Stream(8:w1208, 9:0 ("timeout in ms (-1)"), 11:w1206) -> (0:w1205:errorcluster)  [unwired: 1 in, 2 out]
      }
      frame "----Network Shared Variables-----" {
      }
      frame "NSV:Write" {
        n587 = Unbundle By Name(w1402) -> ("IP Address"=w1401:string)
        n588 = Index Array(array=w1399) -> (element=w1394:string)  [unwired: 1 in]
        n589 = Concatenate Strings("ni.var.psp://", w1401, "/Network Shared Variables/") -> (w1400:string)
        n590 = case shown="\"M2 Heater Output\"" w1394 {
          selector: w1394 -> [_ w1411 w1423 w1435 w1447 w1459 _ w1480 _ _]
          tunnel: w1400 -> [_ w1412 w1424 w1436 w1448 w1460 w1464 w1481 w1490 w1500]
          tunnel: w1398 -> [w1405 w1415 w1427 w1439 w1451 w1463 w1476 w1486 w1496 w1506]
          tunnel: w1397 -> [_ w1414 w1426 w1438 w1450 w1462 w1475 w1485 w1495 w1505]
          tunnel: [w1405 w1407 w1420 w1432 w1444 w1456 w1470 w1484 w1493 w1503] -> w1396
          tunnel: [_ _ w1418 w1430 w1441 w1453 _ _ _ _] -> w1393
          tunnel: [_ _ _ _ _ _ _ _ w1487 w1497] -> w1392
          frame Default {
          }
          frame "Cascade Compressor controls" {
            n591 = Variant To Data(error in=w1415, type=T22 {"High Stage manual speed control"=FALSE, "Manual High stage frequency"=0.0, "Low Stage manual speed control"=FALSE, "Manual Low Stage frequency"=0.0} ("Cascade Compressor controls"), Variant=w1414) -> (data=w1409:T22, error out=w1410:errorcluster)
            n592 = Format Into String(format string="%s", initial string=w1412, w1411) -> (resulting string=w1408:string)  [unwired: 1 in, 1 out]
            n593 = shared-variable-write(w1408, w1410, w1409) -> (w1407:errorcluster)  [unwired: 1 out]
          }
          frame "M2 EEV Manual" {
            n594 = Variant To Data(error in=w1427, type=i16 0 ("M2 EEV Manual control"), Variant=w1426) -> (data=w1417:i16, error out=w1422:errorcluster)
            n595 = Format Into String(format string="%s", initial string=w1424, w1423) -> (resulting string=w1421:string)  [unwired: 1 in, 1 out]
            n596 = shared-variable-write(w1421, w1422, w1417) -> (w1420:errorcluster)  [unwired: 1 out]
            n597 = Number To Engineering String(2:i16 1 ("precision (6)"), 4:w1417) -> (0:w1418:string)  [unwired: 2 in]
          }
          frame "M1 EEV Manual" {
            n598 = Variant To Data(error in=w1439, type=i16 0 ("M2 EEV Manual control"), Variant=w1438) -> (data=w1429:i16, error out=w1434:errorcluster)
            n599 = Format Into String(format string="%s", initial string=w1436, w1435) -> (resulting string=w1433:string)  [unwired: 1 in, 1 out]
            n600 = shared-variable-write(w1433, w1434, w1429) -> (w1432:errorcluster)  [unwired: 1 out]
            n601 = Number To Engineering String(2:i16 1 ("precision (6)"), 4:w1429) -> (0:w1430:string)  [unwired: 2 in]
          }
          frame "M1 Heater output" {
            n602 = Variant To Data(error in=w1451, type=0.0 ("M1 Heater PWM"), Variant=w1450) -> (data=w1442:dbl, error out=w1446:errorcluster)
            n603 = Format Into String(format string="%s", initial string=w1448, w1447) -> (resulting string=w1445:string)  [unwired: 1 in, 1 out]
            n604 = shared-variable-write(w1445, w1446, w1442) -> (w1444:errorcluster)  [unwired: 1 out]
            n605 = Number To Engineering String(2:i16 1 ("precision (6)"), 4:w1442) -> (0:w1441:string)  [unwired: 2 in]
          }
          frame "M2 Heater Output" {
            n606 = Variant To Data(error in=w1463, type=0.0 ("M1 Heater PWM"), Variant=w1462) -> (data=w1454:dbl, error out=w1458:errorcluster)
            n607 = Format Into String(format string="%s", initial string=w1460, w1459) -> (resulting string=w1457:string)  [unwired: 1 in, 1 out]
            n608 = shared-variable-write(w1457, w1458, w1454) -> (w1456:errorcluster)  [unwired: 1 out]
            n609 = Number To Engineering String(2:i16 1 ("precision (6)"), 4:w1454) -> (0:w1453:string)  [unwired: 2 in]
          }
          frame "Thermal Load" {
            n610 = Variant To Data(error in=w1476, type=0.0 ("Numeric"), Variant=w1475) -> (data=w1471:dbl, error out=w1469:errorcluster)
            n611 = Format Into String(format string="%s", initial string=w1464, "Network Inputs" ("input 1")) -> (resulting string=w1465:string)  [unwired: 1 in, 1 out]
            n612 = Replace Array Subset(array=dbl[] [0.0, 0.0], new element=w1471, index=0) -> (w1468:dbl[])
            n613 = shared-variable-write(w1465, w1469, w1468) -> (w1470:errorcluster)  [unwired: 1 out]
          }
          frame "Manual Bypass Mode" {
            n614 = Variant To Data(error in=w1486, type=bool[] [] ("Manual Bypass Mode"), Variant=w1485) -> (data=w1478:bool[], error out=w1483:errorcluster)
            n615 = Format Into String(format string="%s", initial string=w1481, w1480) -> (resulting string=w1479:string)  [unwired: 1 in, 1 out]
            n616 = shared-variable-write(w1479, w1483, w1478) -> (w1484:errorcluster)  [unwired: 1 out]
          }
          frame "M1 TSD Feedback" {
            n617 = Variant To Data(error in=w1496, type=FALSE ("TSD Feedback"), Variant=w1495) -> (data=w1487:bool, error out=w1492:errorcluster)
            n618 = Format Into String(format string="%s", initial string=w1490, "TSD Feedback" ("input 1")) -> (resulting string=w1489:string)  [unwired: 1 in, 1 out]
            n619 = shared-variable-write(w1489, w1492, w1487) -> (w1493:errorcluster)  [unwired: 1 out]
          }
          frame "M2 TSD Feedback" {
            n620 = Variant To Data(error in=w1506, type=FALSE ("TSD Feedback"), Variant=w1505) -> (data=w1497:bool, error out=w1502:errorcluster)
            n621 = Format Into String(format string="%s", initial string=w1500, "M2 TSD Feedback" ("input 1")) -> (resulting string=w1499:string)  [unwired: 1 in, 1 out]
            n622 = shared-variable-write(w1499, w1502, w1497) -> (w1503:errorcluster)  [unwired: 1 out]
          }
        }
      }
      frame "NSV:Read" {
        n623 = Unbundle By Name(w1511) -> ("IP Address"=w1512:string)
        n624 = Concatenate Strings("ni.var.psp://", w1512, "/Network Shared Variables/") -> (w1510:string)
        n625 = for {
          tunnel: w1508 -> [w1517]
          tunnel: [w1518] -> w1507
          tunnel: w1509 -> [w1516] mode=indexing
          tunnel: w1510 -> [w1515]
          n626 = Concatenate Strings(w1515, w1516) -> (w1519:string)
          n627 = case shown="\"Output Cluster\"" w1516 {
            tunnel: w1517 -> [w1524 w1535 w1551 w1568 w1574 w1580 w1585 w1590 w1595 w1600 w1607 w1612 w1625 w1628 w1643]
            tunnel: [w1522 w1525 w1536 w1568 w1573 w1579 w1583 w1588 w1594 w1596 w1606 w1611 w1621 w1626 w1642] -> w1518
            tunnel: w1519 -> [w1523 w1534 w1550 _ w1572 w1578 w1584 w1589 w1592 w1599 w1605 w1610 w1624 w1630 w1645]
            frame "BootupTime" {
              n628 = shared-variable-read(w1523, w1524, timestamp(0 s since 1904-01-01)) -> (w1522:errorcluster, →"Boot Up Time":timestamp)  [unwired: 2 out]
            }
            frame "Output Cluster" {
              # "Read the RT Information to debug GUI"
              n629 = shared-variable-read(w1534, w1535, T5 {"Condensing Pressure"=0.0, "Suction Pressure"=0.0, "Bypass steps"=0, "Operating Time"=0.0, "SubCooling"=0.0, "Superheat"=0.0, "M1 Superheat"=0.0, "M2 Superheat"=0.0, "Autotune output"=0.0, "M1 Testing Elapsed Time"=0.0, "M2 Testing Elapsed Time"=0.0, "M1 Valve Control Mode"=0, "System Amps"=0.0, "Compressor Run Time"=0.0, "SD card free Space"=0.0, "Free Memory"=0.0, "M1 Pressure Feedback"=0.0, "M2 Pressure Feedback"=0.0, "Compression Ratio"=0.0, "Serial Number"=0.0, "M1 AC Load V"=0.0, "M1 AC Load W"=0.0, "M1 DC Load W"=0.0, "M1 RH"=0.0, "RH Threshold"=0.0} ("output cluster")) -> (w1525:errorcluster, w1532:T5)  [unwired: 2 out]
              "data out" <- w1532
              n630 = Unbundle By Name(w1532) -> ("RH Threshold"=w1527:dbl, "M1 RH"=w1528:dbl, "M1 Superheat"=→"M1 Superheat":dbl, "M1 Testing Elapsed Time"=→"M1 Testing Elapsed Time":dbl, "M1 AC Load V"=→"M1 AC Load V":dbl)
              n631 = Bundle("RH Threshold"=w1527, "M1 RH"=w1528) -> (→"M1 Humidity":cluster{"RH Threshold":dbl, "M1 RH":dbl})  [unwired: 1 in]
            }
            frame "TSD" {
              n632 = shared-variable-read(w1550, w1551, T3 {"TSD Millivolts"=0.0, "X factor"=0.0, "Offset"=0.0, "TSD Temp"=0.0, "TSD Feedback"=FALSE, "TSD Max"=0.0, "TSD Min"=0.0} ("TSD Data")) -> (w1537:errorcluster, w1546:T3)  [unwired: 2 out]
              n633 = Unbundle By Name(w1546) -> ("TSD Millivolts"=w1548:dbl, "X factor"=w1542:dbl, "Offset"=w1541:dbl)
              n634 = in-place {
                in-place-border: "Change TSD" -> [w1558]
                in-place-border: w1537 -> [w1553]
                in-place-border: [w1552] -> w1536
                n635 = in-place-match #1(w1542) -> (w1557:dbl)
                n636 = in-place-match #2(w1541) -> (w1555:dbl)
                n637 = case shown="False" w1558 {
                  tunnel: w1557 -> [w1561 w1567]
                  tunnel: [w1561 w1565] -> w1556
                  tunnel: w1555 -> [w1560 w1566]
                  tunnel: [w1560 w1564] -> w1554
                  tunnel: w1553 -> [w1559 w1563]
                  tunnel: [w1559 w1562] -> w1552
                  frame False {
                  }
                  frame True {
                    n638 = call "New TSD Values.vi"("Error In"=w1563, "Offset"=w1566, "X factor"=w1567) -> ("Error Out"=w1562:errorcluster, "Offset out"=w1564:dbl, "X factor out"=w1565:dbl)  [unwired: 6 in]
                  }
                }
                n639 = in-place-match #1(w1556) -> (w1540:dbl)
                n640 = in-place-match #2(w1554) -> (w1539:dbl)
              }
              n641 = Equal To 0?(x=w1548) -> (x = 0?=w1547:bool)
              n642 = Select(t=nan, s=w1547, f=w1548) -> (s? t:f=w1545:dbl)
              n643 = Bundle By Name(cluster=w1546, "TSD Millivolts"=w1545, "X factor"=w1540, "Offset"=w1539) -> (→"TSD Data":T3)
            }
            frame "DC PS Load Watts" {
              # "We dont use DC power Supply Anymore, now the TTV uses AC programmable power supply.  It tells the cobra exaclty how many watts the TTV is producing"
              # "This is for testing and datalogging purpose"
            }
            frame "Event Log" {
              n644 = shared-variable-read(w1572, w1574, T19 [] ("Event Log")) -> (w1573:errorcluster, w1570:T19)  [unwired: 2 out]
              n645 = call "Is Value Changed.vim"("value"=w1570) -> ("changed or first call?"=w1569:bool)
              n646 = case shown="True" w1569 {
                tunnel: w1570 -> [_ w1575]
                frame False {
                }
                frame True {
                  "Event log" <- w1575
                }
              }
            }
            frame "AI", Default {
              # "NVIDIA Testing"
              # "Analog Inputs"
              n647 = shared-variable-read(w1578, w1580, dbl[] [] ("AI (V) 2")) -> (w1579:errorcluster, →"AI (V)":dbl[])  [unwired: 2 out]
            }
            frame "Errors" {
              n648 = shared-variable-read(w1584, w1585, string[] [] ("Errors 2")) -> (w1583:errorcluster, →"Errors" →"Error":string[])  [unwired: 2 out]
            }
            frame "TCP Command" {
              # "The list of ports with connection status"
              n649 = shared-variable-read(w1589, w1590, string[] [] ("Errors 2")) -> (w1588:errorcluster, →"TCP commands":string[])  [unwired: 2 out]
            }
            frame "compressor manual frequency control" {
              w1593 = T22 {"High Stage manual speed control"=FALSE, "Manual High stage frequency"=0.0, "Low Stage manual speed control"=FALSE, "Manual Low Stage frequency"=0.0}  # Cascade Compressor controls
              # "king cobra compressor RPM"
              n650 = shared-variable-read(w1592, w1595, w1593) -> (w1594:errorcluster, w1591:T22)  [unwired: 2 out]
              n651 = local write "Cascade Compressor controls"(w1591) -> ()
            }
            frame "Stack Light State" {
              # "Monitoring RT Status"
              n652 = shared-variable-read(w1599, w1600, T2."Sleeping Fault" ("Stack light states")) -> (w1596:errorcluster, →"Stack light states":T2)  [unwired: 2 out]
            }
            frame "M1 Values" {
              # "Array that includes EEV PID Output"
              n653 = shared-variable-read(w1605, w1607, dbl[] [0.0, 0.0]) -> (w1606:errorcluster, w1603:dbl[])  [unwired: 2 out]
              n654 = Index Array(array=w1603) -> (element #1=→"M1 Buffer":dbl, element #2=→"M1 Valve Output":dbl)  [unwired: 2 in]
            }
            frame "M2 Values" {
              n655 = disable-structure shown="Enabled" {
                disable-tunnel: [w1619 _] -> w1614
                disable-tunnel: dbl[] [0.0, 0.0] -> [w1618 _]
                disable-tunnel: w1612 -> [w1617 w1620]
                disable-tunnel: [w1616 w1620] -> w1611
                disable-tunnel: w1610 -> [w1615 _]
                frame Enabled {
                  n656 = shared-variable-read(w1615, w1617, w1618) -> (w1616:errorcluster, w1619:dbl[])  [unwired: 2 out]
                }
                frame Disabled {
                }
              }
              n657 = Index Array(array=w1614) -> (element #1=→"M2 Buffer":dbl, element #2=→"M2 Valve Output":dbl)  [unwired: 2 in]
            }
            frame "TCP Connections" {
              n658 = shared-variable-read(w1624, w1625, T21 [{"port "=1300, "remote address"="", "Connection timeout ms"=100, "Waiting for connection"=TRUE, "Waiting for Command"=TRUE, "timeout ms"=5000}] ("TCP Connections")) -> (w1621:errorcluster, →"TCP Connections":T21)  [unwired: 2 out]
            }
            frame "TSD Feedback" {
              n659 = shared-variable-read(w1630, w1628, FALSE ("data type")) -> (w1627:errorcluster, w1634:bool)  [unwired: 2 out]
              n660 = disable-structure shown="Disabled" {
                disable-tunnel: w1627 -> [w1638 _]
                disable-tunnel: [w1637 _] -> w1626
                frame Disabled {
                  n661 = flat-sequence {
                    tunnel: w1638 -> [w1640]
                    tunnel: [w1640] -> w1637
                    tunnel: u32 5000 ("milliseconds to wait") -> [w1639]
                    frame #0 {
                      n662 = Wait (ms)(milliseconds to wait=w1639) -> ()  [unwired: 1 out]
                    }
                  }
                }
                frame Enabled {
                }
              }
              n663 = call "Is Value Changed.vim"("value"=w1634) -> ("changed or first call?"=w1633:bool)
              n664 = Equal?(x=w1634, y=FALSE) -> (x = y?=w1635:bool)
              n665 = And(x=w1635, y=w1633) -> (x .and. y?=w1629:bool)
              n666 = case shown="False" w1629 {
                tunnel: w1634 -> [w1641 _]
                frame False {
                  n667 = property on="M1 TSD Feedback" class="Bool (strict)"("Value"=w1641) -> ()  [unwired: 2 in, 2 out]
                }
                frame True {
                }
              }
            }
            frame "M2 TSD Feedback" {
              n668 = shared-variable-read(w1645, w1643, FALSE ("data type")) -> (w1642:errorcluster, w1649:bool)  [unwired: 2 out]
              n669 = call "Is Value Changed.vim"("value"=w1649) -> ("changed or first call?"=w1648:bool)
              n670 = Equal?(x=w1649, y=FALSE) -> (x = y?=w1650:bool)
              n671 = And(x=w1650, y=w1648) -> (x .and. y?=w1644:bool)
              n672 = case shown="False" w1644 {
                tunnel: w1649 -> [w1651 _]
                frame False {
                  n673 = property on="M2 TSD Feedback" class="Bool (strict)"("Value"=w1651) -> ()  [unwired: 2 in, 2 out]
                }
                frame True {
                }
              }
            }
          }
        }
      }
      frame "-----------TCP-------------" {
      }
      frame "TCP:Open Connection" {
        w1665 = u16 3000  # port
        n674 = Unbundle By Name(w1661) -> ("IP Address"=w1667:string)
        n675 = TCP Open Connection(address=w1667, remote port or service name=w1665, error in (no error)=w1666) -> (connection ID=w1669:refnum<k5>, error out=w1668:errorcluster)  [unwired: 2 out]
        n676 = call-poly <vilib>:"Read Meta Data.vi"("error in"=w1668, "connection ID"=w1669) -> ("error out"=w1658:errorcluster, "connection info out"=w1657:T27)  [unwired: 1 in, 7 out]
        n677 = Unbundle By Name(w1657) -> ("connection ID"=w1656:refnum<k5>)
        n678 = Not A Number/Path/Refnum?(number/path/refnum=w1656) -> (NaN/Path/Refnum?=w1655:bool)
        n679 = Not(x=w1655) -> (.not. x?=w1654:bool)
        n680 = Bundle By Name(cluster=w1661, "TCP connection info"=w1657, "TCP Connection"=w1654) -> (w1660:T24)
        n681 = Number To Decimal String(number=w1665) -> (decimal integer string=w1659:string)  [unwired: 1 in]
      }
      frame "TCP:Read Dataset" {
        n682 = Unbundle By Name(w1672) -> ("Dataset"=w1673:T29, "TCP connection info"=w1674:T27)
        n683 = call-poly <vilib>:"Read Message.vi"("options"=T41 {"ignore timeout error"=TRUE, "timeout ms (1000)"=1000} ("Options"), "error in"=w1680, "connection info in"=w1674) -> ("error out"=w1678:errorcluster, "name"=w1676:T28, "data string"=w1677:string, "timed out?"=w1679:bool)  [unwired: 2 in, 3 out]
        n684 = case shown="False" w1679 {
          tunnel: w1677 -> [w1686 _]
          tunnel: w1676 -> [w1687 _]
          tunnel: w1678 -> [w1685 w1761]
          tunnel: [w1684 w1761] -> w1675
          tunnel: w1673 -> [w1683 _]
          tunnel: w1672 -> [w1682 w1760]
          tunnel: [w1681 w1760] -> w1671
          frame False {
            n685 = case shown="\"M2 History Data\"" w1687 {
              tunnel: w1686 -> [_ w1695 w1709 w1721 w1727 w1739 w1751]
              tunnel: w1685 -> [w1689 w1697 w1711 w1723 w1731 w1743 w1755]
              tunnel: [w1689 w1696 w1710 w1722 w1730 w1742 w1754] -> w1684
              tunnel: w1683 -> [_ _ _ w1719 w1726 w1738 w1750]
              tunnel: w1682 -> [w1688 w1692 w1706 w1718 w1729 w1741 w1753]
              tunnel: [w1688 w1691 w1705 w1718 w1728 w1740 w1752] -> w1681
              frame Default {
              }
              frame "M1 History Data " {
                n686 = Unflatten From JSON(JSON string=w1695, type and defaults=cluster{"Y":dbl[], "dt":dbl, "t0":dbl}[] [], error in (no error)=w1697) -> (value=w1693:cluster{"Y":dbl[], "dt":dbl, "t0":dbl}[], error out=w1696:errorcluster)  [unwired: 4 in]
                n687 = for {
                  tunnel: w1693 -> [w1700] mode=indexing
                  tunnel: [w1699] -> w1690 mode=indexing
                  tunnel: [w1698] -> _ mode=indexing
                  n688 = Unbundle By Name(w1700) -> ("t0"=w1702:dbl, "dt"=w1703:dbl, "Y"=w1699:dbl[])
                  n689 = To Time Stamp(1:w1702) -> (0:w1701:timestamp)
                  n690 = Bundle By Name("t0"=w1701, "dt"=w1703, "Y"=w1699) -> (w1698:waveform(dbl))  [unwired: 1 in]
                }
                n691 = Bundle By Name(cluster=w1692, "M1 History Temps"=w1690) -> (w1691:T24)
              }
              frame "M2 History Data" {
                n692 = Unflatten From JSON(JSON string=w1709, type and defaults=cluster{"Y":dbl[], "dt":dbl, "t0":dbl}[] [], error in (no error)=w1711) -> (value=w1707:cluster{"Y":dbl[], "dt":dbl, "t0":dbl}[], error out=w1710:errorcluster)  [unwired: 4 in]
                n693 = for {
                  tunnel: w1707 -> [w1714] mode=indexing
                  tunnel: [w1713] -> _ mode=indexing
                  tunnel: [w1712] -> w1704 mode=indexing
                  n694 = Unbundle By Name(w1714) -> ("t0"=w1716:dbl, "dt"=w1717:dbl, "Y"=w1712:dbl[])
                  n695 = To Time Stamp(1:w1716) -> (0:w1715:timestamp)
                  n696 = Bundle By Name("t0"=w1715, "dt"=w1717, "Y"=w1712) -> (w1713:waveform(dbl))  [unwired: 1 in]
                }
                n697 = Bundle By Name(cluster=w1706, "M2 History Temps"=w1704) -> (w1705:T24)
              }
              frame "System Module" {
                w1720 = T45 {"Power On Off"=FALSE, "Discharge Temp"=0.0, "Liquid Temp"=0.0, "Suction Temp"=0.0, "Ambient Temp"=0.0, "Sleep"=FALSE, "System Status"=0, "M1 Actuated"=FALSE, "M2 Actuated"=FALSE, "Sleep Timer"=0.0, "M1 Bin"={"Bin String"="", "Bin Color"=1}, "M2 Bin"={"Bin String"="", "Bin Color"=1}, "Discharge Pressure"=0.0, "Suction Pressure"=0.0, "Compression Ratio"=0.0, "Compressor Amps"=0.0, "Compressor Hours"=0.0, "Bypass Steps"=0, "SubCooling"=0.0, "SuperHeat"=0.0, "Serial Number"="", "EMO detected"=FALSE, "EMO Tripped"=FALSE, "Thermal cutoff"=FALSE, "Thermal cutoff 2"=FALSE, "High Pressure switch"=FALSE, "Running Time"="", "SOM Status"={"Boot Up Time"="", "Software Version"="", "CPU Usage"=0.0, "Memory Available"=0.0, "SD card free space"=0.0, "SOM Storage"=0.0}, "Cascade Extra"={"Discharge Temp High Side"=0.0, "Suction Temp High Side"=0.0, "Liquid Temp High side"=0.0, "Discharge Pressure 2"=0.0, "Suction Pressure 2"=0.0, "Low Side RPM"=0.0, "High Side RPM"=0.0}}  # System Status
                # "Timestamp can't unflatten from JSON"
                n698 = Unbundle By Name(w1719) -> ()  [unwired: 1 out]
                n699 = Unflatten From JSON(JSON string=w1721, type and defaults=w1720, error in (no error)=w1723) -> (error out=w1722:errorcluster)  [unwired: 4 in, 1 out]
              }
              frame "M1 Status" {
                n700 = Unbundle By Name(w1726) -> ("M1 Status"=w1725:T31)
                n701 = Unflatten From JSON(JSON string=w1727, type and defaults=w1725, error in (no error)=w1731) -> (value=w1724:T31, error out=w1730:errorcluster)  [unwired: 4 in]
                n702 = disable-structure shown="Disabled" {
                  disable-tunnel: w1729 -> [w1734 w1735]
                  disable-tunnel: [w1733 w1735] -> w1728
                  disable-tunnel: w1724 -> [w1732 _]
                  frame Disabled {
                    n703 = Bundle By Name(cluster=w1734, "Dataset.M1 Status"=w1732) -> (w1733:T24)
                  }
                  frame Enabled {
                  }
                }
              }
              frame "M2 Status" {
                n704 = Unbundle By Name(w1738) -> ("M2 Status"=w1737:T31)
                n705 = Unflatten From JSON(JSON string=w1739, type and defaults=w1737, error in (no error)=w1743) -> (value=w1736:T31, error out=w1742:errorcluster)  [unwired: 4 in]
                n706 = disable-structure shown="Enabled" {
                  disable-tunnel: w1741 -> [w1746 w1747]
                  disable-tunnel: [w1745 w1747] -> w1740
                  disable-tunnel: w1736 -> [w1744 _]
                  frame Disabled {
                    n707 = Bundle By Name(cluster=w1746, "Dataset.M2 Status"=w1744) -> (w1745:T24)
                  }
                  frame Enabled {
                  }
                }
              }
              frame "Config Data" {
                n708 = Unbundle By Name(w1750) -> ("Config Data"=w1749:T32)
                n709 = Unflatten From JSON(JSON string=w1751, type and defaults=w1749, error in (no error)=w1755) -> (value=w1748:T32, error out=w1754:errorcluster)  [unwired: 4 in]
                n710 = disable-structure shown="Enabled" {
                  disable-tunnel: w1753 -> [w1758 w1759]
                  disable-tunnel: [w1757 w1759] -> w1752
                  disable-tunnel: w1748 -> [w1756 _]
                  frame Disabled {
                    n711 = Bundle By Name(cluster=w1758, "Dataset.Config Data"=w1756) -> (w1757:T24)
                  }
                  frame Enabled {
                  }
                }
              }
            }
          }
          frame True {
          }
        }
      }
      frame "TCP:Write" {
        n712 = Index Array(array=w1770) -> (element=w1766:string)  [unwired: 1 in]
        n713 = case shown="\"M2 Enable\"" w1766 {
          tunnel: w1769 -> [w1774 w1781 w1787 w1794 w1804 w1812 w1821 w1829 w1837 w1845 w1852 w1859 w1866 w1873 w1880]
          tunnel: [w1774 w1777 w1784 w1790 w1800 w1806 w1816 w1823 w1832 w1840 w1851 w1857 w1861 w1871 w1876] -> w1763
          tunnel: w1768 -> [_ w1779 w1786 w1793 w1802 w1811 w1819 w1827 w1835 w1843 w1850 w1858 w1864 w1872 w1879]
          tunnel: [_ w1776 w1783 w1789 w1799 w1807 w1815 w1824 w1831 w1839 w1849 w1856 w1860 w1870 w1875] -> w1767
          tunnel: [_ w1775 w1782 _ _ _ _ _ _ _ w1848 w1855 _ w1869 w1874] -> w1765
          tunnel: [_ _ _ _ w1796 w1805 w1814 w1822 w1830 w1838 _ _ _ _ _] -> w1762
          frame Default {
            (unwired) "No data to command"
          }
          frame "Power On-Off" {
            n714 = Variant To Data(error in=w1781, type=TRUE, Variant=w1779) -> (data=w1775:bool, error out=w1778:errorcluster)
            n715 = call <vilib>:"Flatten To JSON String.vi"("error in (no error)"=w1778, "Variant"=w1775) -> ("error out"=w1777:errorcluster, "JSON String"=w1776:string)  [unwired: 8 in]
          }
          frame "M1 Power Drive Control" {
            n716 = Variant To Data(error in=w1787, type=TRUE, Variant=w1786) -> (data=w1782:bool, error out=w1785:errorcluster)
            n717 = call <vilib>:"Flatten To JSON String.vi"("error in (no error)"=w1785, "Variant"=w1782) -> ("error out"=w1784:errorcluster, "JSON String"=w1783:string)  [unwired: 8 in]
          }
          frame "M2 Power Drive Control" {
            n718 = Variant To Data(error in=w1794, type=TRUE, Variant=w1793) -> (data=w1791:bool, error out=w1792:errorcluster)
            n719 = call <vilib>:"Flatten To JSON String.vi"("error in (no error)"=w1792, "Variant"=w1791) -> ("error out"=w1790:errorcluster, "JSON String"=w1789:string)  [unwired: 8 in]
          }
          frame "M1 Set Temp" {
            n720 = Variant To Data(error in=w1804, type=20.0 ("SET TEMP 1"), Variant=w1802) -> (data=w1797:dbl, error out=w1801:errorcluster)
            n721 = call <vilib>:"Flatten To JSON String.vi"("error in (no error)"=w1801, "Variant"=w1797) -> ("error out"=w1800:errorcluster, "JSON String"=w1799:string)  [unwired: 8 in]
            n722 = Number To Engineering String(2:i16 1 ("precision (6)"), 4:w1797) -> (0:w1796:string)  [unwired: 2 in]
          }
          frame "M2 Set Temp" {
            n723 = Variant To Data(error in=w1812, type=0.0 ("SET TEMP 1"), Variant=w1811) -> (data=w1809:dbl, error out=w1808:errorcluster)
            n724 = call <vilib>:"Flatten To JSON String.vi"("error in (no error)"=w1808, "Variant"=w1809) -> ("error out"=w1806:errorcluster, "JSON String"=w1807:string)  [unwired: 8 in]
            n725 = Number To Engineering String(2:i16 1 ("precision (6)"), 4:w1809) -> (0:w1805:string)  [unwired: 2 in]
          }
          frame "M1 Feedback" {
            n726 = Variant To Data(error in=w1821, type=u8 0 ("Network Data Down.M1 Commands.Feedback"), Variant=w1819) -> (data=w1817:u8, error out=w1818:errorcluster)
            n727 = call <vilib>:"Flatten To JSON String.vi"("error in (no error)"=w1818, "Variant"=w1817) -> ("error out"=w1816:errorcluster, "JSON String"=w1815:string)  [unwired: 8 in]
            n728 = Format Into String(w1817) -> (resulting string=w1814:string)  [unwired: 3 in, 1 out]
          }
          frame "M2 Feedback" {
            n729 = Variant To Data(error in=w1829, type=u8 0 ("Network Data Down.M2 Commands.Feedback"), Variant=w1827) -> (data=w1825:u8, error out=w1826:errorcluster)
            n730 = call <vilib>:"Flatten To JSON String.vi"("error in (no error)"=w1826, "Variant"=w1825) -> ("error out"=w1823:errorcluster, "JSON String"=w1824:string)  [unwired: 8 in]
            n731 = Format Into String(w1825) -> (resulting string=w1822:string)  [unwired: 3 in, 1 out]
          }
          frame "M1 Package" {
            n732 = Variant To Data(error in=w1837, type=u16 0 ("Network Data Down.M1 Commands.Package"), Variant=w1835) -> (data=w1833:u16, error out=w1834:errorcluster)
            n733 = call <vilib>:"Flatten To JSON String.vi"("error in (no error)"=w1834, "Variant"=w1833) -> ("error out"=w1832:errorcluster, "JSON String"=w1831:string)  [unwired: 8 in]
            n734 = Format Into String(w1833) -> (resulting string=w1830:string)  [unwired: 3 in, 1 out]
          }
          frame "M2 Package" {
            n735 = Variant To Data(error in=w1845, type=u16 0 ("Network Data Down.M2 Commands.Package"), Variant=w1843) -> (data=w1841:u16, error out=w1842:errorcluster)
            n736 = call <vilib>:"Flatten To JSON String.vi"("error in (no error)"=w1842, "Variant"=w1841) -> ("error out"=w1840:errorcluster, "JSON String"=w1839:string)  [unwired: 8 in]
            n737 = Format Into String(w1841) -> (resulting string=w1838:string)  [unwired: 3 in, 1 out]
          }
          frame "M1 Enable" {
            n738 = Variant To Data(error in=w1852, type=TRUE, Variant=w1850) -> (data=w1848:bool, error out=w1846:errorcluster)
            n739 = call <vilib>:"Flatten To JSON String.vi"("error in (no error)"=w1846, "Variant"=w1848) -> ("error out"=w1851:errorcluster, "JSON String"=w1849:string)  [unwired: 8 in]
          }
          frame "M2 Enable" {
            n740 = Variant To Data(error in=w1859, type=TRUE, Variant=w1858) -> (data=w1855:bool, error out=w1853:errorcluster)
            n741 = call <vilib>:"Flatten To JSON String.vi"("error in (no error)"=w1853, "Variant"=w1855) -> ("error out"=w1857:errorcluster, "JSON String"=w1856:string)  [unwired: 8 in]
          }
          frame "Update Config" {
            w1865 = T32 {"Packages"={"DUT Force lbf"={" 0"=0, " 1"=0, " 2"=0, "3"=0, "4"=0, "5"=0, " 6"=0, "7"=0, "8"=0, "9"=0}, "DUT Names"={"0"="", "1"="", "2"="", "3"="", "4"="", "5"="", "6"="", "7"="", "8"="", "9"=""}}, "Heater PID"={"P"=0.0, "I"=0.0, "D"=0.0}, "Piston Settings"={"Forces Slope"=0.0, "Forces Intercept"=0.0, "Transition Force"=0.0, "Up Force"=0.0, "Diameter (mm)"=0.0, "Delay (ms)"=0.0, "Pressure Ramp Delay (ms)"=0.0}, "Safe Temps"={"Minimum"=17, "Enabled"=TRUE, "Maximum"=95}, "System Settings"={"Number of Heads"=0, "60Hz Power"=TRUE, "FTC200"=TRUE, "AutoStartup"=FALSE, "Purge"=TRUE, "Sensors"=TRUE, "HandClamp"=TRUE, "ATE"=TRUE, "Benchtop"=TRUE, "Production"=TRUE, "Refrigerant"=0, "Handler"=TRUE, "Shuttle"=TRUE, "220V"=FALSE, "Cascade"=FALSE, "Suction Sensor"=0, "Discharge Sensor"=0}, "Stepper Settings "={"Microstepping"=0, "Velocity"=8}, "Set Point Range"={"Max"=0.0, "Min"=0.0}, "Pedestal Check DeltaT"=0.0, "Ramp Delta T"=0.0, "Ramp-SS Threshold"=0.0, "SS Tolerance"=0.0, "EEV PID"={"Ramp Up Target"=0.0, "Ramp Down Target"=0.0, "Steady State Target"=0.0, "Output"={"Max"=0.0, "Min"=0.0}, "EBB and Flow Temp TH"=0.0, "Cryomode EEV Max"=0.0, "Valve minimum opening "=0.0, "Ramp Up EEV Steps"=0.0, "Ramp Down EEV Steps"=0.0, "SS EEV Steps Reset"=0.0, "EBB and Flow Tol"=0.0, "Gains"={"P"=0.0, "I"=0.0, "D"=0.0}, "Dissabled Target"=0.0, "CryoMode Gains"={"P"=0.0, "I"=0.0, "D"=0.0}, "M1 SuperHeat Setpoint"=0.0, "M2 Gains"={"P"=0.0, "I"=0.0, "D"=0.0}, "Flow Curve"=0}, "Sleep Timeout"=0.0, "Bypass Values"={"Bypass Valve"=TRUE, "Flow Curve"=0, "Output"={"Max"=0, "Min"=0}, "Feedback"=0, "Cyth Bypass"=TRUE, "PID"={"P"=0.0, "I"=0.0, "D"=0.0}, "Pressure setpoint"=0, "Cryo Temp"=0, "Superheat Setpoint"=0, "Cryo Setpoint"=0}, "Default Temp"=0.0, "InTEC"={"Enabled"=FALSE, "IP"="192.168.1.100", "Port"=5000}, "M1 TSD"={"Gain"=0.0, "Offset"=0.0, "V Offset "=0.0}, "M2 TSD"={"Gain"=0.0, "Offset"=0.0, "V Offset "=0.0}, "M1 T-Case Calibration"={"Gain"=0.0, "Offset"=0.0}, "M2 T-Case Calibration"={"Gain"=0.0, "Offset"=0.0}, "Heater PID TSD"={"P"=0.0, "I"=0.0, "D"=0.0}, "M2 Heater PID"={"P"=0.0, "I"=0.0, "D"=0.0}}  # Config Data
            n742 = Variant To Data(error in=w1866, type=w1865, Variant=w1864) -> (data=w1863:T32, error out=w1862:errorcluster)
            n743 = call <vilib>:"Flatten To JSON String.vi"("error in (no error)"=w1862, "Variant"=w1863) -> ("error out"=w1861:errorcluster, "JSON String"=w1860:string)  [unwired: 8 in]
          }
          frame "Reboot RT" {
            n744 = Variant To Data(error in=w1873, type=TRUE ("Stop RT"), Variant=w1872) -> (data=w1869:bool, error out=w1867:errorcluster)
            n745 = call <vilib>:"Flatten To JSON String.vi"("error in (no error)"=w1867, "Variant"=w1869) -> ("error out"=w1871:errorcluster, "JSON String"=w1870:string)  [unwired: 8 in]
          }
          frame "Stop RT" {
            n746 = Variant To Data(error in=w1880, type=TRUE ("STop RT"), Variant=w1879) -> (data=w1874:bool, error out=w1877:errorcluster)
            n747 = call <vilib>:"Flatten To JSON String.vi"("error in (no error)"=w1877, "Variant"=w1874) -> ("error out"=w1876:errorcluster, "JSON String"=w1875:string)  [unwired: 8 in]
          }
        }
        n748 = Unbundle By Name(w1772) -> ("TCP connection info"=w1771:T27)
        n749 = call-poly <vilib>:"Write Message.vi"("error in"=w1763, "data"=w1767, "name"=w1766, "connection info in"=w1771) -> ("error out"=w1773:errorcluster)  [unwired: 1 in, 6 out]
      }
      frame "TCP:Close Connection" {
        w1883 = 66 items=["No Error", "Argument Error", "Memory Full", "Out of Zone", "End of File", "File Already Open", "Generic File IO Error", "File Not Found", "File Permission Error", "Disk Full", "Duplicate Path", "Too Many Files Open", "Not Enabled", "Resource File Not Found", "Cannot Add Resource", "Resource Not Found", "Image Not Found", "Image Memory Error", "Pen Does Not Exist", "Config Bad Type", "Config Token Not Found", "Config Parse Error", "Config Memory Error", "Bad External Code Format", "Bad External Code Offset", "External Code Not Present", "Null Window", "Destroy Window Mixup", "Null Menu", "Print Aborted", "Bad Print Record", "Print Driver Error", "Windows Error During Print", "Memory Error During Print", "Print Dialog Error", "Generic Print Error", "Invalid Device Refnum", "Device Not Found", "Device Parameter Error", "Device Unit Error", "Can't Open Device", "Device Call Aborted", "Generic Error", "Cancelled By User", "Object ID Too Low", "Object ID Too High", "Object Not In Heap", "Unknown Heap", "Bad DefProc ID", "DefProc Not In Table", "Message Out Of Range", "Null Method", "Unknown Message", "Manager Call Not Supported", "Bad address", "Connection In progress", "Connection timed out", "Connection is already in progress", "Network attribute not supported", "Network error", "Address in use", "System out of memory", "Connection aborted", "Connection refused", "Connection is not connected", "Connection is already connected", "Connection closed", "Initialize error (interapplication manager)", "Bad occurrence", "Wait on unbound occurrence handler", "Occurrence queue overflow", "Bad path", "Semaphore not signaled", "Unrecognized type (interapplication manager)"] ("1st Error to Convert")
        n750 = Unbundle By Name(w1887) -> ("TCP connection info"=w1886:T27)
        n751 = call-poly <vilib>:"Get Connection Reference.vi"("error in"=w1888, "connection info in"=w1886) -> ("error out"=w1889:errorcluster, "connection ID out"=w1890:refnum<k5>)  [unwired: 8 out]
        n752 = TCP Close Connection(connection ID=w1890, error in (no error)=w1889) -> (error out=w1882:errorcluster)  [unwired: 2 out]
        n753 = call <vilib>:"Error to Warning.vi"("1st Error to Convert"=w1883, "error in"=w1882) -> ("warning out"=w1881:errorcluster)  [unwired: 3 in, 10 out]
      }
      frame "----------Database -----------" {
      }
      frame "DB:Login" {
        n754 = Variant To Data(error in=w1908, type=T38."Supervisor" ("f"), Variant=w1907) -> (data=w1894:T38, error out=w1896:errorcluster)
        n755 = case shown="\"Engineer\"" w1894 {
          tunnel: [i32[] [0, 1, 2, 3, 4, 5] ("Page array") i32[] [0, 1, 2, 3] ("Page array") i32[] [0, 1, 2] ("Page array") i32[] [0, 1, 2] ("Page array")] -> w1898
          tunnel: ["Supervisor" ("Command") "Engineer" ("Command") "Operator" ("Command") "Guest" ("Command")] -> w1897
          tunnel: w1896 -> [w1911 w1915 w1919 w1923]
          tunnel: [w1911 w1915 w1919 w1923] -> w1895
          tunnel: [TRUE ("Visible") TRUE ("Visible") FALSE ("Visible") FALSE ("Visible")] -> w1893
          frame "Supervisor" {
          }
          frame "Engineer" {
          }
          frame "Operator", Default {
          }
          frame "Guest" {
          }
        }
        n756 = To Variant(anything=w1898) -> (Variant=w1903:variant)
        n757 = call "Messaging EnQ Single.vi"("Command"="UI:Enable Tabs", "Data"=w1903, "error in (no error)"=w1895) -> ("error out"=w1901:errorcluster)  [unwired: 8 in]
        n758 = To Variant(anything=w1894) -> (Variant=w1899:variant)
        n759 = call "Messaging EnQ Single.vi"("Command"="UI:Enable Controls", "Data"=w1899, "error in (no error)"=w1901) -> ("error out"=w1909:errorcluster)  [unwired: 8 in]
        n760 = Bundle By Name(cluster=w1905, "User"=w1894) -> (w1904:T24)
      }
      frame "DB:Event Logger" {
        # "5.12.2021 Johathan asked me to remove  saving the event logging to file"
        n761 = Variant To Data(error in=w1938, type=T20 {"Name"="", "Time Stamp"=timestamp(0 s since 1904-01-01), "Code"=0, "Source"="", "Value"="", "Boolean"=FALSE, "Description"="", "Error"=FALSE, "Warning"=FALSE, " Fault"=FALSE} ("Event"), Variant=w1937) -> (data=w1928:T20, error out=w1929:errorcluster)
        n762 = Unbundle By Name(w1939) -> ("Event Log"=w1940:T20[])
        n763 = call "Event Logger.vi"("Error In"=w1929, "Event"=w1928) -> ("Error Out"=w1926:errorcluster, "Event out"=w1927:T20)  [unwired: 8 in]
        n764 = Insert Into Array(array=w1940, new element=w1927) -> (w1935:T20[])  [unwired: 1 in]
        "GUI Events" <- w1935
        n765 = Bundle By Name(cluster=w1939, "Event Log"=w1935) -> (w1934:T24)
        n766 = Unbundle By Name(w1927) -> ("Description"=w1931:string)
        n767 = Unbundle By Name(w1934) -> ("Core.VI Name"=w1932:string)
        n768 = disable-structure shown="Enabled" {
          disable-tunnel: [w1946 w1947] -> w1933
          disable-tunnel: w1932 -> [w1944 _]
          disable-tunnel: w1931 -> [w1943 _]
          disable-tunnel: w1930 -> [w1942 _]
          disable-tunnel: w1926 -> [w1941 w1947]
          frame Disabled {
            n769 = call "Save Log FGV.vi"("Case"=w1942, "State"=Save_Log_State."Write", "Error In"=w1941, "Descripition"=w1943, "VI Name"=w1944) -> ("Error Out"=w1946:errorcluster)  [unwired: 6 in]
          }
          frame Enabled {
          }
        }
      }
      frame "----------- Application---------" {
      }
      frame "APP:Update Config" {
        # "Confirm Config Data modified"
        n770 = Unbundle By Name(w1958) -> ("Dataset.Config Data"=w1955:T32)
        n771 = Index Array(array=w1957) -> (element=w1956:string)  [unwired: 1 in]
        n772 = case shown="\"Package\"" w1956 {
          tunnel: w1955 -> [w1964 w1968]
          tunnel: [w1960 w1971] -> w1954
          tunnel: [w1961 w1970] -> w1953
          tunnel: [w1962 w1969] -> w1952
          tunnel: w1951 -> [w1966 w1967]
          frame "Package" {
            n773 = Unbundle By Name(w1964) -> ("Packages"=w1965:T46)
            n774 = call "Modified Packages.vi"("error in"=w1966, "Pagckages in"=w1965) -> ("error out"=w1960:errorcluster, "Cancel?"=w1961:bool, "Modified Packages"=w1963:T47)  [unwired: 6 in]
            n775 = Bundle By Name(cluster=w1964, "Packages"=w1963) -> (w1962:T32)
          }
          frame "Configure", Default {
            n776 = call "Update Config Data.vi"("error in (no error)"=w1967, "Config Data Current"=w1968) -> ("error out"=w1971:errorcluster, "Canceled"=w1970:bool, "Modified Config Data"=w1969:T32)  [unwired: 7 in]
          }
        }
        n777 = case shown="False" w1953 {
          tunnel: [w1974 w1976] -> w1959
          tunnel: w1954 -> [w1975 w1976]
          tunnel: w1952 -> [w1973 _]
          tunnel: "NS:Write>>Update Config" ("Command(s)") -> [w1972 _]
          frame False {
            n778 = call "Messaging EnQ Single.vi"("Command"=w1972, "Data"=w1973, "error in (no error)"=w1975) -> ("error out"=w1974:errorcluster)  [unwired: 8 in]
          }
          frame True {
          }
        }
      }
      frame "APP:Load TDMS" {
        n779 = Unbundle By Name(w1995) -> ("IP Address"=w1991:string)
        n780 = Format Into String(format string="%s/files", initial string="http://" ("host uri prefix"), w1991) -> (resulting string=w1980:string)  [unwired: 1 in, 1 out]
        n781 = call "WebDAV FGV.vi"("WebDAV States"=WebDAV_states."Open Sess", "error in (no error)"=w1979, "host uri prefix"=w1980) -> ("error out"=w1987:errorcluster)  [unwired: 6 in, 2 out]
        n782 = call "WebDAV FGV.vi"("WebDAV States"=WebDAV_states."Refresh Dir", "error in (no error)"=w1987, "relative uri"="/u/") -> ("error out"=w1978:errorcluster, "file list"=w1983:T48[])  [unwired: 6 in, 1 out]
        n783 = Reverse 1D Array(array=w1983) -> (reversed array=w1982:T48[])
        n784 = for {
          tunnel: w1982 -> [w2002] mode=indexing
          tunnel: [w1997] -> w1986 mode=indexing if=w1996
          tunnel: [w2000] -> w1985 mode=indexing if=w1996
          tunnel: [w1998] -> w1984 mode=indexing if=w1996
          n785 = Unbundle By Name(w2002) -> ("display name"=w1997:string, "size"=w2001:u64, "last modification"=w1999:timestamp)
          n786 = String To Path(string=w1997) -> (path=w2005:path)
          n787 = Format Date/Time String(seconds (now)=w1999) -> (date/time string=w1998:string)  [unwired: 2 in]
          n788 = call <vilib>:"Get File Extension.vi"("file"=w2005) -> ("lowercase file extension"=w2004:string)  [unwired: 6 in, 4 out]
          n789 = Number To Decimal String(number=w2001) -> (decimal integer string=w2000:string)  [unwired: 1 in]
          n790 = Equal?(x=w2004, y="tdms") -> (x = y?=w1996:bool)
        }
        n791 = Build Array(w1986, w1985, w1984) -> (w1981:string[][])
        n792 = Transpose 2D Array(2D array=w1981) -> (transposed array=w1977:string[][])
        n793 = call "Dialog TDMS Datalog.vi"("Error In"=w1978, "Logdata"=w1977) -> ("Error Out"=w1994:errorcluster)  [unwired: 9 in]
      }
      frame "Update Variables" {
        w2010 = TRUE  # Reboot RT
        n794 = Variant To Data(error in=w2012, type=w2010, Variant=w2007) -> (data=w2006:bool, error out=w2011:errorcluster)
        n795 = Bundle By Name(cluster=w2009, "Reboot"=w2006) -> (w2008:T24)
      }
    }
    n796 = call "Add Event.vi"("Log?"=w19, "Name"=w20, "Value"=w16, "Error In"=w22, "Description"=w17, "Boolean"=w18) -> ("Error Out"=w21:errorcluster)  [unwired: 5 in]
  }
  n797 = while {
    shift-right: [w2016] -> w13
    shift-left: w10 -> [w2017]
    stop <- w2018 stop-if-true
    # "Controller"
    n798 = local read "Login TO"() -> (w2013:i32)
    n799 = Multiply(x=60000, y=w2013) -> (x*y=w2014:i32)
    n800 = event shown="[2] \"Power On-Off\", \"Shutdown\", \"Reboot RT\", \"M1 Commands Panel.M1 Enable\", \"M2 Commands Panel.M2 Enable\": Value Change" {
      selector: _ -> [_ _ _ _ _ _ _ _]
      dyn-events: _ -> [_ _ _ _ _ _ _ _]
      timeout: w2014 -> [_ _ _ _ _ _ _ _]
      tunnel: [w2023 _ _ _ _ _ _ w2477] -> w2018
      tunnel: [w2022 w2027 w2048 w2169 w2241 w2415 w2433 w2480] -> w2016
      tunnel: w2017 -> [w2021 w2031 w2039 w2170 w2240 w2416 w2434 w2481]
      event Timeout {
        # "Logout when not received any event for 10 min"
        n801 = event-data() -> ()  [unwired: 1 in, 1 out]
        n802 = property on="Login" class="Bool (strict)"(error in=w2021, "Value"=FALSE) -> (error out=w2020:errorcluster)  [unwired: 1 in, 1 out]
        n803 = call "Messaging AE.vi"("Error In"=w2020) -> ("Error Out"=w2022:errorcluster, "queue out"=w2024:refnum<queue>)  [unwired: 9 in]
        n804 = Not A Number/Path/Refnum?(number/path/refnum=w2024) -> (NaN/Path/Refnum?=w2023:bool)
      }
      event "M1 Set Temp", "M1 Package", "M1 Feedback", "M1 Power Drive Control", "M2 Set Temp", "M2 Package", "M2 Feedback", "M2 Power Drive Control": Value Change {
        n805 = event-data() -> ("CtlRef"=w2032:refnum<vi>, "NewVal"=w2025:variant)  [unwired: 1 in]
        n806 = property class="Ctl"(reference=w2032) -> ("Caption.Text"=w2026:string)  [unwired: 1 in, 2 out]
        n807 = Concatenate Strings("NS:Write>>" ("Command"), w2026) -> (w2030:string)
        n808 = call "Messaging EnQ Single.vi"("Command"=w2030, "Data"=w2025, "error in (no error)"=w2031) -> ("error out"=w2028:errorcluster)  [unwired: 8 in]
        n809 = disable-structure shown="Disabled" {
          disable-tunnel: w2028 -> [w2038 _]
          disable-tunnel: [w2037 _] -> w2027
          disable-tunnel: w2026 -> [w2035 _]
          disable-tunnel: w2025 -> [w2033 _]
          frame Disabled {
            n810 = Concatenate Strings("TCP:Write>>" ("Command"), w2035) -> (w2034:string)
            n811 = call "Messaging EnQ Single.vi"("Command"=w2034, "Data"=w2033, "error in (no error)"=w2038) -> ("error out"=w2037:errorcluster)  [unwired: 8 in]
          }
          frame Enabled {
          }
        }
      }
      event "Power On-Off", "Shutdown", "Reboot RT", "M1 Commands Panel.M1 Enable", "M2 Commands Panel.M2 Enable": Value Change {
        n812 = event-data() -> ("CtlRef"=w2053:refnum<vi>, "NewVal"=w2051:bool)  [unwired: 1 in]
        n813 = property class="Bool"(reference=w2053) -> ("Caption.Text"=w2042:string)  [unwired: 1 in, 2 out]
        n814 = Concatenate Strings("TCP:Write>>" ("Command"), w2042) -> (w2041:string)
        n815 = property on="Comp" class="Bool (strict)"() -> ("Value"=w2052:bool)  [unwired: 2 in, 2 out]
        n816 = Concatenate Strings("NS:Write>>" ("Command"), w2042) -> (w2040:string)
        n817 = case shown="\"Reboot RT\"" w2042 {
          tunnel: w2052 -> [_ _ w2097 w2127 w2143]
          tunnel: [w2058 w2066 w2099 w2124 w2141] -> w2047
          tunnel: [_ w2067 w2100 w2134 w2145] -> w2046
          tunnel: w2051 -> [_ _ w2098 _ w2138]
          tunnel: "Are you sure you want to " ("message") -> [_ w2065 _ w2129 w2144]
          tunnel: [w2058 w2061 w2096 w2125 w2142] -> w2045
          tunnel: w2041 -> [_ w2059 w2095 w2123 w2140]
          tunnel: w2040 -> [_ w2060 w2094 w2122 w2139]
          frame Default {
            w2058 = ""
          }
          frame "Power On-Off" {
            n818 = local read "Play/Pause"() -> (w2068:bool)
            n819 = Format Into String(format string="%s", initial string=w2065, "pause?" ("message")) -> (resulting string=w2062:string)  [unwired: 1 in, 1 out]
            n820 = case shown="False" w2068 {
              tunnel: w2062 -> [_ w2090]
              tunnel: [w2071 w2085] -> w2070
              tunnel: [w2075 w2087] -> w2066
              tunnel: w2060 -> [w2072 w2088]
              tunnel: w2059 -> [w2073 w2089]
              tunnel: [w2076 w2086] -> w2061
              frame False {
                n821 = property on="M2 Enable" class="Bool (strict)"() -> ("Value"=w2080:bool)  [unwired: 2 in, 2 out]
                n822 = property on="M1 Enable" class="Bool (strict)"() -> ("Value"=w2077:bool)  [unwired: 2 in, 2 out]
                n823 = Not(x=w2080) -> (.not. x?=w2079:bool)
                n824 = Not(x=w2077) -> (.not. x?=w2078:bool)
                n825 = And(x=w2078, y=w2079) -> (x .and. y?=w2071:bool)
                n826 = case shown="False" w2071 {
                  tunnel: [w2082 w2084] -> w2076
                  tunnel: [w2081 w2084] -> w2075
                  tunnel: "At least one head must be \nenabled to run on" ("message") -> [_ w2083]
                  tunnel: w2073 -> [w2082 _]
                  tunnel: w2072 -> [w2081 _]
                  frame False {
                  }
                  frame True {
                    w2084 = ""
                    n827 = One Button Dialog(message=w2083) -> ()  [unwired: 1 in, 1 out]
                  }
                }
              }
              frame True {
                n828 = Two Button Dialog(message=w2090) -> (T button?=w2085:bool)  [unwired: 2 in]
                n829 = case shown="False" w2085 {
                  tunnel: w2089 -> [_ w2092]
                  tunnel: w2088 -> [_ w2093]
                  tunnel: [w2091 w2093] -> w2087
                  tunnel: [w2091 w2092] -> w2086
                  frame False {
                    w2091 = ""
                  }
                  frame True {
                  }
                }
              }
            }
            n830 = Not(x=w2070) -> (.not. x?=w2069:bool)
            n831 = To Variant(anything=w2069) -> (Variant=w2067:variant)
          }
          frame "M1 Enable", "M2 Enable" {
            n832 = case shown="False" w2097 {
              tunnel: [w2102 w2111] -> w2099
              tunnel: [w2103 w2110] -> w2100
              tunnel: w2098 -> [w2104 w2105]
              tunnel: w2094 -> [w2102 w2108]
              tunnel: w2095 -> [w2101 w2107]
              tunnel: [w2101 w2106] -> w2096
              frame False {
                n833 = To Variant(anything=w2104) -> (Variant=w2103:variant)
              }
              frame True {
                n834 = property on="M2 Enable" class="Bool (strict)"() -> ("Value"=w2115:bool)  [unwired: 2 in, 2 out]
                n835 = property on="M1 Enable" class="Bool (strict)"() -> ("Value"=w2109:bool)  [unwired: 2 in, 2 out]
                n836 = Not(x=w2115) -> (.not. x?=w2114:bool)
                n837 = Not(x=w2109) -> (.not. x?=w2113:bool)
                n838 = And(x=w2113, y=w2114) -> (x .and. y?=w2112:bool)
                n839 = case shown="True" w2112 {
                  tunnel: w2105 -> [w2117 _]
                  tunnel: [w2118 w2120] -> w2111
                  tunnel: [w2119 _] -> w2110
                  tunnel: w2108 -> [w2118 _]
                  tunnel: w2107 -> [w2116 _]
                  tunnel: [w2116 w2120] -> w2106
                  frame False {
                    n840 = To Variant(anything=w2117) -> (Variant=w2119:variant)
                  }
                  frame True {
                    w2120 = ""
                    n841 = One Button Dialog(message="At least one head must be \nenabled to run on") -> ()  [unwired: 1 in, 1 out]
                  }
                }
              }
            }
          }
          frame "Stop RT" {
            n842 = Format Into String(format string="%s", initial string=w2129, "stop?" ("message")) -> (resulting string=w2133:string)  [unwired: 1 in, 1 out]
            n843 = Two Button Dialog(message=w2133) -> (T button?=w2128:bool)  [unwired: 2 in]
            n844 = Not(x=w2127) -> (.not. x?=w2130:bool)
            n845 = And(x=w2130, y=w2128) -> (x .and. y?=w2126:bool)
            n846 = case shown="False" w2126 {
              tunnel: w2123 -> [_ w2137]
              tunnel: w2122 -> [_ w2136]
              tunnel: [w2135 w2137] -> w2125
              tunnel: [w2135 w2136] -> w2124
              frame False {
                w2135 = ""
              }
              frame True {
              }
            }
            n847 = To Variant(anything=w2126) -> (Variant=w2134:variant)
          }
          frame "Reboot RT" {
            n848 = disable-structure shown="Enabled" {
              disable-tunnel: [w2158 w2164] -> w2145
              disable-tunnel: w2144 -> [w2157 _]
              disable-tunnel: w2143 -> [w2156 _]
              disable-tunnel: [w2155 _] -> w2142
              disable-tunnel: [w2154 "Update Variables" ("Command")] -> w2141
              disable-tunnel: w2140 -> [w2153 _]
              disable-tunnel: w2139 -> [w2152 _]
              disable-tunnel: w2138 -> [_ w2163]
              frame Disabled {
                n849 = Format Into String(format string="%s", initial string=w2157, " Reboot RT?" ("message")) -> (resulting string=w2151:string)  [unwired: 1 in, 1 out]
                n850 = Two Button Dialog(message=w2151) -> (T button?=w2147:bool)  [unwired: 2 in]
                n851 = Not(x=w2156) -> (.not. x?=w2148:bool)
                n852 = And(x=w2148, y=w2147) -> (x .and. y?=w2146:bool)
                n853 = case shown="True" w2146 {
                  tunnel: w2153 -> [_ w2161]
                  tunnel: w2152 -> [_ w2160]
                  tunnel: [w2159 w2161] -> w2155
                  tunnel: [w2159 w2160] -> w2154
                  frame False {
                    w2159 = ""
                  }
                  frame True {
                  }
                }
                n854 = To Variant(anything=w2146) -> (Variant=w2158:variant)
              }
              frame Enabled {
                n855 = To Variant(anything=w2163) -> (Variant=w2164:variant)
              }
            }
          }
        }
        n856 = call "Messaging EnQ Single.vi"("Command"=w2047, "Data"=w2046, "error in (no error)"=w2039) -> ("error out"=w2049:errorcluster)  [unwired: 8 in]
        n857 = disable-structure shown="Disabled" {
          disable-tunnel: w2049 -> [w2057 _]
          disable-tunnel: [w2056 _] -> w2048
          disable-tunnel: w2046 -> [w2055 _]
          disable-tunnel: w2045 -> [w2054 _]
          frame Disabled {
            n858 = call "Messaging EnQ Single.vi"("Command"=w2054, "Data"=w2055, "error in (no error)"=w2057) -> ("error out"=w2056:errorcluster)  [unwired: 8 in]
          }
          frame Enabled {
          }
        }
      }
      event "M1 Commands Panel.M1 TSD Feedback", "Cascade Compressor controls", "M2 Commands Panel.M2 TSD Feedback", "Manual Bypass Mode", "M1 Heater output", "M1 EEV Manual", "M2 Heater Output", "M2 EEV Manual": Value Change {
        n859 = event-data() -> ("CtlRef"=w2171:refnum<vi>, "NewVal"=w2168:variant)  [unwired: 1 in]
        n860 = property class="Ctl"(reference=w2171) -> ("Caption.Text"=w2165:string)  [unwired: 1 in, 2 out]
        n861 = case shown="\"M2 EEV Manual control\"" w2165 {
          selector: w2165 -> [w2173 _ _ _ _]
          tunnel: w2170 -> [w2177 w2180 w2194 w2208 w2222]
          tunnel: [w2176 w2179 w2193 w2207 w2221] -> w2169
          tunnel: w2168 -> [w2175 w2178 w2192 w2206 w2220]
          tunnel: "Manual Bypass Mode" -> [_ w2186 w2200 w2214 w2228]
          tunnel: "NSV:Write>>" ("DNL_Message") -> [w2174 w2183 w2197 w2211 w2225]
          frame Default {
            n862 = Concatenate Strings(w2174, w2173) -> (w2172:string)
            n863 = call "Messaging EnQ Single.vi"("Command"=w2172, "Data"=w2175, "error in (no error)"=w2177) -> ("error out"=w2176:errorcluster)  [unwired: 8 in]
          }
          frame "M2 EEV Manual control" {
            n864 = Index Array(array=w2186, index=3) -> (element=w2184:bool)
            n865 = Concatenate Strings(w2183, "M2 EEV Manual" ("format string")) -> (w2182:string)
            n866 = case shown="True" w2184 {
              tunnel: w2182 -> [_ w2191]
              tunnel: w2180 -> [w2187 w2190]
              tunnel: [w2187 w2189] -> w2179
              tunnel: w2178 -> [_ w2188]
              frame False {
              }
              frame True {
                n867 = call "Messaging EnQ Single.vi"("Command"=w2191, "Data"=w2188, "error in (no error)"=w2190) -> ("error out"=w2189:errorcluster)  [unwired: 8 in]
              }
            }
          }
          frame "M1 EEV Manual control" {
            n868 = Index Array(array=w2200, index=1) -> (element=w2198:bool)
            n869 = Concatenate Strings(w2197, "M1 EEV Manual" ("format string")) -> (w2196:string)
            n870 = case shown="True" w2198 {
              tunnel: w2196 -> [_ w2205]
              tunnel: w2194 -> [w2201 w2204]
              tunnel: [w2201 w2203] -> w2193
              tunnel: w2192 -> [_ w2202]
              frame False {
              }
              frame True {
                n871 = call "Messaging EnQ Single.vi"("Command"=w2205, "Data"=w2202, "error in (no error)"=w2204) -> ("error out"=w2203:errorcluster)  [unwired: 8 in]
              }
            }
          }
          frame "M1 Heater PWM" {
            n872 = Index Array(array=w2214, index=0) -> (element=w2212:bool)
            n873 = Concatenate Strings(w2211, "M1 Heater output" ("format string")) -> (w2210:string)
            n874 = case shown="True" w2212 {
              tunnel: w2210 -> [_ w2219]
              tunnel: w2208 -> [w2215 w2218]
              tunnel: [w2215 w2217] -> w2207
              tunnel: w2206 -> [_ w2216]
              frame False {
              }
              frame True {
                n875 = call "Messaging EnQ Single.vi"("Command"=w2219, "Data"=w2216, "error in (no error)"=w2218) -> ("error out"=w2217:errorcluster)  [unwired: 8 in]
              }
            }
          }
          frame "M2 Heater PWM" {
            n876 = Index Array(array=w2228, index=2) -> (element=w2226:bool)
            n877 = Concatenate Strings(w2225, "M2 Heater Output" ("format string")) -> (w2224:string)
            n878 = case shown="True" w2226 {
              tunnel: w2224 -> [_ w2233]
              tunnel: w2222 -> [w2229 w2232]
              tunnel: [w2229 w2231] -> w2221
              tunnel: w2220 -> [_ w2230]
              frame False {
              }
              frame True {
                n879 = call "Messaging EnQ Single.vi"("Command"=w2233, "Data"=w2230, "error in (no error)"=w2232) -> ("error out"=w2231:errorcluster)  [unwired: 8 in]
              }
            }
          }
        }
      }
      event "Net Cluster.Menu Ring", "Net Cluster.IP Override", "Net Cluster.System Ready": Value Change {
        n880 = event-data() -> ("OldVal"=w2234:variant, "NewVal"=w2238:variant, "CtlRef"=w2242:refnum<vi>)  [unwired: 1 in]
        n881 = Unbundle By Name("Net Cluster") -> ("Menu Ring"=w2237:u16, "Manual IP"=w2236:string)
        n882 = property class="Ctl"(reference=w2242) -> ("Label.Text"=w2239:string)  [unwired: 1 in, 2 out]
        n883 = case shown="\"Menu Ring\", Default" w2239 {
          tunnel: w2238 -> [_ _ w2397]
          tunnel: [w2243 w2384 w2399] -> w2241
          tunnel: w2240 -> [w2249 w2380 w2398]
          tunnel: w2237 -> [w2245 _ _]
          tunnel: w2236 -> [w2244 _ _]
          tunnel: w2234 -> [_ w2383 w2395]
          frame "IP Override" {
            n884 = property on="Menu Ring" class="Ring (strict)"() -> ("Strings []"=w2248:string[])  [unwired: 2 in, 2 out]
            n885 = for {
              tunnel: "\\b[0-9]+\\.[0-9]+\\.[0-9]+\\.[0-9]+" ("regular expression") -> [w2253]
              tunnel: w2248 -> [w2252] mode=indexing
              tunnel: [w2251] -> w2246 mode=indexing
              n886 = xnode ("Match Regular Expression")("input string"=w2252, "regular expression"=w2253) -> ("whole match"=w2251:string)  [unwired: 4 in, 4 out]
            }
            n887 = Empty String/Path?(string/path=w2244) -> (empty?=w2250:bool)
            n888 = case shown="False" w2250 {
              tunnel: w2245 -> [w2375 _]
              tunnel: w2244 -> [w2377 _]
              tunnel: [w2368 w2378] -> w2243
              tunnel: w2249 -> [w2369 w2378]
              tunnel: w2246 -> [w2370 _]
              frame False {
                n889 = Search 1D Array(1D array=w2370, element=w2377) -> (index of element=w2373:i32)  [unwired: 1 in]
                n890 = To Unsigned Word Integer(number=w2373) -> (unsigned 16bit integer=w2372:u16)
                n891 = Equal?(x=w2373, y=-1) -> (x = y?=w2376:bool)
                n892 = Select(t=w2375, s=w2376, f=w2372) -> (s? t:f=w2371:u16)
                n893 = property on="Menu Ring" class="Ring (strict)"(error in=w2369, "Val(Sgnl)"=w2371) -> (error out=w2368:errorcluster)  [unwired: 1 in, 1 out]
              }
              frame True {
              }
            }
          }
          frame "System Ready" {
            n894 = Variant To Data(error in=w2380, type=TRUE ("System"), Variant=w2383) -> (data=w2381:bool, error out=w2379:errorcluster)
            n895 = case shown="True" w2381 {
              tunnel: w2379 -> [w2385 w2387]
              tunnel: [w2385 w2386] -> w2384
              frame False {
              }
              frame True {
                n896 = Two Button Dialog(message="Are you sure you want to disconnect?") -> (T button?=w2388:bool)  [unwired: 2 in]
                n897 = case shown="True" w2388 {
                  tunnel: w2387 -> [w2390 w2392]
                  tunnel: [w2390 w2391] -> w2386
                  frame False {
                  }
                  frame True {
                    n898 = property on="Menu Ring" class="Ring (strict)"(error in=w2392, "Val(Sgnl)"=u16 100 ("Value (Signaling)")) -> (error out=w2391:errorcluster)  [unwired: 1 in, 1 out]
                  }
                }
              }
            }
          }
          frame "Menu Ring", Default {
            n899 = Two Button Dialog(message="Are you sure that you want \nto quit test and change the system?") -> (T button?=w2394:bool)  [unwired: 2 in]
            n900 = case shown="False" w2394 {
              tunnel: [w2400 w2407] -> w2399
              tunnel: w2398 -> [w2403 w2406]
              tunnel: w2397 -> [_ w2405]
              tunnel: w2395 -> [w2402 _]
              frame False {
                n901 = Variant To Data(error in=w2403, type=u16 0 ("Value"), Variant=w2402) -> (data=w2401:u16, error out=w2400:errorcluster)
                n902 = property on="Menu Ring" class="Ring (strict)"("Value"=w2401) -> ()  [unwired: 2 in, 2 out]
              }
              frame True {
                n903 = call "Messaging EnQ Single.vi"("Command"="MACRO:NS Update", "Data"=w2405, "error in (no error)"=w2406) -> ("error out"=w2407:errorcluster)  [unwired: 8 in]
              }
            }
          }
        }
      }
      event "Configure", "Package", "Graph Temp Unit", "Net Cluster.Refresh": Value Change {
        n904 = event-data() -> ("CtlRef"=w2414:refnum<vi>, "NewVal"=w2410:bool)  [unwired: 1 in]
        n905 = property class="Bool"(reference=w2414) -> ("Label.Text"=w2413:string)  [unwired: 1 in, 2 out]
        n906 = case shown="\"Graph Temp Unit\"" w2413 {
          selector: w2413 -> [_ _ w2426 w2429]
          tunnel: ["NS:Detect Systems" ("Command(s)") "UI:Refresh Graph" ("Command") w2425 w2428] -> w2412
          tunnel: [TRUE ("@Front?") _ _ _] -> w2411
          tunnel: w2410 -> [_ w2423 _ _]
          tunnel: [_ w2419 _ _] -> w2409
          frame "Refresh", Default {
          }
          frame "Graph Temp Unit" {
            n907 = Select(t="°C" ("Command"), s=w2423, f="°F" ("Command")) -> (s? t:f=w2420:string)
            n908 = To Variant(anything=w2420) -> (Variant=w2419:variant)
          }
          frame "Configure" {
            n909 = Concatenate Strings("APP:Update Config>>" ("Command(s)"), w2426) -> (w2425:string)
          }
          frame "Package" {
            n910 = Concatenate Strings("APP:Update Config>>" ("Command(s)"), w2429) -> (w2428:string)
          }
        }
        n911 = call "Messaging EnQ Single.vi"("Command"=w2412, "@Front?"=w2411, "Data"=w2409, "error in (no error)"=w2416) -> ("error out"=w2415:errorcluster)  [unwired: 7 in]
      }
      event "Datalog", "Login TO", "Login": Value Change {
        n912 = event-data() -> ("OldVal"=w2431:variant, "CtlRef"=w2436:refnum<vi>, "NewVal"=w2432:variant)  [unwired: 1 in]
        n913 = property class="Ctl"(reference=w2436) -> ("Label.Text"=w2435:string)  [unwired: 1 in, 2 out]
        n914 = case shown="\"Login\"" w2435 {
          tunnel: w2434 -> [w2437 w2447 w2450 w2452]
          tunnel: [w2437 w2444 w2448 w2458] -> w2433
          tunnel: w2432 -> [_ w2446 _ w2455]
          tunnel: w2431 -> [_ w2443 _ _]
          frame Default {
          }
          frame "Login TO" {
            n915 = Variant To Data(type=0 ("Login TO"), Variant=w2443) -> (data=w2441:i32)  [unwired: 1 in, 1 out]
            n916 = Variant To Data(error in=w2447, type=0 ("Login TO"), Variant=w2446) -> (data=w2439:i32, error out=w2444:errorcluster)
            n917 = Equal To 0?(x=w2439) -> (x = 0?=w2438:bool)
            n918 = Select(t=w2441, s=w2438, f=w2439) -> (s? t:f=w2440:i32)
            n919 = property on="Login TO" class="DigNum (strict)"("Value"=w2440) -> ()  [unwired: 2 in, 2 out]
          }
          frame "Datalog" {
            n920 = call "Messaging EnQ Single.vi"("Command"="APP:Load TDMS", "error in (no error)"=w2450) -> ("error out"=w2448:errorcluster)  [unwired: 9 in]
          }
          frame "Login" {
            n921 = Variant To Data(error in=w2452, type=FALSE, Variant=w2455) -> (data=w2453:bool, error out=w2451:errorcluster)
            n922 = case shown="True" w2453 {
              tunnel: w2451 -> [w2461 w2468]
              tunnel: [w2461 w2463] -> w2459
              tunnel: [T38."Operator" ("f") w2464] -> w2460
              frame False {
              }
              frame True {
                n923 = call "Login.vi"("error in"=w2468) -> ("error out"=w2467:errorcluster, "OK?"=w2465:bool, "Level"=w2466:T38)  [unwired: 7 in]
                n924 = case shown="False" w2465 {
                  tunnel: w2467 -> [w2471 w2473]
                  tunnel: w2466 -> [_ w2474]
                  tunnel: [T38."Operator" ("f") w2474] -> w2464
                  tunnel: [w2469 w2473] -> w2463
                  frame False {
                    n925 = property on="Login" class="Bool (strict)"(error in=w2471, "Value"=FALSE ("Login")) -> (error out=w2469:errorcluster)  [unwired: 1 in, 1 out]
                  }
                  frame True {
                  }
                }
              }
            }
            n926 = To Variant(anything=w2460) -> (Variant=w2457:variant)
            n927 = call "Messaging EnQ Single.vi"("Command"="DB:Login", "Data"=w2457, "error in (no error)"=w2459) -> ("error out"=w2458:errorcluster)  [unwired: 8 in]
          }
        }
      }
      event Panel Close? {
        n928 = event-data() -> ()  [unwired: 1 in, 1 out]
        n929 = Two Button Dialog(message="Are you sure you want to Stop the Application?") -> (T button?=w2478:bool)  [unwired: 2 in]
        n930 = case shown="True" w2478 {
          tunnel: w2481 -> [w2484 w2489]
          tunnel: [w2484 w2488] -> w2480
          tunnel: [FALSE ("Discard?") TRUE ("Discard?")] -> w2477
          tunnel: "MACRO:Shutdown" ("Command") -> [_ w2487]
          tunnel: [TRUE ("Discard?") TRUE ("Discard?")] -> w2475
          frame False {
          }
          frame True {
            n931 = call "Messaging EnQ Single.vi"("Command"=w2487, "@Front?"=TRUE, "error in (no error)"=w2489) -> ("error out"=w2488:errorcluster)  [unwired: 8 in]
          }
        }
        n932 = event-data("Discard?"=w2475) -> ()  [unwired: 1 in, 1 out]
      }
    }
  }
  n933 = Merge Errors(w13, w12) -> (→"Error Out":errorcluster)
